vi "MainProgram.vi"(0 "DAQmx Task":refnum<k21>, 1 "BNC Port":refnum<visa-resource-name>, 2 "SRS Port":refnum<visa-resource-name>, 3 "Energy Meter  port":refnum<visa-resource-name>, 4 "SDG II port":refnum<visa-resource-name>, 5 "Mode":T18=enum."GenericTOF", 6 "Micos Port":refnum<visa-resource-name>="COM3", 7 "CommPort (ESP300)":refnum<visa-resource-name>="COM7", 8 "Serial Config (Micos)":T15={"Baud Rate"=115200, "Parity"=0, "Data Bits"=8, "Stop Bits"=10, "Flow Control"=0} {"Flow Control" items=["None", "XON/XOFF", "RTS/CTS", "XON/XOFF & RTS/CTS", "DTR/DSR", "XON/XOFF & DTR/DSR"]; "Stop Bits" items=["1.0"=10, "1.5"=15, "2.0"=20]; "Data Bits" items=["7"=7, "8"=8]; "Parity" items=["None", "Odd", "Even", "Mark", "Space"]; "Baud Rate" items=["300"=300, "600"=600, "1200"=1200, "2400"=2400, "4800"=4800, "9600"=9600, "19200"=19200]}, 9 "Serial Config (ESP300)":T15={"Baud Rate"=19200, "Parity"=0, "Data Bits"=8, "Stop Bits"=10, "Flow Control"=2} {"Flow Control" items=["None", "XON/XOFF", "RTS/CTS", "XON/XOFF & RTS/CTS", "DTR/DSR", "XON/XOFF & DTR/DSR"]; "Stop Bits" items=["1.0"=10, "1.5"=15, "2.0"=20]; "Data Bits" items=["7"=7, "8"=8]; "Parity" items=["None", "Odd", "Even", "Mark", "Space"]; "Baud Rate" items=["300"=300, "600"=600, "1200"=1200, "2400"=2400, "4800"=4800, "9600"=9600, "19200"=19200]}, 10 "#Axis (Micos)":i32=3, 11 "#Axis (ESP300)":i32=3, 12 "Simulation (Micos)":bool=TRUE, 13 "Simulation (ESP300)":bool=TRUE, 14 "MainDAQ_Selector":T16=enum."FakeSignal(Emulator)" caption="Restart Required", 15 "Laser Control Method":T17=enum."SDG_II" caption="Restart Required") -> ()   [LabVIEW 2013]
uses:
  Files/Signal_Segment.ctl
  ControlDef/ProcessingMode.ctl
  ControlDef/Average#.ctl
  ProcessMethods/Binning/BinType.ctl
  ControlDef/MainDAQ_Selector.ctl
  ControlDef/LaserCtrl_Method.ctl
  ControlDef/SpecLengthSelector.ctl
  ControlDef/SampleRateSelector.ctl
  ControlDef/DAQRangeSelector.ctl
  <instrlib>/DG535/Command/DG535_TriggerMode.ctl
  ControlDef/StepWidthSelector.ctl
  ControlDef/Files_Format.ctl
  <instrlib>/DG535/DG535_Configs.ctl
  <instrlib>/DG535/Command/Set Trigger.ctl
  <instrlib>/DG535/Command/Set Delay.ctl
  <instrlib>/DG535/Command/DG535_Channel.ctl
  <instrlib>/DG535/Command/Set Output.ctl
  <instrlib>/DG535/Command/DG535_Output.ctl
  <instrlib>/AnalogDiscSDKLv/VIs/DWF_AnalogIn_Configurations.ctl
  <instrlib>/AnalogDiscSDKLv/VIs/DWF_AcqMode.ctl
  <instrlib>/AnalogDiscSDKLv/VIs/DWF_Filter.ctl
  <instrlib>/AnalogDiscSDKLv/VIs/DWF_TrigSrc.ctl
  <instrlib>/AnalogDiscSDKLv/VIs/DWF_TrigCond.ctl
  <instrlib>/AnalogDiscSDKLv/VIs/DWF_TrigType.ctl
  <instrlib>/GageLv_uic/VI/Gage_Configs.ctl
  ControlDef/InstruMode_Typedef.ctl
  Hardware/BNC(QuantumComposers)/BNC_Configs.ctl
  ControlDef/InstrumentSpecificControls/UIC-AToF/InitializationParams_BNC565_2Ch_AToF.ctl
  Hardware/BNC(QuantumComposers)/Command/Set C-Input.ctl
  Hardware/BNC(QuantumComposers)/Command/Set C-Mode.ctl
  Hardware/BNC(QuantumComposers)/Command/Set C-Output.ctl
  Hardware/BNC(QuantumComposers)/Command/Set C-Enable.ctl
  Hardware/GenericDAQ/VI/GenericDAQ_Configs.ctl
  <vilib>/Utility/error.llb/DialogType.ctl
  ControlDef/AllControlsRefs.ctl
  ControlDef/States-AToF.ctl
  Hardware/FemtoLaser(Legacy)/Laser_Status.ctl
  Files/SaveControlsRef.ctl
  Files/WriterState.ctl
  Hardware/DAQmx(Legacy)/DAQmx_Status.ctl
  Hardware/EPM2000(Legacy)/EPM2K_Status.ctl
  ProcessMethods/SignalAverager/ProcessParams.ctl
  ProcessMethods/SignalAverager/DAQParams.ctl
  ProcessMethods/SignalAverager/DisplayGraph.ctl
  <instrlib>/ESP300/Public/Data/ESP300_State.ctl
  Hardware/BNC(QuantumComposers)/BNC_States.ctl
  <instrlib>/DG535/Command/DG535_States.ctl
  <instrlib>/Micos_uic/Public/Data/Micos_Data.ctl
  ControlDef/QueueRefs.ctl
  <instrlib>/AnalogDiscSDKLv/VIs/DWF_CtrlQueue.ctl
  <instrlib>/AnalogDiscSDKLv/VIs/DWF_State.ctl
  ControlDef/Signal.ctl
  ProcessMethods/SignalAverager/ProcessStates.ctl
  <instrlib>/AnalogDiscSDKLv/VIs/DWF_Signal.ctl
  <instrlib>/AnalogDiscSDKLv/VIs/DWF_PrivateStats.ctl
  <instrlib>/AnalogDiscSDKLv/VIs/DWF_InstrumentStatus.ctl
  <instrlib>/GageLv_uic/VI/Gage_PrivateStats.ctl
  <instrlib>/GageLv_uic/VI/Gage_DAQStatus.ctl
  Apps/GenericUSBCamera/CameraEventTypedef.ctl
  Hardware/Joystick/Joystick_UserEvent.ctl
  Hardware/GenericDAQ/VI/GenericDAQ_PrivateStats.ctl
  Hardware/GenericDAQ/VI/GenericDAQ_Status.ctl
  <instrlib>/GageLv_uic/VI/SetSecondaryDataVIRef_Typedef.ctl
  Files/BinaryHeader.ctl
  Apps/BeamProfiling/BeamProfiling_Params.ctl
  Apps/InstruOptimizer/OptimizerParams.ctl
  Apps/ImagingMS/Imaging_Params.ctl
  <instrlib>/Micos_uic/Public/Data/Micos_State.ctl
  <vilib>/Analysis/baseanly.llb/A x Vector.vi
  ControlDef/QuitProg.vi
  <instrlib>/Micos_uic/Public/Position_Micos.vi
  <instrlib>/ESP300/Public/Position_ESP300.vi
  ControlDef/MiscParams.vi
  ControlDef/PauseMeander.vi
  <userlib>/_OpenG.lib/comparison/comparison.llb/DBL Changed__ogtk.vi
  UI/Autoscale_Y_Single.vi
  <vilib>/Analysis/Matrix/Numeric/Conversions/Array To Matrix - RA2.vi
  <instrlib>/DG535/SRS_DG535_Lib.lvlib
  <instrlib>/ESP300/ESP300.lvlib
  <instrlib>/Micos_uic/Micos_uic.lvlib
  <userlib>/Utility/ErrorLog_lib.lvlib
  Hardware/Signal_Emulator(Legacy)/Emu_CoreDAQ_Globle.vi
  <instrlib>/AnalogDiscSDKLv/AnalogDiscSDKLv.lvlib
  <instrlib>/GageLv_uic/Gage.lvlib
  <vilib>/userdefined/High Color/IMAQdx.ctl
  <vilib>/Analysis/Matrix/NI_Matrix.lvlib
  <vilib>/Analysis/NI_AALBase.lvlib
  Hardware/GenericDAQ/GenericDAQ.lvlib
panel:
  out "Graph (B)":cluster{dbl[], dbl[]}(graph) caption="ChiMS, (C) 2014, Laser Ablation Time-of-Flight Mass Spectrometer with Postionization, under LGPLv3 license, rev.1827"
  in  "Scale(B)Y--":bool caption="AutoScale Y"
  in  "Scale(B)Y++":bool caption="AutoScale Y"
  in  "Binning(B)":bool
  in  "IncrementUpdate(B)":bool=TRUE caption="Increment"
  in  "Scale(B)X++":bool caption="AutoScale X"
  in  "Scale(B)X--":bool caption="AutoScale X"
  in  "Scale(B)_X":bool caption="AutoScale X"
  in  "GraphEnable (B)":bool=TRUE caption="Graph (B)"
  in  "Scale(B)_Y":bool caption="AutoScale Y"
  in  "SW_Average":T1=10 caption="Average" items=["1"=1, "5"=5, "10"=10, "25"=25, "50"=50, "100"=100, "250"=250, "500"=500, "1000"=1000, "2500"=2500, "5000"=5000]
  out "Graph (A)":cluster{dbl[], dbl[]}(graph)
  in  "Scale(A)Y--":bool caption="AutoScale Y"
  in  "Scale(A)Y++":bool caption="AutoScale Y"
  in  "Binning(A)":bool
  in  "IncrementUpdate(A)":bool caption="Increment"
  in  "Scale(A)X++":bool caption="AutoScale X"
  in  "Scale(A)X--":bool caption="AutoScale X"
  in  "Scale(A)_X":bool caption="AutoScale X"
  in  "Scale(A)_Y":bool caption="AutoScale Y"
  in  "GraphEnable (A)":bool=TRUE caption="Graph (A)"
  out "Nd:YAG Energy":dbl(slide) caption="Nd:YAG Energy (J)" scale=0.0..0.03 scale format="%#_2p"
  out "LaserEnergy":dbl(slide) caption="Spitfire Energy (J)" scale=0.0..2e-06 scale format="%#_2p"
  in  "LaserON":bool caption="Spitfire"
  in  "Files Format":T2=enum."Binary Files"
  in  "Snap":bool
  in  "Record":bool
  in  "Signal Segment":T3={"SampleRate"=1000000000.0, "TrigDelay"=0.0, "SpecLength"=512.0, "DAQ_Range"=1000.0, "Average#"=0, "Position"=[], "Spectrum"=[], "Calibr."=[], "Pressure"=-1.0, "Desp_LaserEnergy"=0.0, "PI_LaserEnergy"=0.0, "Voltages Table"=[[0.0, 0.0, 0.0, 0.0]], "ProcMode"=enum."None", "Threshold"=0.005, "Comment"="", "TickCount"=0.0, "Time Stamp"=timestamp(0 s since 1904-01-01)} {"TickCount" format="%#.2f"}
  in  "Setting Panel":T5(tab)=enum."Com.Setup"
  in  "Pause":bool
  in  "StepWidth (Micos)":T6=0.2 caption="StepWidth" items=["0.2 um"=0.0002, "0.001 mm"=0.001, "0.002 mm"=0.002, "0.005 mm "=0.005, "0.01 mm"=0.01, "0.02 mm"=0.02, "0.05 mm"=0.05, "0.1 mm"=0.1, "0.2 mm"=0.2, "1 mm"=1.0]
  in  "SetFocus":bool caption="Go To"
  in  "Focus (-)":bool
  in  "Focus (+)":bool
  in  "Back(+)":bool
  in  "Front(-)":bool
  in  "Back":bool
  in  "Front":bool
  in  "Down(-)":bool
  in  "Right(-)":bool
  in  "Up(+)":bool
  in  "Left(+)":bool
  in  "Right":bool
  in  "Left":bool
  in  "StopMoving":bool
  in  "Up":bool
  in  "Down":bool
  in  "Home(Micos)":bool
  in  "MoveAbs(Micos)":bool caption="Go To"
  in  "Destination":dbl[](array[numeric])=[17.0, 17.0, 24.2] caption="Destination (mm)" min=0.0 max=34.0 format="%#.5f"
  in  "Meander":bool
  in  "Accele.(Micos)":dbl=20.0 caption="Acceleration" format="%#.3f"
  in  "Velocity(Micos)":dbl=10.0 caption="Velocity" format="%#2.3f"
  out "Velcoty_ind_micos":dbl=10.0 caption="Velocity" format="%#_5f"
  out "Accele._ind_micos":dbl=20.0 caption="Acceleration" format="%#_4f"
  out "Position(Micos)":dbl[](array[numeric]) caption="Stage Position (mm)" format="%#.5f"
  in  "DepthProfile":bool
  in  "BeamProfiling(ESP)":bool
  in  "Velocity (ESP) #3":dbl=2.0 caption="Velocity#3" format="%#.3g"
  in  "DelayScan":bool
  in  "MotorDisabled(ESP)":bool
  in  "Meander (ESP)":bool
  in  "Accele. (ESP)":dbl=0.8 caption="Acceleration" format="%#.3g"
  in  "Set dbl pulse Delay":bool
  in  "DP_Delay (ps)":dbl caption="Delay (ps)" min=-3.0 max=300.0 format="%#.3f"
  in  "Down(ESP)":bool
  in  "Up(ESP)":bool
  in  "STOP(ESP)":bool
  in  "Left(ESP)":bool
  in  "Right(ESP)":bool
  in  "Destination(ESP)":dbl[](array[numeric])=[0.0, 0.25, 32.7] caption="Destination" min=0.0 max=360.0 format="%.4f"
  in  "Go(ESP)":bool
  in  "HomeSearch(ESP)":bool
  in  "Velocity (ESP)":dbl=0.2 caption="Velocity" format="%#.3g"
  out "Position(ESP)":dbl[](array[numeric]) caption="Currrent Postion"
  in  "StepWidth (ESP)":T6=0.1 caption="StepWidth (mm)" items=["0.2 um"=0.0002, "0.001 mm"=0.001, "0.002 mm"=0.002, "0.005 mm "=0.005, "0.01 mm"=0.01, "0.02 mm"=0.02, "0.05 mm"=0.05, "0.1 mm"=0.1, "0.2 mm"=0.2, "1 mm"=1.0]
  in  "ZeroDelayPos":dbl=0.679 caption="0 Delay@(mm)" format="%#.3f"
  out "DP_Delay (ps)_indicator":dbl caption="Delay (ps)" min=-3.0 max=300.0 format="%#.3f"
  in  "Delay(PI)":dbl=3e-05 caption="VUV Delay" min=-0.001 max=0.001 step=1e-08 format="%_3ps"
  in  "Delay(LDI-Rej.)":dbl=-2e-06 caption="LDIRej_end" min=-0.001 max=0.0 step=1e-07 format="%_3ps"
  in  "SRS On/Off":bool caption="Dont Rely On\nShowing\nCheck BNC"
  in  "Internal/Burst Rate":dbl=10.0 caption="Internal/Burst Rate (Hz)" min=0.001 max=1000000.0 format="%.3f"
  in  "Trigger Mode (SRS)":T7=enum."External" caption="Trigger Mode"
  in  "Ch_D":dbl=2.8e-05 format="%_3ps"
  in  "Ch_C":dbl format="%_3ps"
  in  "Ch_B":dbl=3e-05 format="%_3ps"
  in  "Ch_A":dbl=0.099807701 format="%_7ps"
  in  "Width B":dbl=1e-06 min=0.0 max=9.9e-05 step=1e-09 format="%_3ps"
  in  "Width A":dbl=1e-06 min=0.0 max=9.9e-05 step=1e-09 format="%_3ps"
  in  "BNC On/Off":bool caption="Dont Rely On\nShowing\nCheck BNC"
  in  "Mode (BNC)":T8(ring)=enum."Single Shot" caption="Mode"
  in  "Channels Enable Status":bool[](array[boolean])=[TRUE, TRUE]
  in  "Set Mode":bool caption="Set BNC"
  in  "Trigger Mode (BNC)":T9(ring)=enum."Triggered" caption="Trigger Mode"
  in  "Rep.Rate (BNC)":dbl=10.0 caption="Repetive Rate" min=0.0 max=1000.0 format="%#_6f Hz"
  in  "Delay B":dbl min=0.0 max=9.9e-05 step=1e-09 format="%_3ps"
  in  "Delay A":dbl format="%_3ps"
  in  "Gain (Voltage Range)":T10=4294966296 items=["-100~900 mV"=4294966296, "-380~20 mV"=4294966895, "-20~380 mV"=4294966896, "+/-5 V"=10000, "+/-2 V"=4000, "+/-1 V"=2000, "+/-500 mV"=1000, "+/-200 mV"=400, "+/-100 mV"=200, "+/-50 mV"=100]
  in  "Spectrum Length":T11=32768.0 items=["256K"=262144.0, "192K"=196608.0, "128K"=131072.0, "96K"=98304.0, "64K"=65280.0, "32K"=32768.0, "24K"=24576.0, "16K"=16384.0, "8K"=8192.0, "1K"=1024.0, "512"=512.0]
  in  "SampleRate":T12=500000000.0 items=["50MS/s"=50000000.0, "100MS/s"=100000000.0, "125MS/s"=125000000.0, "200MS/s"=200000000.0, "250MS/s"=250000000.0, "500MS/s"=500000000.0, "1GS/s"=1000000000.0, "1.6GS/s"=1600000000.0]
  in  "Threshold":dbl=0.01 format="%#_3pV"
  in  "Baseline":dbl
  in  "TopLine":dbl=1.0
  in  "Processing Mode":T4
  in  "ZeroOffsetCorrection":dbl=0.0055 format="%.3p V"
  in  "Resolution(B)":bool
  in  "Resolution(A)":bool
  in  "Cali.":dbl[](array[numeric])=[0.0707, 0.16163, 0.02539] caption="Calibration Params (a, b, c)" format="%#.6f"
  in  "Switch(SDG_II)":bool caption="Status"
  in  "Mode(SDG_II)":bool caption="Mode"
  in  "ManlTrig(SDG)":bool caption="Manual Trigger"
  in  "BinWidth (A)":dbl=0.1
  in  "BinType (A)":T13=enum."ByMass"
  in  "BinWidth (B)":dbl=0.5
  in  "BinType (B)":T13=enum."ByScreen"
  in  "DisplayIncrement":u32=15
  in  "YAGEnergyCoeff.":dbl=132.6
  in  "fsEnergyCoeff.":dbl=1.29
  in  "GenericDAQ_Config":T14={"Acquisition"={"Sample Rate"=1000000000.0, "Mode"=0, "Start (0)"=0.0, "Depth"=1024.0, "Segment"=1}, "Channels"=[{"Range"=1, "DC Offset"=0}], "Mode(Gage)"=enum."Continuous"} {"Acquisition"."Depth" min=256.0 step=128.0; "Acquisition"."Mode" items=["Single", "Dual", "Quad", "Octal"]; "Acquisition"."Sample Rate" format="%.0p"}
  out "Filename Indicator":path caption="Filename"
  in  "ComSettingsTab":enum32{"Micos", "ESP300", "Misc", "Misc 2"}(tab)=enum."ESP300"
  in  "ColdStartReset":bool=TRUE caption="ResetSettings"
  in  "Gage_Config":T19={"Acquisition"={"Sample Rate"=500000000.0, "Mode"=0, "Start (0)"=0.0, "Depth"=32768.0, "Segment Size"=32768.0, "Trigger Delay"=0.0, "Trigger Timeout"=-1.0, "Trigger Holdoff"=0.0, "Clock mode"=enum."Internal", "Segment"=1}, "Channels"=[{"Coupling"=1, "Differential Input"=FALSE, "Direct-to-ADC"=FALSE, "Range"=2000, "Impedance"=50, "DC Offset"=0, "Filter"=0}], "Trigger"={"Slope"=1, "Level"=25, "Source"=0, "External Range"=10000, "External Coupling"=0, "External"=TRUE, "Disable"=FALSE, "External Impedance"=0}, "Mode(Gage)"=enum."Continuous"} {"Trigger"."External Impedance" items=["50 Ohm", "HiZ"]; "Trigger"."External Coupling" items=["DC", "AC"]; "Trigger"."External Range" min=2000 max=10000 step=8000; "Trigger"."Slope" items=["Rising", "Falling"]; "Trigger"."Level" min=-100 max=100; "Trigger"."Source" min=0 max=64 step=1; "Channels"."Impedance" min=50 max=1000000 step=999950; "Channels"."Coupling" items=["DC", "AC"]; "Acquisition"."Segment Size" min=256.0 step=128.0; "Acquisition"."Trigger Delay" min=0.0 step=128.0; "Acquisition"."Trigger Timeout" format="%.0p"; "Acquisition"."Trigger Holdoff" min=0.0 step=128.0; "Acquisition"."Depth" min=256.0 step=128.0; "Acquisition"."Mode" items=["Single", "Dual", "Quad", "Octal"]; "Acquisition"."Sample Rate" format="%.0p"}
  in  "AnalogDisc_Configs":T20={"Acqusition"={"Freq(Hz,SampleRate)"=10000000.0, "BufferSize"=8192, "Mode"=enum."Single", "RecordLength(s)"=8192.0}, "Channels"=[{"Range(V)"=5.0, "Offset(V)"=0.0, "Filter"=enum."Decimate", "Enable"=TRUE}], "Trigger"={"TriggerSource"=enum."None", "Timeout(s)"=0.0, "Holdoff(s)"=1e-06, "Position/Delay(s)"=0.0}, "AnalogTrigger"={"Channel"=0, "Polarity"=enum."Rising", "Type"=enum."Pulse", "Level(V)"=0.0, "Filter"=enum."Decimate", "Hysterisis(V)"=0.0}} {"AnalogTrigger"."Hysterisis(V)" format="%#_6p"; "Acqusition"."RecordLength(s)" format="%#_6p"; "Acqusition"."Freq(Hz,SampleRate)" format="%#_6p"; "Acqusition"."BufferSize" min=1 max=16384 step=1; "Trigger"."Position/Delay(s)" format="%#_6p"; "Trigger"."Holdoff(s)" format="%#_6p"}
  in  "Timing Tab":enum32{"DG535", "BNC"}(tab)
  in  "DG535_Configs":T26={"Trigger"={"Trigger Mode"=enum."External", "Internal/Burst Rate"=10.0, "External  Level"=1.5, "Impedance"=TRUE, "Slope"=FALSE}, "Delays"=[{"Channel"=enum."A Output", "Sync To"=enum."T0 Output", "Delay"=0.099807701}, {"Channel"=enum."B Output", "Sync To"=enum."A Output", "Delay"=1.2e-05}, {"Channel"=enum."C Output", "Sync To"=enum."T0 Output", "Delay"=0.0}, {"Channel"=enum."D Output", "Sync To"=enum."T0 Output", "Delay"=1e-05}, {"Channel"=enum."Trigger Input", "Sync To"=enum."T0 Output", "Delay"=0.0}], "Output"=[{"Channel"=enum."A Output", "Level"=enum."TTL", "Load"=TRUE, "Polarity"=FALSE, "Amplitude"=1.0, "Offset"=0.0}, {"Channel"=enum."B Output", "Level"=enum."TTL", "Load"=FALSE, "Polarity"=TRUE, "Amplitude"=1.0, "Offset"=0.0}, {"Channel"=enum."C Output", "Level"=enum."TTL", "Load"=TRUE, "Polarity"=FALSE, "Amplitude"=1.0, "Offset"=0.0}, {"Channel"=enum."D Output", "Level"=enum."TTL", "Load"=TRUE, "Polarity"=FALSE, "Amplitude"=1.0, "Offset"=0.0}, {"Channel"=enum."T0 Output", "Level"=enum."TTL", "Load"=FALSE, "Polarity"=FALSE, "Amplitude"=1.0, "Offset"=0.0}, {"Channel"=enum."AB Output", "Level"=enum."TTL", "Load"=TRUE, "Polarity"=FALSE, "Amplitude"=1.0, "Offset"=0.0}, {"Channel"=enum."CD Output", "Level"=enum."TTL", "Load"=TRUE, "Polarity"=FALSE, "Amplitude"=1.0, "Offset"=0.0}]} caption="DG535 Settings (Restart Needed)" {"Trigger"."External  Level" min=-2.56 max=2.56 format="%.2f"; "Trigger"."Internal/Burst Rate" min=0.001 max=1000000.0 format="%.3f"; "Delays"."Delay" format="%#_6p"; "Output"."Offset" min=-3.0 max=4.0 format="%.2f"; "Output"."Amplitude" min=-3.0 max=4.0 format="%.2f"}
  in  "BNC_Config":T32={"System"={"Rep.Rate"=1000.0, "Sys Ext Mode"=enum."Triggered", "Mode"=enum."Single Shot"}, "Channels"=[]}
  in  "CameraOn":bool caption="Go To"
  out "Info":string="subProgram Ready..."
  out "Write Counter":i32
  out "Trig. Rate (Hz)":dbl=88.0 caption="DAQ Rate" format="%#.1p"
  out "Moving (Newport)":bool
  out "Moving (Micos)":bool
  in  "Quit":bool
  # "(C) 2014 UIC, Yang Cui, Luke Hanley. Provided AS IS, use at your own risk."
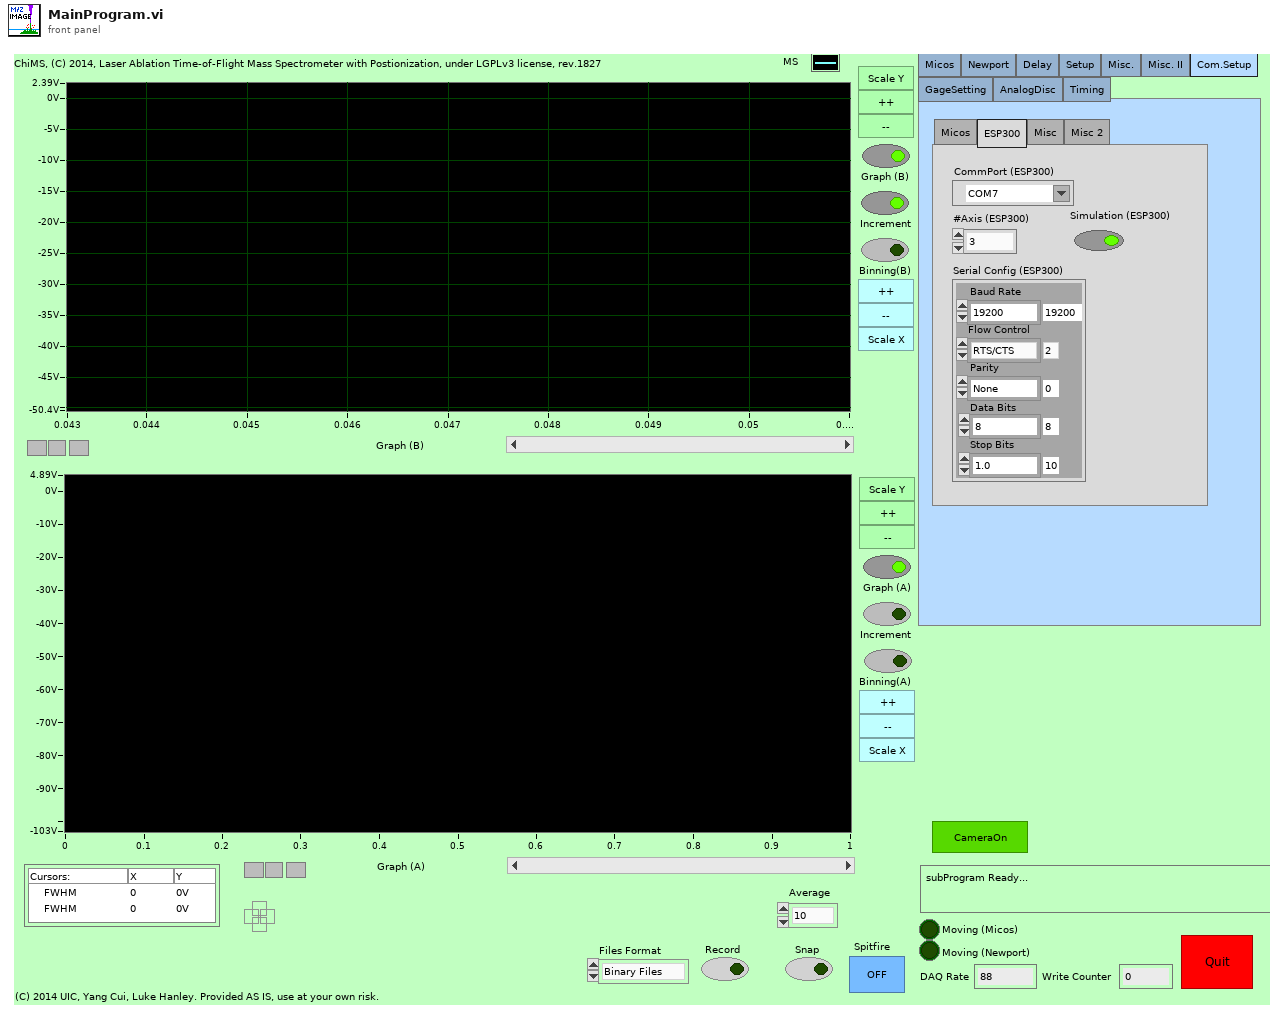
[diagram p1: front panel]
types:
  T1 = typedef "Average#.ctl" = u16
  T2 = typedef "Files_Format.ctl" = enum16{"Text Files", "mzML Files", "Binary Files", "BioMap Files", "imzML Files"}
  T3 = typedef "Signal_Segment.ctl" = cluster{"SampleRate":dbl, "TrigDelay":dbl, "SpecLength":dbl, "DAQ_Range":dbl, "Average#":i32, "Position":dbl[], "Spectrum":sgl[], "Calibr.":dbl[], "Pressure":dbl, "Desp_LaserEnergy":dbl, "PI_LaserEnergy":dbl, "Voltages Table":sgl[][], "ProcMode":T4, "Threshold":dbl, "Comment":string, "TickCount":dbl, "Time Stamp":timestamp}
  T4 = typedef "ProcessingMode.ctl" = enum16{"None", "Drop by Threshold", "TDC Simulate", "SetFilter"}
  T5 = enum32{"Micos", "Newport", "Delay", "Setup", "Misc.", "Misc. II", "Com.Setup", "GageSetting", "AnalogDisc", "Timing"}
  T6 = typedef "StepWidthSelector.ctl" = dbl
  T7 = typedef "SRS_DG535_Lib.lvlib/DG535_TriggerMode.ctl" = enum16{"Internal", "External", "SingleShot", "Burst", "Line"}
  T8 = enum16{"Normal", "Single Shot", "Duty Cycle", "Burst"}
  T9 = enum16{"Disabled", "Triggered", "Gated", "Triggered & Gated"}
  T10 = typedef "DAQRangeSelector.ctl" = u32
  T11 = typedef "SpecLengthSelector.ctl" = dbl
  T12 = typedef "SampleRateSelector.ctl" = dbl
  T13 = typedef "BinType.ctl" = enum16{"ByTime", "ByScreen", "ByMass", "ToUnitMass"}
  T14 = typedef "GenericDAQ.lvlib/GenericDAQ_Configs.ctl" = cluster{"Acquisition":cluster{"Sample Rate":dbl, "Mode":u16, "Start (0)":dbl, "Depth":dbl, "Segment":u32}, "Channels":cluster{"Range":u32, "DC Offset":i32}[], "Mode(Gage)":enum16{"Normal", "Continuous", "MultiRecord", "HwAverage"}}
  T15 = cluster{"Baud Rate":u32, "Parity":u16, "Data Bits":u16, "Stop Bits":u16, "Flow Control":u16}
  T16 = typedef "MainDAQ_Selector.ctl" = enum16{"None", "Gage", "Gage_AdvMultiRec_8bit1Ch", "IonWerks_TDCx4", "Tektronics", "KnifeEdge_Emu", "AnalogDisc", "Gage_AMR_8bit2Ch", "Gage_AMR_16bit1Ch", "Gage_AMR_16bit2Ch", "FakeSignal(Emulator)"}
  T17 = typedef "LaserCtrl_Method.ctl" = enum16{"SRS_DG535", "BNC", "SDG_II"}
  T18 = typedef "InstruMode_Typedef.ctl" = enum16{"fsLDPI", "nsLDPI", "nsLD-fsPI", "GenericTOF", "BeamProfiling"}
  T19 = typedef "Gage.lvlib/Gage_Configs.ctl" = cluster{"Acquisition":cluster{"Sample Rate":dbl, "Mode":u16, "Start (0)":dbl, "Depth":dbl, "Segment Size":dbl, "Trigger Delay":dbl, "Trigger Timeout":dbl, "Trigger Holdoff":dbl, "Clock mode":enum16{"Internal", "External", "Reference"}, "Segment":u32}, "Channels":cluster{"Coupling":u16, "Differential Input":bool, "Direct-to-ADC":bool, "Range":u32, "Impedance":u32, "DC Offset":i32, "Filter":i32}[], "Trigger":cluster{"Slope":u16, "Level":i32, "Source":i32, "External Range":u32, "External Coupling":u16, "External":bool, "Disable":bool, "External Impedance":u16}, "Mode(Gage)":enum16{"Normal", "Continuous", "MultiRecord", "HwAverage"}}
  T20 = typedef "AnalogDiscSDKLv.lvlib/DWF_AnalogIn_Configurations.ctl" = cluster{"Acqusition":cluster{"Freq(Hz,SampleRate)":dbl, "BufferSize":i32, "Mode":T21, "RecordLength(s)":dbl}, "Channels":cluster{"Range(V)":dbl, "Offset(V)":dbl, "Filter":T22, "Enable":bool}[], "Trigger":cluster{"TriggerSource":T23, "Timeout(s)":dbl, "Holdoff(s)":dbl, "Position/Delay(s)":dbl}, "AnalogTrigger":cluster{"Channel":i32, "Polarity":T24, "Type":T25, "Level(V)":dbl, "Filter":T22, "Hysterisis(V)":dbl}}
  T21 = typedef "AnalogDiscSDKLv.lvlib/DWF_AcqMode.ctl" = enum16{"Single", "ScanShift", "ScanScreen", "Record"}
  T22 = typedef "AnalogDiscSDKLv.lvlib/DWF_Filter.ctl" = enum16{"Decimate", "Average", "MinMax"}
  T23 = typedef "AnalogDiscSDKLv.lvlib/DWF_TrigSrc.ctl" = enum16{"None", "PC", "DetectorAnalogIn", "DetectorDigitalIn", "AnalogIn", "DigitalIn", "DigitalOut", "AnalogOut1", "AnalogOut2", "AnalogOut3", "AnalogOut4", "External1", "External2", "External3", "External4"}
  T24 = typedef "AnalogDiscSDKLv.lvlib/DWF_TrigCond.ctl" = enum16{"Rising", "Falling"}
  T25 = typedef "AnalogDiscSDKLv.lvlib/DWF_TrigType.ctl" = enum16{"Edge", "Pulse", "Transition"}
  T26 = typedef "DG535_Configs.ctl" = cluster{"Trigger":T27, "Delays":T28[], "Output":T30[]}
  T27 = typedef "SRS_DG535_Lib.lvlib/Set Trigger.ctl" = cluster{"Trigger Mode":T7, "Internal/Burst Rate":dbl, "External  Level":sgl, "Impedance":bool, "Slope":bool}
  T28 = typedef "SRS_DG535_Lib.lvlib/Set Delay.ctl" = cluster{"Channel":T29, "Sync To":T29, "Delay":dbl}
  T29 = typedef "SRS_DG535_Lib.lvlib/DG535_Channel.ctl" = enum16{"Trigger Input", "T0 Output", "A Output", "B Output", "AB Output", "C Output", "D Output", "CD Output", "NULL"}
  T30 = typedef "SRS_DG535_Lib.lvlib/Set Output.ctl" = cluster{"Channel":T29, "Level":T31, "Load":bool, "Polarity":bool, "Amplitude":dbl, "Offset":dbl}
  T31 = typedef "SRS_DG535_Lib.lvlib/DG535_Output.ctl" = enum16{"TTL", "NIM", "ECL", "Variable"}
  T32 = typedef "BNC_Configs.ctl" = cluster{"System":cluster{"Rep.Rate":dbl, "Sys Ext Mode":enum16{"Disabled", "Triggered", "Gated", "Triggered & Gated"}, "Mode":enum16{"Normal", "Single Shot", "Duty Cycle", "Burst"}}, "Channels":T33[]}
  T33 = typedef "InitializationParams_BNC565_2Ch_AToF.ctl" = cluster{"C-Input":T34, "C-Mode":T35, "C-Output":T36, "C-Enables":T37}
  T34 = typedef "Set C-Input.ctl" = cluster{"Channel":i32, "Sync Source":i32}
  T35 = typedef "Set C-Mode.ctl" = cluster{"Channel":i32, "Delay":dbl, "Width":dbl}
  T36 = typedef "Set C-Output.ctl" = cluster{"Channel":i32, "Polarity":bool}
  T37 = typedef "Set C-Enable.ctl" = cluster{"Channel":i32, "Enable":bool}
  T38 = typedef "AllControlsRefs.ctl" = cluster{"Communication":cluster{"Micos":cluster{"Simulation (Micos)":refnum<vi>, "Micos Port":refnum<vi>, "Serial Config (Micos)":refnum<vi>, "#Axis (Micos)":refnum<vi>}, "ESP300":cluster{"Simulation (ESP300)":refnum<vi>, "CommPort (ESP300)":refnum<vi>, "Serial Config (ESP300)":refnum<vi>, "#Axis (ESP300)":refnum<vi>}, "DAQmx Task":refnum<vi>, "BNC Port":refnum<vi>, "SRS Port":refnum<vi>, "SDG_II port":refnum<vi>, "EnergyMeter port":refnum<vi>}, "Method":cluster{"Mode":refnum<vi>, "MainDAQ_Selector":refnum<vi>, "LaserCtrlMethod":refnum<vi>}, "DG535":cluster{"Delay(PI)":refnum<vi>, "Delay(LDI-Rej.)":refnum<vi>, "Internal/Burst Rate":refnum<vi>, "Trigger Mode (SRS)":refnum<vi>}, "BNC":cluster{"Mode (BNC)":refnum<vi>, "Channels Enable Status":refnum<vi>, "Trigger Mode (BNC)":refnum<vi>, "Rep.Rate (BNC)":refnum<vi>, "Delay A":refnum<vi>, "Width A":refnum<vi>, "Delay B":refnum<vi>, "Width B":refnum<vi>}, "Expt":cluster{"Cali.":refnum<vi>, "Gain (Voltage Range)":refnum<vi>, "Spectrum Length":refnum<vi>, "SampleRate":refnum<vi>, "Processing Mode":refnum<vi>, "Threshold":refnum<vi>, "Baseline":refnum<vi>, "TopLine":refnum<vi>, "ZeroOffsetCorrection":refnum<vi>}, "LowLevel":cluster{"AnalogDisc_Configs":refnum<vi>, "DG535_Configs":refnum<vi>, "Gage_Config":refnum<vi>, "BNC_Config":refnum<vi>}}
  T39 = typedef "DialogType.ctl" = u16
  T40 = cluster{"AnalogDisc_Configs":refnum<vi>, "DG535_Configs":refnum<vi>, "Gage_Config":refnum<vi>, "BNC_Config":refnum<vi>}
  T41 = cluster{"Mode":refnum<vi>, "MainDAQ_Selector":refnum<vi>, "Laser Control Method":refnum<vi>}
  T42 = cluster{"Delay(PI)":refnum<vi>, "Delay(LDI-Rej.)":refnum<vi>, "Internal/Burst Rate":refnum<vi>, "Trigger Mode (SRS)":refnum<vi>}
  T43 = cluster{"Simulation (ESP300)":refnum<vi>, "CommPort (ESP300)":refnum<vi>, "Serial Config (ESP300)":refnum<vi>, "#Axis (ESP300)":refnum<vi>}
  T44 = cluster{"Simulation (Micos)":refnum<vi>, "Micos Port":refnum<vi>, "Serial Config (Micos)":refnum<vi>, "#Axis (Micos)":refnum<vi>}
  T45 = cluster{"Mode (BNC)":refnum<vi>, "Channels Enable Status":refnum<vi>, "Trigger Mode (BNC)":refnum<vi>, "Rep.Rate (BNC)":refnum<vi>, "Delay A":refnum<vi>, "Width A":refnum<vi>, "Delay B":refnum<vi>, "Width B":refnum<vi>}
  T46 = cluster{"Cali.":refnum<vi>, "Gain (Voltage Range)":refnum<vi>, "Spectrum Length":refnum<vi>, "SampleRate":refnum<vi>, "Processing Mode":refnum<vi>, "Threshold":refnum<vi>, "Baseline":refnum<vi>, "TopLine":refnum<vi>, "ZeroOffsetCorrection":refnum<vi>}
  T47 = cluster{cluster{"Simulation (Micos)":refnum<vi>, "Micos Port":refnum<vi>, "Serial Config (Micos)":refnum<vi>, "#Axis (Micos)":refnum<vi>}, cluster{"Simulation (ESP300)":refnum<vi>, "CommPort (ESP300)":refnum<vi>, "Serial Config (ESP300)":refnum<vi>, "#Axis (ESP300)":refnum<vi>}, "DAQmx Task":refnum<vi>, "BNC Port":refnum<vi>, "SRS Port":refnum<vi>, "SDG II port":refnum<vi>, "Energy Meter  port":refnum<vi>}
  T48 = cluster{"Trigger":T27, "Delays":T28[], "Output":T30[]}
  T49 = enum8{"Enabled", "Disabled", "Disabled and Grayed Out"}
  T50 = typedef "InstrumentConfiguration.ctl" = cluster{"Mode":string, "InstrumentMode":cluster{"MainDAQ_Selector":T16, "LaserCtrlMethod":T17, "InstruMode":T18}, "CommuniationSettings":cluster{"SDG_II":refnum<visa-resource-name>, "DG535":refnum<visa-resource-name>, "BNC565":refnum<visa-resource-name>, "EPM2000":refnum<visa-resource-name>, "NI-DAQmx":refnum<visa-resource-name>, "Micos":cluster{"Simulation":bool, "ComPort":refnum<visa-resource-name>, "Serial Config":cluster{"Baud Rate":u32, "Parity":u16, "Data Bits":u16, "Stop Bits":u16, "Flow Control":u16}, "#Axis":i32}, "ESP300":cluster{"Simulation":bool, "ComPort":refnum<visa-resource-name>, "Serial Config":cluster{"Baud Rate":u32, "Parity":u16, "Data Bits":u16, "Stop Bits":u16, "Flow Control":u16}, "#Axis":i32}}, "DG535":cluster{"Trigger":T27, "Delays":T28[], "Output":T30[]}, "Gage_Config":T19, "AnalogDisc_Config":T20, "Micos":cluster{"Velocity":dbl, "Acceleration":dbl}, "ESP300":cluster{"Velocity":dbl[], "Acceleration":dbl[]}, "EPM2000":cluster{"Factor(A)":dbl, "Factor(B)":dbl}, "ProcessMethod":cluster{"TopLine":dbl, "Threshold":dbl, "Baseline":dbl, "ZeroOffset":dbl, "Processing Mode":T4}, "Timing(LDPI)":cluster{"Delay(PI)":dbl, "Delay(Rejection)":dbl, "NoDelayOffset":dbl, "RepRate(Hz)":dbl}, "Cali.":dbl[], "BNC_Config":T32}
  T51 = typedef "GenericDAQ.lvlib/GenericDAQ_PrivateStats.ctl" = cluster{"Model":string, "TrigRate(Hz)":dbl, "TrigCount":i32, "Mode":enum16{"Normal", "Continuous", "MultiRecord", "HwAverage"}, "DAQ_Status":T52, "SecondaryDataVIRef":refnum<vi>, "Option(SecondaryDataVI)":i32, "cSegment":i32}
  T52 = typedef "GenericDAQ.lvlib/GenericDAQ_Status.ctl" = enum16{"Done", "Armed", "Triggered", "Transfering"}
  T53 = typedef "Joystick_UserEvent.ctl" = cluster{"StepMove":refnum<user-event>, "ContMove":refnum<user-event>, "EStop":refnum<user-event>}
  T54 = typedef "CameraEventTypedef.ctl" = cluster{"Command":enum16{"MouseClick", "MouseDoubleClick", "MouseRightClick", "SetCalibration", "AutoCalibration"}, "Params.":variant}
  T55 = typedef "Gage.lvlib/Gage_PrivateStats.ctl" = cluster{"Model":string, "TrigRate(Hz)":dbl, "TrigCount":i32, "Mode(Gage)":enum16{"Normal", "Continuous", "MultiRecord", "HwAverage"}, "Handle":cluster{"Handle":u32, "Sample size":u32, "Resolution":i32, "Offset":i32, "Channels":u32, "Boards":u32}, "DAQ_Status":T56, "SecondaryDataVIRef":refnum<vi>, "Option(SecondaryDataVI)":i32, "cSegment":i32, "TSArray":dbl[], "Adj.SegmenttSize":dbl}
  T56 = typedef "Gage.lvlib/Gage_DAQStatus.ctl" = enum16{"Done", "Armed", "Triggered", "Transfering"}
  T57 = typedef "AnalogDiscSDKLv.lvlib/DWF_PrivateStats.ctl" = cluster{"Handle_DWF":i32, "Model":string, "SN":string, "TrigRate(Hz)":dbl, "TrigCount":i32, "Mode":enum16{"Normal", "Turbo"}, "STS":T58, "SecondaryDataParams.":cluster{"SecondaryDataVIRef.":refnum<vi>, "Option":i32}}
  T58 = typedef "AnalogDiscSDKLv.lvlib/DWF_InstrumentStatus.ctl" = enum16{"stsRdy", "stsARM", "stsDone", "stsTrig", "stsCfg", "stsPrefill", "stsNotDone", "stsTrigDly", "stsError", "stsBusy", "stsStop"}
  T59 = typedef "AnalogDiscSDKLv.lvlib/DWF_Signal.ctl" = cluster{"tickcount":u32, "Signal":sgl[][], "SecondaryData":dbl[], "Flag":enum16{"Normal", "MultiRecStart", "MultiRecEnd", "Reserved1", "Reserved2", "Reserved3"}}
  T60 = typedef "AnalogDiscSDKLv.lvlib/DWF_CtrlQueue.ctl" = cluster{"DWF States":T61, "Variant":variant}
  T61 = typedef "AnalogDiscSDKLv.lvlib/DWF_State.ctl" = enum16{"Enumerate", "Open", "Close", "CloseAll", "Reset", "Quit", "==Settings==", "SetAcquisition_", "SetChannels_", "SetTrigger_", "SetAnalogTrigDetector_", "SetAll_AcquChTrig_", "fConfigurate", "fStart", "GetStatus", "_WaitForDone/Idle", "_GetData", "GetAcquisition", "GetChannels", "GetTrigger", "GetAll_AcquChTrig", "==Messaging==", "_PushDataOut", "GetStat_", "GetConfig_", "==ModeSetup==", "SetSignalBuffer_", "SetMode_", "SetSecondaryDataRef._", "==AnalogOut==", "GetChannelCount_AO", "fStart_AO", "SetChEnable_AO", "SetConfig_AO", "SetFuncData_AO", "SetOffset_AO_", "SetMasterNode_AO", "SetStates_AO", "SetSymetry_AO", "SetTriggerSource_AO", "==Trigger==", "ManualTrigger"}
  T62 = typedef "QueueRefs.ctl" = cluster{"LaserCtrlMethod":T17, "Apps":refnum<queue>, "MainDAQCoreQueue":refnum<queue>, "Micos":refnum<queue>, "ESP300":refnum<queue>, "SMC100":refnum<queue>, "SRS DG535":refnum<queue>, "BNC":refnum<queue>, "SDG_ii":refnum<queue>, "NI-USB_DAQmx":refnum<queue>, "ProcCore_CtrlQueue":refnum<queue>, "WriterCtrl":refnum<queue>, "WriterSIG":refnum<queue>, "Feedback":refnum<queue>, "EPM2000":refnum<queue>, "InfoRef":refnum<vi>, "AppsLock":T63, "ProcCore_SignalQueue":refnum<queue>}
  T63 = typedef "Semaphore RefNum" = refnum<k1>
  T64 = typedef "Micos_uic.lvlib/Micos_Data.ctl" = cluster{"Position":dbl[], "Velocity":dbl[], "Acceleration":dbl[], "Moving":bool, "Simulation":bool, "tickcount_mov":u32, "tickcount_pos":u32, "NumOfAxis":i32, "Initialized":bool, "CommPort":refnum<visa-resource-name>, "Range":dbl[][], "Serial Configuration":cluster{"Baud Rate":u32, "Parity":u16, "Data Bits":u16, "Stop Bits":u16, "Flow Control":u16}, "MotorDisabled":refnum<vi>}
  T65 = typedef "ProcessParams.ctl" = cluster{"DisplayIncrement":u32, "DisplayIncrementRef":refnum<vi>, "Rep .Rate (Hz)":dbl, "Save":bool, "SW_Average":u32, "Filter":T4, "FilterParams":variant, "DAQParams":T66, "Graph":T67[], "CmdParams.":variant, "Average(SW)Ref":refnum<vi>, "Calibr.Params":refnum<vi>, "SignalSegmentRef":refnum<vi>, "WriterQueue":refnum<queue>}
  T66 = typedef "DAQParams.ctl" = cluster{"TrigDelay":dbl, "Offset":i32, "Resolution":i32, "Range (mV)":u32, "Sample Rate":dbl, "Depth":dbl, "Segments":u32}
  T67 = typedef "DisplayGraph.ctl" = cluster{"XY_Graph":refnum<vi>, "Enable":bool, "IncreDisplay":bool, "Binning":bool, "IncremetDisplayRef":refnum<vi>, "PlotDisplayRef":refnum<vi>, "BinningRef":refnum<vi>, "FWHM":bool, "ResoltionRef":refnum<vi>, "BinWidthRef":refnum<vi>, "BinWidth":dbl, "BinTypeRef":refnum<vi>, "BinType":T13}
  T68 = typedef "WriterState.ctl" = cluster{"State":enum16{"Open", "Close", "ChangeFormat", "SetHeader", "QuitProg."}, "Params":variant}
  T69 = typedef "SaveControlsRef.ctl" = cluster{"Write Counter":refnum<vi>, "Segment Counter":refnum<vi>, "Writer error out":refnum<vi>}
  T70 = typedef "Laser_Status.ctl" = cluster{"State":enum16{"Initialize", "Idle/Update", "Configure", "Turn On", "Tun OFF", "Continuous", "Single Shot", "ManualTrigger", "Close", "Quit"}, "Parameter":dbl}
  T71 = typedef "States-AToF.ctl" = enum16{"Initialize", "Idle", "CalcMzArray", "Meander_SGL_MCS", "Meander_MCS", "CleanSurface", "Meander_Npt", "Meander_SGL_Npt", "KnifeEdgeExpt", "KnifeEdgeExpt_Npt", "Imaging_Micos", "Imaging_ESP", "DepthProfiling", "Set_2PulseDelay", "DelayScan", "PeakSearch", "ExportOrigin", "Save Settings", "Load Settings", "Save as Default", "Load Default", "EnergyCalibration", "Quit", "Interrupted_Stop", "Quit_SubProgram", "StepMove_Joystick", "ContMove_Joystick", "Stop_Joystick", "Check_AppsLock", "Return_Status", "DepthProfile_RT", "UpdateInstruStates", "InstruOptimizer_static", "InstruOptimizer_dynamic", "DepthProfiling(3D)"}
  T72 = typedef "SetSecondaryDataVIRef_Typedef.ctl" = cluster{"SecondaryDataVIRef.":refnum<vi>, "Option":i32}
  T73 = cluster{"SecondaryDataVIRef.":refnum<vi>, "Option":i32}
  T74 = typedef "ESP300.lvlib/ESP300_State.ctl" = cluster{"State":enum16{"Initialize", "SetDefaultConfig", "Close", "Quit", "Identify", "MoveAbs", "MoveAbs_all", "MoveRel", "MoveRel_all", "STOP", "Origin/Home", "WaitStop", "QueryStatus", "UpdateXPos", "UpdateAll", "SetVelocity", "SetAcceleration", "ClearErr", "LogMessage", "MotorEnable(1)", "EnableAxis", "JoyStick", "GetVelocity", "GetAcceleration", "SendCmd", "SetSoftLimits", "Beep", "_SettingReturn", "SoftReset"}, "Params.":variant}
  T75 = typedef "Signal.ctl" = cluster{"Command":T76, "Params":variant}
  T76 = typedef "ProcessStates.ctl" = enum16{"Initialize", "Normal", "Display", "Write2Buffer", "CalcMzArray", "StartSave", "StopSave", "ConfigChanged", "EndOfLine", "SetFilterParams", "SetGraphsEnable", "SetAcquisitionParams", "ChangeDisplayIncrement", "ChangeRepRate", "SetWriterRef", "Quit", "StartOfLine"}
  T77 = typedef "BinaryHeader.ctl" = cluster{"Start Position":dbl[], "StepWidth":dbl[], "Dimension":i32[], "SpecLength":i32}
  T78 = typedef "BeamProfiling_Params.ctl" = cluster{"File Header":T77, "w_fit_init.":dbl[], "z0_fit_init.":dbl[], "LowSpeed":dbl, "HighSpeed":dbl, "x/y?":bool, "IncidentAngle":dbl}
  T79 = typedef "OptimizerParams.ctl" = cluster{"File Header":T77, "Instru.Params.":dbl[], "APSO_Params.":dbl[], "LowSpeed":dbl, "HighSpeed":dbl}
  T80 = typedef "Imaging_Params.ctl" = cluster{"File Header":T77, "ScanSpeed":dbl, "HighSpeed":dbl, "SampleRate":T12, "Rep.Rate (Hz)":dbl, "TrigDelay":dbl, "mzCali":dbl[], "KeepStill(ms)":u32, "SaveRaw":bool}
  T81 = cluster{"MotionStageRefs":refnum<queue>, "Axis#":i32, "Delay(ps)":dbl, "ZeroDelay_Offset":dbl}
  T82 = typedef "SRS_DG535_Lib.lvlib/DG535_States.ctl" = cluster{"State":enum16{"Initialize", "Set Trigger", "Set Output", "Set Delay", "Manl_Trig", "Run", "Stop", "Close", "Quit"}, "Para.":variant}
  T83 = typedef "EPM2K_Status.ctl" = cluster{"State":enum16{"Initialize", "Idle/Update", "Configure", "Read", "Close", "Quit"}, "Parameter":dbl}
  T84 = typedef "BNC_States.ctl" = cluster{"State":enum16{"Initialize", "Set System", "Set C-Input", "Set C-Mode", "Set C-Output", "Set C-Enable", "Manl_Trig", "Run", "Stop", "Query C Number", "Close", "Quit"}, "Para.":variant}
  T85 = typedef "DAQmx_Status.ctl" = cluster{"State":enum16{"Initialize", "Idle", "Update", "Close", "Quit"}, "Para.":variant}
  T86 = typedef "Micos_uic.lvlib/Micos_State.ctl" = cluster{"State":enum16{"Initialize", "SetDefaultConfig", "Close", "Quit", "Identify", "MoveAbs", "MoveAbs_all", "MoveRel", "MoveRel_all", "STOP", "Origin/Home", "WaitStop", "QueryStatus", "UpdateXPos", "UpdateAll", "SetVelocity", "SetAcceleration", "ClearErr", "LogMessage", "MotorEnable(1)", "EnableAxis", "JoyStick", "GetVelocity", "GetAcceleration", "SendCmd", "SetSoftLimits", "Beep", "_SettingReturn", "SoftReset"}, "Params.":variant}
  T87 = cluster{"Rep.Rate":dbl, "Sys Ext Mode":enum16{"Disabled", "Triggered", "Gated", "Triggered & Gated"}, "Mode":enum16{"Normal", "Single Shot", "Duty Cycle", "Burst"}}
  T88 = typedef "IMAQdx.ctl" = refnum<k21>
  T89 = cluster{"Coupling":u16, "Differential Input":bool, "Direct-to-ADC":bool, "Range":u32, "Impedance":u32, "DC Offset":i32, "Filter":i32}[]
  T90 = cluster{"Coupling":u16, "Differential Input":bool, "Direct-to-ADC":bool, "Range":u32, "Impedance":u32, "DC Offset":i32, "Filter":i32}
  T91 = cluster{"axes total":u32, "buttons total":u32, "pov total":u32, "device name":string}[]
  T92 = enum16{"MouseClick", "MouseDoubleClick", "MouseRightClick", "SetCalibration", "AutoCalibration"}
  T93 = typedef "NI_Matrix.lvlib/RealMatrix.ctl" = dbl[][]
  T94 = typedef "ImageConvPara.ctl" = cluster{"Start Position":dbl[], "StepWidth":dbl[], "Dimension":i32[], "ScanSpeed":dbl}
  T95 = typedef "ImageConvPara_3d.ctl" = cluster{"Start Position":dbl[], "StepWidth":dbl[], "Dimension":i32[], "MeanderSpeed":dbl}
  T96 = typedef "DepthProfilingParams.ctl" = cluster{"SamplingPos.":cluster{"x":dbl, "y":dbl, "z":dbl}[][], "KeepStill(ms)":u32, "Idle(ms)":u32, "HighSpeed":dbl, "RepRate (Hz)":dbl}
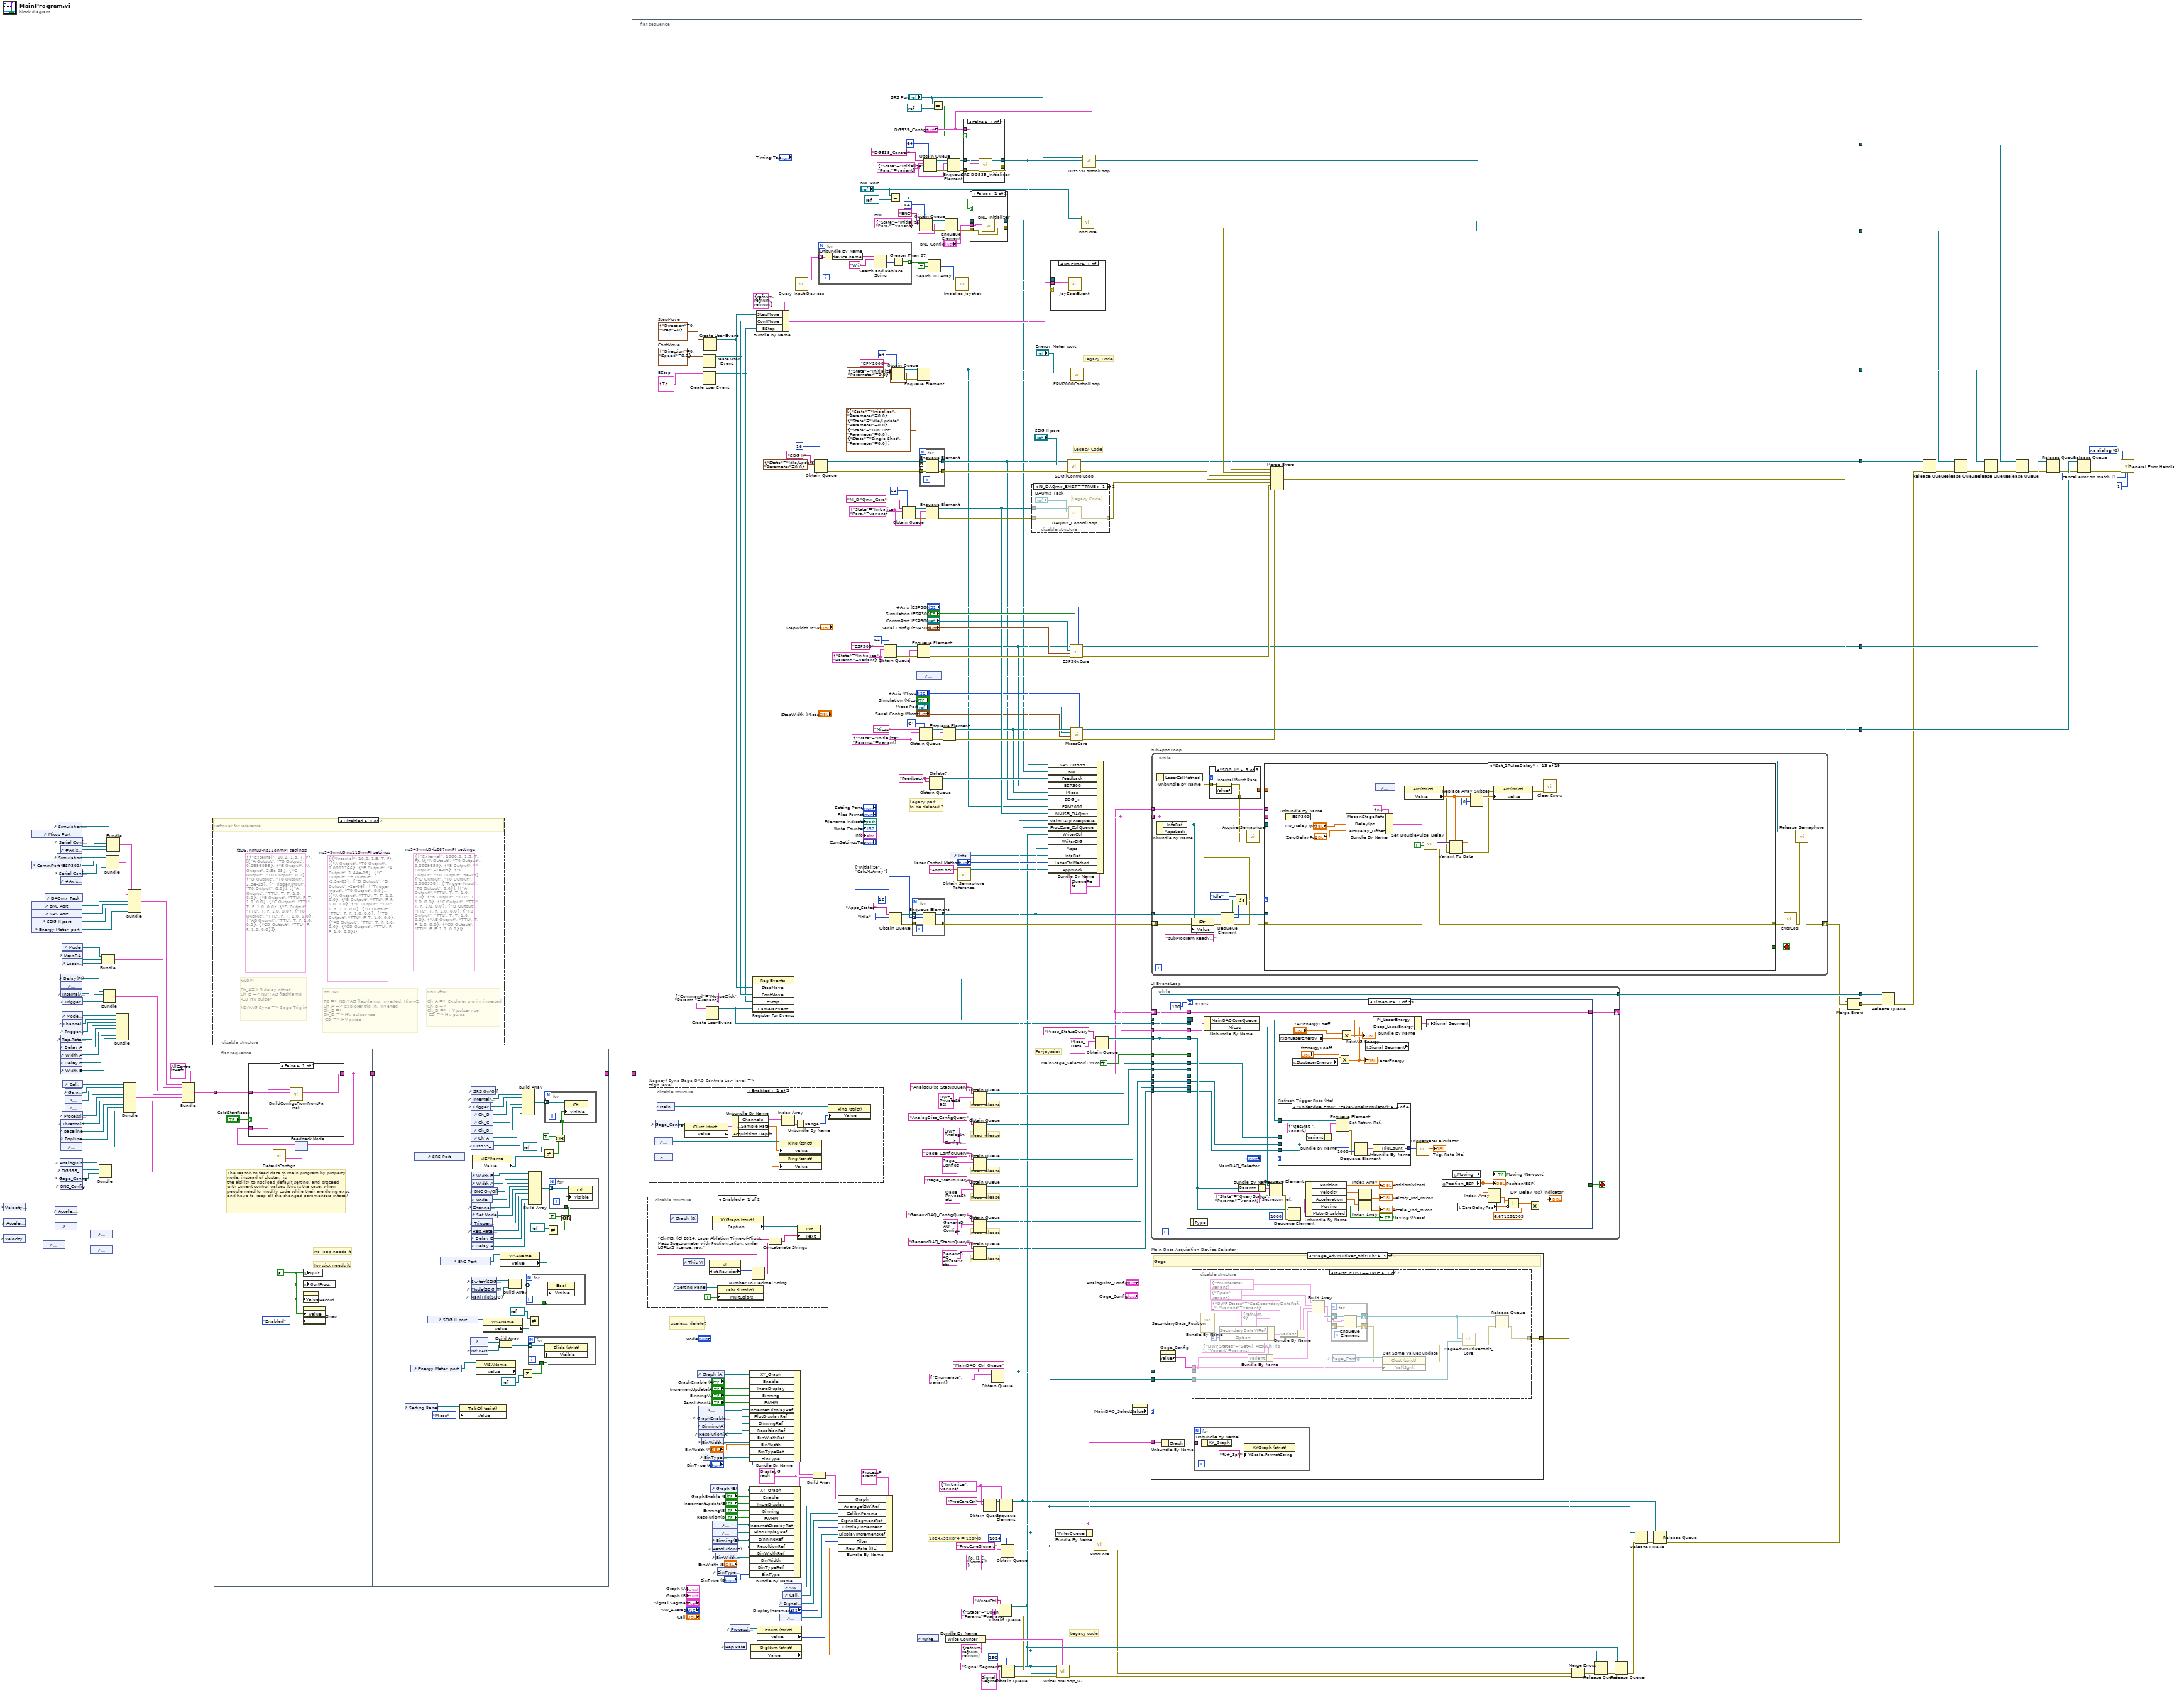
[diagram p0: block diagram]
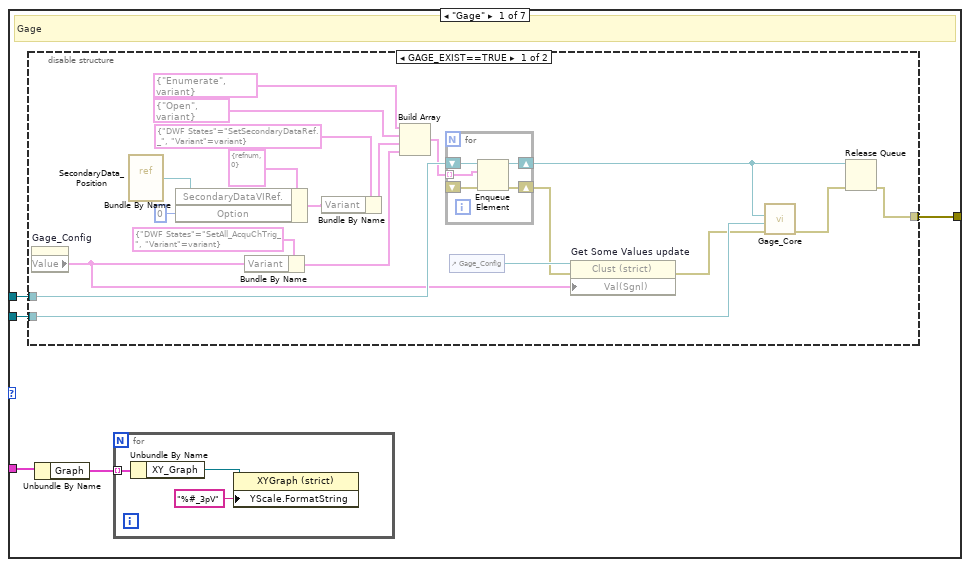
[diagram p8: hidden frame]
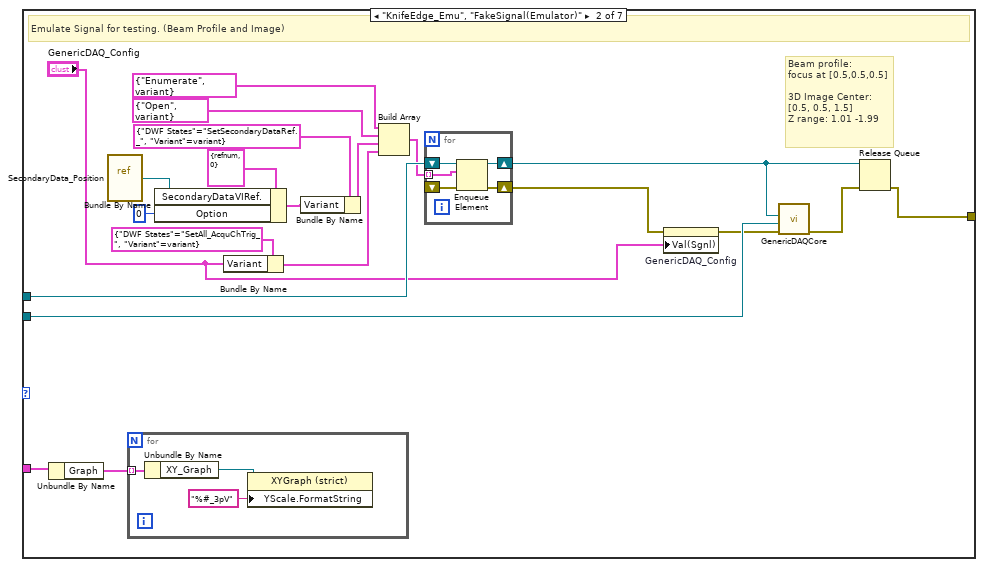
[diagram p10: hidden frame]
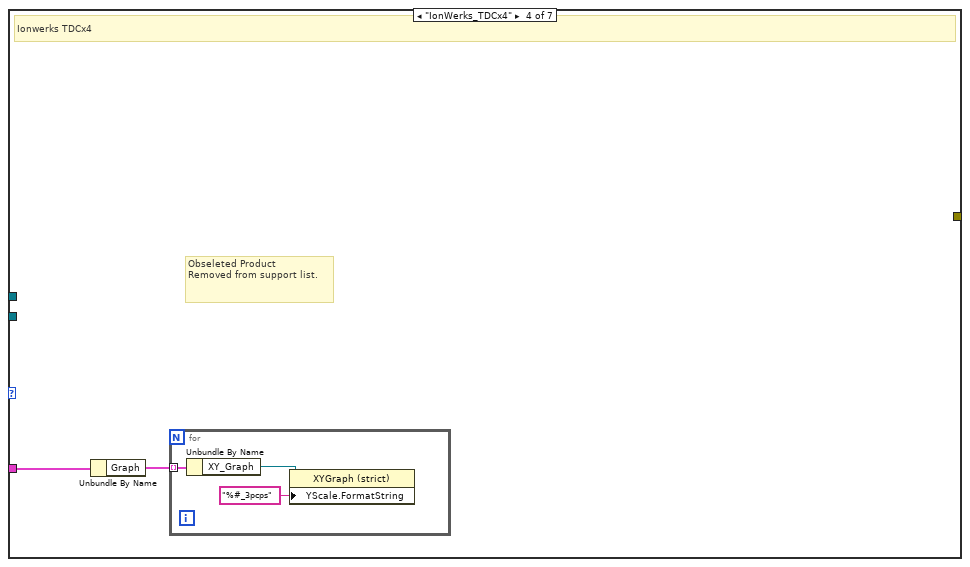
[diagram p12: hidden frame]
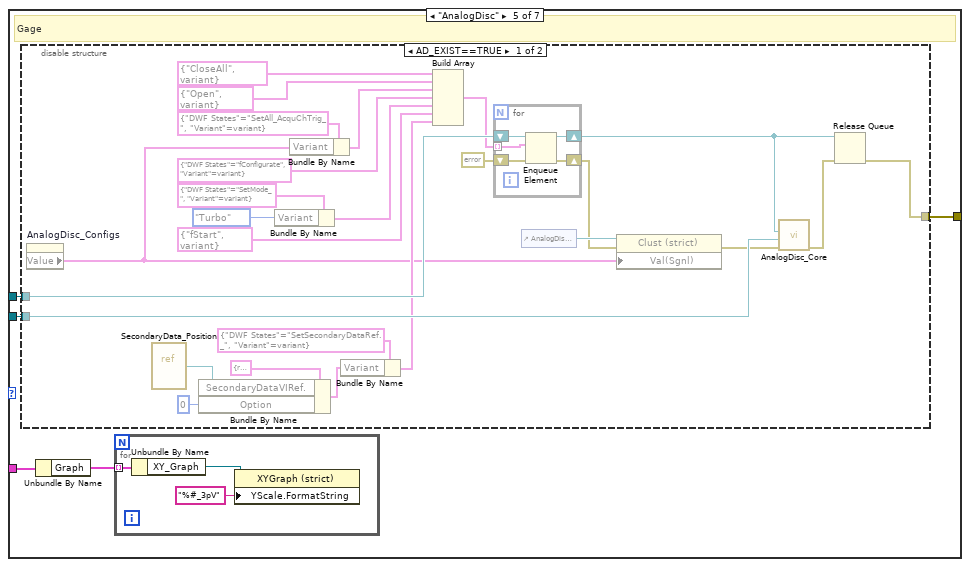
[diagram p13: hidden frame]
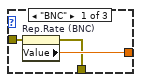
[diagram p17: hidden frame]
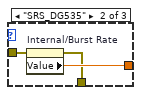
[diagram p18: hidden frame]
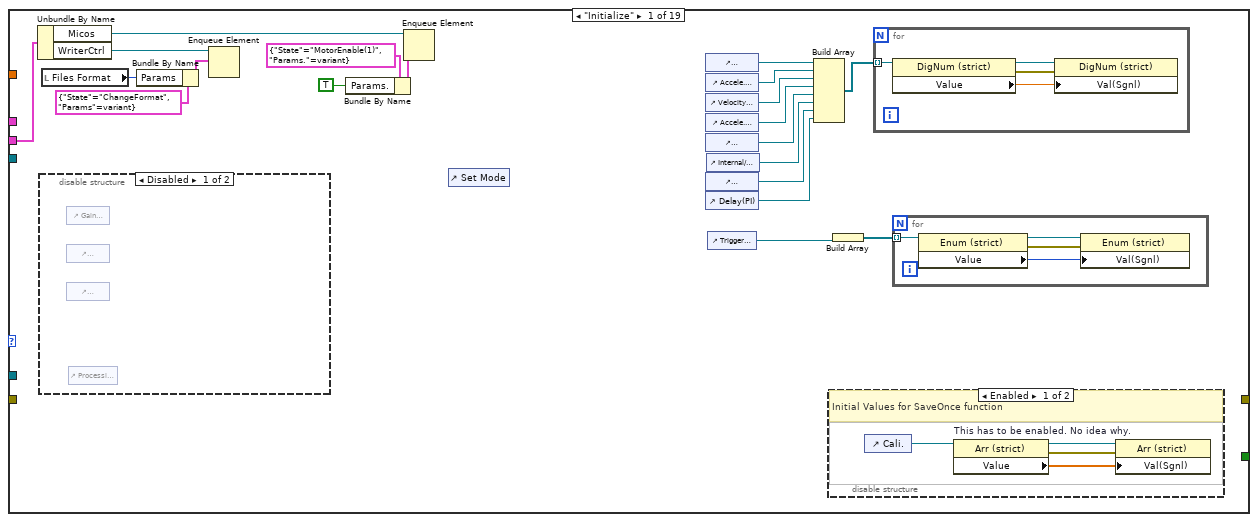
[diagram p19: hidden frame]
diagram:
  w56 = 1 items=["no exception", "cancel error on match", "set error on match"] ("[exception action] (none:0)")
  w57 = T39 0 items=["no dialog", "OK message", "continue or stop message", "OK message + warnings", "continue/stop + warnings"] ("type of dialog (OK msg:1)")
  n1 = control-ref of="Velocity (ESP) #3"() -> ()  [unwired: 1 out]
  n2 = control-ref of="Accele. (ESP)"() -> ()  [unwired: 1 out]
  n3 = control-ref of="Velocity (ESP)"() -> ()  [unwired: 1 out]
  n4 = control-ref of="Micos Port"() -> (w49:refnum<vi>)
  n5 = control-ref of="CommPort (ESP300)"() -> (w52:refnum<vi>)
  n6 = control-ref of="BNC Port"() -> (w45:refnum<vi>)
  n7 = control-ref of="SRS Port"() -> (w44:refnum<vi>)
  n8 = control-ref of="SDG II port"() -> (w42:refnum<vi>)
  n9 = control-ref of="Energy Meter  port"() -> (w43:refnum<vi>)
  n10 = control-ref of="ZeroDelayPos"() -> ()  [unwired: 1 out]
  n11 = control-ref of="DAQmx Task"() -> (w6:refnum<vi>)
  n12 = control-ref of="Accele.(Micos)"() -> ()  [unwired: 1 out]
  n13 = control-ref of="Velocity(Micos)"() -> ()  [unwired: 1 out]
  n14 = control-ref of="Simulation (Micos)"() -> (w47:refnum<vi>)
  n15 = control-ref of="Simulation (ESP300)"() -> (w53:refnum<vi>)
  n16 = control-ref of="Serial Config (Micos)"() -> (w48:refnum<vi>)
  n17 = control-ref of="Serial Config (ESP300)"() -> (w51:refnum<vi>)
  n18 = control-ref of="AnalogDisc_Configs"() -> (w37:refnum<vi>)
  n19 = control-ref of="DG535_Configs"() -> (w38:refnum<vi>)
  n20 = control-ref of="Gage_Config"() -> (w39:refnum<vi>)
  n21 = control-ref of="BNC_Config"() -> (w3:refnum<vi>)
  n22 = control-ref of="#Axis (Micos)"() -> (w46:refnum<vi>)
  n23 = control-ref of="#Axis (ESP300)"() -> (w50:refnum<vi>)
  n24 = control-ref of="Delay(PI)"() -> (w33:refnum<vi>)
  n25 = control-ref of="Delay(LDI-Rej.)"() -> (w32:refnum<vi>)
  n26 = control-ref of="Internal/Burst Rate"() -> (w31:refnum<vi>)
  n27 = control-ref of="Rep.Rate (BNC)"() -> (w27:refnum<vi>)
  n28 = control-ref of="Delay A"() -> (w26:refnum<vi>)
  n29 = control-ref of="Width A"() -> (w25:refnum<vi>)
  n30 = control-ref of="Delay B"() -> (w24:refnum<vi>)
  n31 = control-ref of="Width B"() -> (w23:refnum<vi>)
  n32 = control-ref of="Threshold"() -> (w17:refnum<vi>)
  n33 = control-ref of="Baseline"() -> (w16:refnum<vi>)
  n34 = control-ref of="TopLine"() -> (w15:refnum<vi>)
  n35 = control-ref of="ZeroOffsetCorrection"() -> (w14:refnum<vi>)
  n36 = control-ref of="Mode"() -> (w34:refnum<vi>)
  n37 = control-ref of="MainDAQ_Selector"() -> (w36:refnum<vi>)
  n38 = control-ref of="Laser Control Method"() -> (w35:refnum<vi>)
  n39 = control-ref of="Trigger Mode (SRS)"() -> (w30:refnum<vi>)
  n40 = control-ref of="Mode (BNC)"() -> (w29:refnum<vi>)
  n41 = control-ref of="Trigger Mode (BNC)"() -> (w28:refnum<vi>)
  n42 = control-ref of="Processing Mode"() -> (w18:refnum<vi>)
  n43 = control-ref of="Channels Enable Status"() -> (w1:refnum<vi>)
  n44 = control-ref of="Cali."() -> (w22:refnum<vi>)
  n45 = control-ref of="Gain (Voltage Range)"() -> (w21:refnum<vi>)
  n46 = control-ref of="Spectrum Length"() -> (w20:refnum<vi>)
  n47 = control-ref of="SampleRate"() -> (w19:refnum<vi>)
  n48 = control-ref of="YAGEnergyCoeff."() -> ()  [unwired: 1 out]
  n49 = control-ref of="fsEnergyCoeff."() -> ()  [unwired: 1 out]
  n50 = Bundle("AnalogDisc_Configs"=w37, "DG535_Configs"=w38, "Gage_Config"=w39, "BNC_Config"=w3) -> (w9:T40)  [unwired: 1 in]
  n51 = Bundle("Mode"=w34, "MainDAQ_Selector"=w36, "Laser Control Method"=w35) -> (w13:T41)  [unwired: 1 in]
  n52 = Bundle("Delay(PI)"=w33, "Delay(LDI-Rej.)"=w32, "Internal/Burst Rate"=w31, "Trigger Mode (SRS)"=w30) -> (w12:T42)  [unwired: 1 in]
  n53 = Bundle("Simulation (ESP300)"=w53, "CommPort (ESP300)"=w52, "Serial Config (ESP300)"=w51, "#Axis (ESP300)"=w50) -> (w41:T43)  [unwired: 1 in]
  n54 = Bundle("Simulation (Micos)"=w47, "Micos Port"=w49, "Serial Config (Micos)"=w48, "#Axis (Micos)"=w46) -> (w40:T44)  [unwired: 1 in]
  n55 = Bundle("Mode (BNC)"=w29, "Channels Enable Status"=w1, "Trigger Mode (BNC)"=w28, "Rep.Rate (BNC)"=w27, "Delay A"=w26, "Width A"=w25, "Delay B"=w24, "Width B"=w23) -> (w11:T45)  [unwired: 1 in]
  n56 = Bundle("Cali."=w22, "Gain (Voltage Range)"=w21, "Spectrum Length"=w20, "SampleRate"=w19, "Processing Mode"=w18, "Threshold"=w17, "Baseline"=w16, "TopLine"=w15, "ZeroOffsetCorrection"=w14) -> (w10:T46)  [unwired: 1 in]
  n57 = Bundle(w40, w41, "DAQmx Task"=w6, "BNC Port"=w45, "SRS Port"=w44, "SDG II port"=w42, "Energy Meter  port"=w43) -> (w8:T47)  [unwired: 1 in]
  n58 = Bundle(cluster=T38 {"Communication"={"Micos"={"Simulation (Micos)"=refnum, "Micos Port"=refnum, "Serial Config (Micos)"=refnum, "#Axis (Micos)"=refnum}, "ESP300"={"Simulation (ESP300)"=refnum, "CommPort (ESP300)"=refnum, "Serial Config (ESP300)"=refnum, "#Axis (ESP300)"=refnum}, "DAQmx Task"=refnum, "BNC Port"=refnum, "SRS Port"=refnum, "SDG_II port"=refnum, "EnergyMeter port"=refnum}, "Method"={"Mode"=refnum, "MainDAQ_Selector"=refnum, "LaserCtrlMethod"=refnum}, "DG535"={"Delay(PI)"=refnum, "Delay(LDI-Rej.)"=refnum, "Internal/Burst Rate"=refnum, "Trigger Mode (SRS)"=refnum}, "BNC"={"Mode (BNC)"=refnum, "Channels Enable Status"=refnum, "Trigger Mode (BNC)"=refnum, "Rep.Rate (BNC)"=refnum, "Delay A"=refnum, "Width A"=refnum, "Delay B"=refnum, "Width B"=refnum}, "Expt"={"Cali."=refnum, "Gain (Voltage Range)"=refnum, "Spectrum Length"=refnum, "SampleRate"=refnum, "Processing Mode"=refnum, "Threshold"=refnum, "Baseline"=refnum, "TopLine"=refnum, "ZeroOffsetCorrection"=refnum}, "LowLevel"={"AnalogDisc_Configs"=refnum, "DG535_Configs"=refnum, "Gage_Config"=refnum, "BNC_Config"=refnum}}, "Communication"=w8, "Method"=w13, "DG535"=w12, "BNC"=w11, "Expt"=w10, "LowLevel"=w9) -> (w2:T38)
  n59 = disable-structure shown="Disabled" {
    frame Disabled {
      (unwired) T48 {"Trigger"={"Trigger Mode"=enum."Internal", "Internal/Burst Rate"=10.0, "External  Level"=1.5, "Impedance"=TRUE, "Slope"=FALSE}, "Delays"=[{"Channel"=enum."A Output", "Sync To"=enum."T0 Output", "Delay"=0.0001766}, {"Channel"=enum."B Output", "Sync To"=enum."A Output", "Delay"=1.44e-05}, {"Channel"=enum."C Output", "Sync To"=enum."B Output", "Delay"=-2.5e-05}, {"Channel"=enum."D Output", "Sync To"=enum."B Output", "Delay"=-2e-06}, {"Channel"=enum."Trigger Input", "Sync To"=enum."T0 Output", "Delay"=0.0}], "Output"=[{"Channel"=enum."A Output", "Level"=enum."TTL", "Load"=TRUE, "Polarity"=TRUE, "Amplitude"=1.0, "Offset"=0.0}, {"Channel"=enum."B Output", "Level"=enum."TTL", "Load"=FALSE, "Polarity"=FALSE, "Amplitude"=1.0, "Offset"=0.0}, {"Channel"=enum."C Output", "Level"=enum."TTL", "Load"=TRUE, "Polarity"=FALSE, "Amplitude"=1.0, "Offset"=0.0}, {"Channel"=enum."D Output", "Level"=enum."TTL", "Load"=TRUE, "Polarity"=FALSE, "Amplitude"=1.0, "Offset"=0.0}, {"Channel"=enum."T0 Output", "Level"=enum."TTL", "Load"=FALSE, "Polarity"=TRUE, "Amplitude"=1.0, "Offset"=0.0}, {"Channel"=enum."AB Output", "Level"=enum."TTL", "Load"=TRUE, "Polarity"=FALSE, "Amplitude"=1.0, "Offset"=0.0}, {"Channel"=enum."CD Output", "Level"=enum."TTL", "Load"=FALSE, "Polarity"=FALSE, "Amplitude"=1.0, "Offset"=0.0}]}  # ns349nmLD,ns118nmPI settings
      (unwired) T48 {"Trigger"={"Trigger Mode"=enum."External", "Internal/Burst Rate"=10.0, "External  Level"=1.5, "Impedance"=TRUE, "Slope"=FALSE}, "Delays"=[{"Channel"=enum."A Output", "Sync To"=enum."T0 Output", "Delay"=0.0998095}, {"Channel"=enum."B Output", "Sync To"=enum."A Output", "Delay"=2.5e-05}, {"Channel"=enum."C Output", "Sync To"=enum."T0 Output", "Delay"=0.0}, {"Channel"=enum."D Output", "Sync To"=enum."T0 Output", "Delay"=2.3e-05}, {"Channel"=enum."Trigger Input", "Sync To"=enum."T0 Output", "Delay"=0.0}], "Output"=[{"Channel"=enum."A Output", "Level"=enum."TTL", "Load"=TRUE, "Polarity"=TRUE, "Amplitude"=1.0, "Offset"=0.0}, {"Channel"=enum."B Output", "Level"=enum."TTL", "Load"=FALSE, "Polarity"=TRUE, "Amplitude"=1.0, "Offset"=0.0}, {"Channel"=enum."C Output", "Level"=enum."TTL", "Load"=TRUE, "Polarity"=FALSE, "Amplitude"=1.0, "Offset"=0.0}, {"Channel"=enum."D Output", "Level"=enum."TTL", "Load"=TRUE, "Polarity"=FALSE, "Amplitude"=1.0, "Offset"=0.0}, {"Channel"=enum."T0 Output", "Level"=enum."TTL", "Load"=FALSE, "Polarity"=TRUE, "Amplitude"=1.0, "Offset"=0.0}, {"Channel"=enum."AB Output", "Level"=enum."TTL", "Load"=TRUE, "Polarity"=FALSE, "Amplitude"=1.0, "Offset"=0.0}, {"Channel"=enum."CD Output", "Level"=enum."TTL", "Load"=FALSE, "Polarity"=FALSE, "Amplitude"=1.0, "Offset"=0.0}]}  # fs267nmLD-ns118nmPI settings
      (unwired) T48 {"Trigger"={"Trigger Mode"=enum."External", "Internal/Burst Rate"=1000.0, "External  Level"=1.5, "Impedance"=TRUE, "Slope"=FALSE}, "Delays"=[{"Channel"=enum."A Output", "Sync To"=enum."T0 Output", "Delay"=0.0009859}, {"Channel"=enum."B Output", "Sync To"=enum."A Output", "Delay"=-2e-05}, {"Channel"=enum."C Output", "Sync To"=enum."T0 Output", "Delay"=5e-05}, {"Channel"=enum."D Output", "Sync To"=enum."T0 Output", "Delay"=0.000998}, {"Channel"=enum."Trigger Input", "Sync To"=enum."T0 Output", "Delay"=0.0}], "Output"=[{"Channel"=enum."A Output", "Level"=enum."TTL", "Load"=TRUE, "Polarity"=TRUE, "Amplitude"=1.0, "Offset"=0.0}, {"Channel"=enum."B Output", "Level"=enum."TTL", "Load"=TRUE, "Polarity"=TRUE, "Amplitude"=1.0, "Offset"=0.0}, {"Channel"=enum."C Output", "Level"=enum."TTL", "Load"=TRUE, "Polarity"=FALSE, "Amplitude"=1.0, "Offset"=0.0}, {"Channel"=enum."D Output", "Level"=enum."TTL", "Load"=TRUE, "Polarity"=FALSE, "Amplitude"=1.0, "Offset"=0.0}, {"Channel"=enum."T0 Output", "Level"=enum."TTL", "Load"=TRUE, "Polarity"=TRUE, "Amplitude"=1.0, "Offset"=0.0}, {"Channel"=enum."AB Output", "Level"=enum."TTL", "Load"=TRUE, "Polarity"=FALSE, "Amplitude"=1.0, "Offset"=0.0}, {"Channel"=enum."CD Output", "Level"=enum."TTL", "Load"=FALSE, "Polarity"=FALSE, "Amplitude"=1.0, "Offset"=0.0}]}  # ns349nmLD-fs267nmPI settings
      # "nsLD-fsPI\n\nCh_A => Explorer trig in, inverted\nCh_B => \nCh_D => HV pulser rise\n-CD => HV pulse"
      # "nsLDPI\n\nT0 => ND:YAG flashlamp, inverted, High-Z\nCh_A => Explorer trig in, inverted\nCh_B => \nCh_D => HV pulser rise\n-CD => HV pulse"
      # "fsLDPI\n\nCh_A=> 0 delay offset\nCh_B => ND:YAG flashlamp\n-CD HV pulser\n\nND:YAG Sync => Gage Trig in"
      # "Leftover for reference"
    }
    frame Enabled {
    }
  }
  n60 = flat-sequence {
    tunnel: [w75] -> w5
    tunnel: w2 -> [w72]
    tunnel: [w92] -> w4
    tunnel: w5 -> [w92]
    frame #0 {
      w74 = FALSE
      # "no loop needs it"
      # "Joystick needs it"
      # "The reason to feed data to main program by property \nnode, instead of cluster,  is\nthe ability to not load default setting, and proceed \nwith current control values (this is the case, when \npeople need to modify code while their are doing expt\nand have to keep all the changed paramenters intact.)"
      n61 = call "DefaultConfigs.vi"() -> ("Configuration 2"=w76:T50)  [unwired: 11 in]
      n62 = feedback #1(w76) -> (w77:T50)
      n63 = case shown="False" "ColdStartReset" {
        tunnel: w72 -> [w80 w83]
        tunnel: [w81 w82] -> w75
        tunnel: w77 -> [w79 _]
        frame False {
          n64 = call "BuildConfigsFromFrontPanel.vi"("AllControlsRefs"=w80, "InstruConfig"=w79) -> ("InstruConfig out"=w81:T50)  [unwired: 9 in]
        }
        frame True {
          n65 = call "LoadConfigs_fromFile.vi"() -> ("Configuration"=w82:T50)  [unwired: 11 in]
          n66 = property on="ColdStartReset" class="Bool (strict)"("Value"=FALSE ("ResetSettings")) -> ()  [unwired: 2 in, 2 out]
          n67 = call "InitializeAllConfigs.vi"("AllControlsRefs"=w83, "InstruConfig"=w82) -> ()  [unwired: 10 in]
        }
      }
      n68 = feedback-in #1(w75) -> ()
      n69 = local write "Quit"(w74) -> ()
      n70 = global write "QuitProg.vi" "QuitProg."(w74) -> ()
      n71 = property on="Record" class="Bool (strict)"("Value"=w74) -> ()  [unwired: 2 in, 2 out]
      n72 = property on="Snap" class="Bool (strict)"("Value"=w74, "DisabledEnum"=T49."Enabled" ("Disabled")) -> ()  [unwired: 2 in, 2 out]
    }
    frame #1 {
      n73 = control-ref of="Setting Panel"() -> (w86:refnum<vi>)
      n74 = control-ref of="Energy Meter  port"() -> (w93:refnum<vi>)
      n75 = control-ref of="SRS Port"() -> (w100:refnum<vi>)
      n76 = control-ref of="SDG II port"() -> (w95:refnum<vi>)
      n77 = control-ref of="BNC Port"() -> (w97:refnum<vi>)
      n78 = property class="TabCtl (strict)"(reference=w86, "Value"=T5."Micos") -> ()  [unwired: 1 in, 2 out]
      n79 = control-ref of="LaserEnergy"() -> (w121:refnum<vi>)
      n80 = control-ref of="Nd:YAG Energy"() -> (w122:refnum<vi>)
      n81 = control-ref of="SRS On/Off"() -> (w134:refnum<vi>)
      n82 = control-ref of="Internal/Burst Rate"() -> (w133:refnum<vi>)
      n83 = control-ref of="Trigger Mode (SRS)"() -> (w132:refnum<vi>)
      n84 = control-ref of="Ch_D"() -> (w131:refnum<vi>)
      n85 = control-ref of="Ch_C"() -> (w130:refnum<vi>)
      n86 = control-ref of="Ch_B"() -> (w129:refnum<vi>)
      n87 = control-ref of="Ch_A"() -> (w128:refnum<vi>)
      n88 = control-ref of="DG535_Configs"() -> (w124:refnum<vi>)
      n89 = control-ref of="Switch(SDG_II)"() -> (w113:refnum<vi>)
      n90 = control-ref of="Mode(SDG_II)"() -> (w114:refnum<vi>)
      n91 = control-ref of="ManlTrig(SDG)"() -> (w115:refnum<vi>)
      n92 = control-ref of="Width B"() -> (w101:refnum<vi>)
      n93 = control-ref of="Width A"() -> (w102:refnum<vi>)
      n94 = control-ref of="BNC On/Off"() -> (w103:refnum<vi>)
      n95 = control-ref of="Mode (BNC)"() -> (w104:refnum<vi>)
      n96 = control-ref of="Channels Enable Status"() -> (w105:refnum<vi>)
      n97 = control-ref of="Set Mode"() -> (w106:refnum<vi>)
      n98 = control-ref of="Trigger Mode (BNC)"() -> (w107:refnum<vi>)
      n99 = control-ref of="Rep.Rate (BNC)"() -> (w108:refnum<vi>)
      n100 = control-ref of="Delay B"() -> (w109:refnum<vi>)
      n101 = control-ref of="Delay A"() -> (w110:refnum<vi>)
      n102 = property class="VISAName"(reference=w100) -> ("Value"=w99:refnum<visa-resource-name>)  [unwired: 1 in, 2 out]
      n103 = property class="VISAName"(reference=w93) -> ("Value"=w94:refnum<visa-resource-name>)  [unwired: 1 in, 2 out]
      n104 = property class="VISAName"(reference=w95) -> ("Value"=w96:refnum<visa-resource-name>)  [unwired: 1 in, 2 out]
      n105 = Build Array(w121, w122) -> (w123:refnum<vi>[])
      n106 = property class="VISAName"(reference=w97) -> ("Value"=w98:refnum<visa-resource-name>)  [unwired: 1 in, 2 out]
      n107 = Build Array(w113, w114, w115) -> (w118:refnum<vi>[])
      n108 = Not Equal?(x=w94, y=refnum<visa-resource-name> refnum ("BNC Port")) -> (x != y?=w119:bool)
      n109 = Build Array(w134, w133, w132, w131, w130, w129, w128, w124) -> (w125:refnum<vi>[])
      n110 = Not Equal?(x=refnum<visa-resource-name> refnum ("BNC Port"), y=w96) -> (x != y?=w116:bool)
      n111 = for {
        tunnel: w118 -> [w138] mode=indexing
        tunnel: w116 -> [w137]
        n112 = property class="Bool"(reference=w138, "Visible"=w137) -> ()  [unwired: 1 in, 2 out]
      }
      n113 = Build Array(w101, w102, w103, w104, w105, w106, w107, w108, w109, w110) -> (w111:refnum<vi>[])
      n114 = for {
        tunnel: w123 -> [w136] mode=indexing
        tunnel: w119 -> [w135]
        n115 = property class="Slide (strict)"(reference=w136, "Visible"=w135) -> ()  [unwired: 1 in, 2 out]
      }
      n116 = Not Equal?(x=refnum<visa-resource-name> refnum ("BNC Port"), y=w99) -> (x != y?=w127:bool)
      n117 = Not Equal?(x=refnum<visa-resource-name> refnum ("BNC Port"), y=w98) -> (x != y?=w91:bool)
      n118 = Or(x=TRUE, y=w127) -> (x .or. y?=w88:bool)
      n119 = for {
        tunnel: w125 -> [w142] mode=indexing
        tunnel: w88 -> [w141]
        n120 = property class="Ctl"(reference=w142, "Visible"=w141) -> ()  [unwired: 1 in, 2 out]
      }
      n121 = Or(x=TRUE, y=w91) -> (x .or. y?=w90:bool)
      n122 = for {
        tunnel: w111 -> [w140] mode=indexing
        tunnel: w90 -> [w139]
        n123 = property class="Ctl"(reference=w140, "Visible"=w139) -> ()  [unwired: 1 in, 2 out]
      }
    }
  }
  n124 = flat-sequence {
    tunnel: [w234] -> w71
    tunnel: [w221] -> w70
    tunnel: [w219] -> w68
    tunnel: [w217] -> w67
    tunnel: [w216] -> w66
    tunnel: [w215] -> w64
    tunnel: [w214] -> w62
    tunnel: [w213] -> w61
    tunnel: w4 -> [w158]
    frame #0 {
      w157 = T75 {"Command"=enum."Initialize", "Params"=variant} ("element")
      w198 = cluster{"EStop":bool} {"EStop"=TRUE}  # EStop
      w203 = cluster{"Direction":i32, "Speed":dbl} {"Direction"=0, "Speed"=0.0}  # ContMove
      w204 = cluster{"Direction":i32, "Step":i32} {"Direction"=0, "Step"=0}  # StepMove
      w205 = TRUE  # MainStage_Selector(T:Micos)
      w280 = T67 {"XY_Graph"=refnum, "Enable"=FALSE, "IncreDisplay"=FALSE, "Binning"=FALSE, "IncremetDisplayRef"=refnum, "PlotDisplayRef"=refnum, "BinningRef"=refnum, "FWHM"=FALSE, "ResoltionRef"=refnum, "BinWidthRef"=refnum, "BinWidth"=0.0, "BinTypeRef"=refnum, "BinType"=enum."ByTime"} ("Graph")
      w243 = T74 {"State"=enum."Initialize", "Params."=variant} ("Cluster")
      w248 = T82 {"State"=enum."Initialize", "Para."=variant} ("element")
      w256 = T84 {"State"=enum."Initialize", "Para."=variant}  # BNC
      w285 = T74 {"State"=enum."Initialize", "Params."=variant} ("Cluster")
      w323 = T83 {"State"=enum."Initialize", "Parameter"=0.0} ("Idle")
      w328 = T85 {"State"=enum."Initialize", "Para."=variant} ("Micos States")
      w350 = "Feedback"
      w358 = T71[] [enum."Initialize", enum."CalcMzArray"] items=["Initialize", "Idle", "CalcMzArray", "Meander_SGL_MCS", "Meander_MCS", "CleanSurface", "Meander_Npt", "Meander_SGL_Npt", "KnifeEdgeExpt", "KnifeEdgeExpt_Npt", "Imaging_Micos", "Imaging_ESP", "DepthProfiling", "Set_2PulseDelay", "DelayScan", "PeakSearch", "ExportOrigin", "Save Settings", "Load Settings", "Save as Default", "Load Default", "EnergyCalibration", "Quit", "Interrupted_Stop", "Quit_SubProgram", "StepMove_Joystick", "ContMove_Joystick", "Stop_Joystick", "Check_AppsLock", "Return_Status", "DepthProfile_RT", "UpdateInstruStates", "InstruOptimizer_static", "InstruOptimizer_dynamic", "DepthProfiling(3D)"]
      # "need release"
      # "need release"
      # "useless, delete?"
      # "For joystick"
      # "Legacy part\nto be deleted ?"
      # "Legacy Code"
      # "Legacy Code"
      # "Legacy code"
      # "need release"
      # "need release"
      # "need release"
      # "need release"
      # "1024x32KB*4 = 128MB"
      n125 = disable-structure shown="Enabled" {
        frame Enabled {
          n126 = control-ref of="Graph (B)"() -> (w371:refnum<vi>)
          n127 = control-ref of="Setting Panel"() -> (w378:refnum<vi>)
          n128 = control-ref of="This VI"() -> (w376:refnum<vi>)
          n129 = property class="VI"(reference=w376) -> ("Hist.Revision"=w373:u32)  [unwired: 1 in, 2 out]
          n130 = property class="XYGraph (strict)"(reference=w371) -> ("Caption"=w370:refnum<vi>)  [unwired: 1 in, 2 out]
          n131 = property class="TabCtl (strict)"(reference=w378, "MultColors"=TRUE ("Allow Multiple Colors")) -> ()  [unwired: 1 in, 2 out]
          n132 = Number To Decimal String(number=w373) -> (decimal integer string=w372:string)  [unwired: 1 in]
          n133 = Concatenate Strings("ChiMS, (C) 2014, Laser Ablation Time-of-Flight Mass Spectrometer with Postionization, under LGPLv3 license, rev." ("string"), w372) -> (w375:string)
          n134 = property class="Txt"(reference=w370, "Text"=w375) -> ()  [unwired: 1 in, 2 out]
        }
        frame Disabled {
        }
      }
      n135 = disable-structure "(Legacy) Sync Gage DAQ Controls Low level =>  High level" shown="Enabled" {
        frame Enabled {
          n136 = control-ref of="SampleRate"() -> (w386:refnum<vi>)
          n137 = control-ref of="Spectrum Length"() -> (w388:refnum<vi>)
          n138 = control-ref of="Gage_Config"() -> (w384:refnum<vi>)
          n139 = control-ref of="Gain (Voltage Range)"() -> (w387:refnum<vi>)
          n140 = property class="Clust (strict)"(reference=w384) -> ("Value"=w385:T19)  [unwired: 1 in, 2 out]
          n141 = Unbundle By Name(w385) -> ("Channels"=w381:T89, "Acquisition.Sample Rate"=w383:dbl, "Acquisition.Depth"=w382:dbl)
          n142 = property class="Ring (strict)"(reference=w386, "Value"=w383) -> ()  [unwired: 1 in, 2 out]
          n143 = property class="Ring (strict)"(reference=w388, "Value"=w382) -> ()  [unwired: 1 in, 2 out]
          n144 = Index Array(array=w381) -> (element=w380:T90)  [unwired: 1 in]
          n145 = Unbundle By Name(w380) -> ("Range"=w379:u32)
          n146 = property class="Ring (strict)"(reference=w387, "Value"=w379) -> ()  [unwired: 1 in, 2 out]
        }
        frame Disabled {
        }
      }
      n147 = control-ref of="Graph (A)"() -> (w314:refnum<vi>)
      n148 = control-ref of="IncrementUpdate(A)"() -> (w306:refnum<vi>)
      n149 = control-ref of="GraphEnable (A)"() -> (w305:refnum<vi>)
      n150 = control-ref of="Binning(A)"() -> (w304:refnum<vi>)
      n151 = control-ref of="Resolution(A)"() -> (w291:refnum<vi>)
      n152 = control-ref of="BinWidth (A)"() -> (w284:refnum<vi>)
      n153 = Create User Event(user event datatype=w203) -> (user event=w201:refnum<user-event>)  [unwired: 1 in, 1 out]
      n154 = Create User Event(user event datatype=w198) -> (user event=w197:refnum<user-event>)  [unwired: 1 in, 1 out]
      n155 = control-ref of="BinType (A)"() -> (w282:refnum<vi>)
      n156 = Create User Event(user event datatype=w204) -> (user event=w202:refnum<user-event>)  [unwired: 1 in, 1 out]
      n157 = Create User Event(user event datatype=T54 {"Command"=enum."MouseClick", "Params."=variant} ("CameraEvent")) -> (user event=w159:refnum<user-event>)  [unwired: 1 in, 1 out]
      n158 = control-ref of="Graph (B)"() -> (w313:refnum<vi>)
      n159 = control-ref of="IncrementUpdate(B)"() -> (w300:refnum<vi>)
      n160 = control-ref of="GraphEnable(B)"() -> (w299:refnum<vi>)
      n161 = control-ref of="Binning(B)"() -> (w298:refnum<vi>)
      n162 = control-ref of="Resolution(B)"() -> (w290:refnum<vi>)
      n163 = control-ref of="BinWidth (B)"() -> (w279:refnum<vi>)
      n164 = control-ref of="BinType (B)"() -> (w277:refnum<vi>)
      n165 = control-ref of="Rep.Rate (BNC)"() -> (w266:refnum<vi>)
      n166 = control-ref of="Processing Mode"() -> (w275:refnum<vi>)
      n167 = Bundle By Name(cluster=w280, "XY_Graph"=w314, "Enable"="GraphEnable (A)", "IncreDisplay"="IncrementUpdate(A)", "Binning"="Binning(A)", "FWHM"="Resolution(A)", "IncremetDisplayRef"=w306, "PlotDisplayRef"=w305, "BinningRef"=w304, "ResoltionRef"=w291, "BinWidthRef"=w284, "BinWidth"="BinWidth (A)", "BinTypeRef"=w282, "BinType"="BinType (A)") -> (w312:T67)
      n168 = Bundle By Name(cluster=w280, "XY_Graph"=w313, "Enable"="GraphEnable (B)", "IncreDisplay"="IncrementUpdate(B)", "Binning"="Binning(B)", "FWHM"="Resolution(B)", "IncremetDisplayRef"=w300, "PlotDisplayRef"=w299, "BinningRef"=w298, "ResoltionRef"=w290, "BinWidthRef"=w279, "BinWidth"="BinWidth (B)", "BinTypeRef"=w277, "BinType"="BinType (B)") -> (w311:T67)
      n169 = property class="DigNum (strict)"(reference=w266) -> ("Value"=w265:dbl)  [unwired: 1 in, 2 out]
      n170 = register-events(w202, w201, w197, w159) -> (reference out=w294:refnum<event-registration>)  [unwired: 2 in, 1 out]
      n171 = Bundle By Name(cluster=T53 {"StepMove"=refnum, "ContMove"=refnum, "EStop"=refnum}, "StepMove"=w202, "ContMove"=w201, "EStop"=w197) -> (w200:T53)
      n172 = property class="Enum (strict)"(reference=w275) -> ("Value"=w274:T4)  [unwired: 1 in, 2 out]
      n173 = control-ref of="Signal Segment"() -> (w295:refnum<vi>)
      n174 = control-ref of="DisplayIncrement"() -> (w264:refnum<vi>)
      n175 = control-ref of="Cali."() -> (w296:refnum<vi>)
      n176 = control-ref of="SW Average"() -> (w297:refnum<vi>)
      n177 = call <vilib>:"Query Input Devices.vi"() -> ("error out"=w322:errorcluster, "joystick info"=w193:T91)  [unwired: 8 in, 2 out]
      n178 = Build Array(w312, w311) -> (w310:T67[])
      n179 = Obtain Queue(max queue size (-1, unlimited)=16, name (unnamed)="SDG II", element data type=T70 {"State"=enum."Idle/Update", "Parameter"=0.0} ("Cluster")) -> (queue out=w346:refnum<queue>, error out=w347:errorcluster)  [unwired: 2 in, 1 out]
      n180 = for {
        tunnel: w193 -> [w402] mode=indexing
        tunnel: [w398] -> w196 mode=indexing
        n181 = Unbundle By Name(w402) -> ("device name"=w401:string)
        n182 = Search and Replace String(input string=w401, search string="Wii") -> (number of replacements=w399:i32)  [unwired: 6 in, 3 out]
        n183 = Greater Than 0?(x=w399) -> (x > 0?=w398:bool)
      }
      n184 = Bundle By Name(cluster=T65 {"DisplayIncrement"=0, "DisplayIncrementRef"=refnum, "Rep .Rate (Hz)"=0.0, "Save"=FALSE, "SW_Average"=0, "Filter"=enum."None", "FilterParams"=variant, "DAQParams"={"TrigDelay"=0.0, "Offset"=0, "Resolution"=0, "Range (mV)"=0, "Sample Rate"=0.0, "Depth"=0.0, "Segments"=0}, "Graph"=[], "CmdParams."=variant, "Average(SW)Ref"=refnum, "Calibr.Params"=refnum, "SignalSegmentRef"=refnum, "WriterQueue"=refnum}, "Graph"=w310, "Average(SW)Ref"=w297, "Calibr.Params"=w296, "SignalSegmentRef"=w295, "DisplayIncrement"="DisplayIncrement", "DisplayIncrementRef"=w264, "Filter"=w274, "Rep .Rate (Hz)"=w265) -> (w262:T65)
      n185 = Obtain Queue(max queue size (-1, unlimited)=64, name (unnamed)="ESP300", element data type=w285) -> (queue out=w348:refnum<queue>, error out=w349:errorcluster)  [unwired: 2 in, 1 out]
      n186 = Obtain Queue(max queue size (-1, unlimited)=16, name (unnamed)="Apps_States", element data type=States-AToF."Idle" ("Ring")) -> (queue out=w362:refnum<queue>, error out=w361:errorcluster)  [unwired: 2 in, 1 out]
      n187 = Equal?(x="BNC Port", y=refnum<visa-resource-name> refnum ("SRS Port")) -> (x = y?=w152:bool)
      n188 = Obtain Queue(max queue size (-1, unlimited)=64, name (unnamed)="EPM2000", element data type=w323) -> (queue out=w325:refnum<queue>, error out=w324:errorcluster)  [unwired: 2 in, 1 out]
      n189 = Obtain Queue(max queue size (-1, unlimited)=64, name (unnamed)="NI_DAQmx_Core", element data type=w328) -> (queue out=w329:refnum<queue>, error out=w331:errorcluster)  [unwired: 2 in, 1 out]
      n190 = for {
        tunnel: w362 -> [w1138]
        tunnel: w361 -> [w1137]
        tunnel: [w1136] -> w269
        tunnel: [w1135] -> w351
        tunnel: w358 -> [w1134] mode=indexing
        n191 = Enqueue Element(queue=w1138, element=w1134, error in (no error)=w1137) -> (queue out=w1136:refnum<queue>, error out=w1135:errorcluster)  [unwired: 1 in, 1 out]
      }
      n192 = control-ref of="MotorDisabled(ESP)"() -> (w260:refnum<vi>)
      n193 = control-ref of="Write Counter"() -> (w336:refnum<vi>)
      n194 = Enqueue Element(queue=w325, element=w323, error in (no error)=w324) -> (queue out=w218:refnum<queue>, error out=w327:errorcluster)  [unwired: 1 in, 1 out]
      n195 = Enqueue Element(queue=w348, element=w285, error in (no error)=w349) -> (queue out=w244:refnum<queue>, error out=w340:errorcluster)  [unwired: 1 in, 1 out]
      n196 = Obtain Queue(max queue size (-1, unlimited)=64, name (unnamed)="BNC", element data type=w256) -> (queue out=w258:refnum<queue>, error out=w259:errorcluster)  [unwired: 2 in, 1 out]
      n197 = Obtain Queue(max queue size (-1, unlimited)=64, name (unnamed)="Micos", element data type=w243) -> (queue out=w359:refnum<queue>, error out=w360:errorcluster)  [unwired: 2 in, 1 out]
      n198 = for {
        tunnel: [w554] -> w341
        tunnel: w347 -> [w553]
        tunnel: w346 -> [w552]
        tunnel: [w551] -> w220
        tunnel: T70[] [{"State"=enum."Initialize", "Parameter"=0.0}, {"State"=enum."Idle/Update", "Parameter"=0.0}, {"State"=enum."Tun OFF", "Parameter"=0.0}, {"State"=enum."Single Shot", "Parameter"=0.0}] -> [w550] mode=indexing
        n199 = Enqueue Element(queue=w552, element=w550, error in (no error)=w553) -> (queue out=w551:refnum<queue>, error out=w554:errorcluster)  [unwired: 1 in, 1 out]
      }
      n200 = Obtain Queue(max queue size (-1, unlimited)=64, name (unnamed)="DG535_Control", element data type=w248) -> (queue out=w247:refnum<queue>, error out=w250:errorcluster)  [unwired: 2 in, 1 out]
      n201 = Enqueue Element(queue=w329, element=w328, error in (no error)=w331) -> (queue out=w271:refnum<queue>, error out=w330:errorcluster)  [unwired: 1 in, 1 out]
      n202 = Search 1D Array(1D array=w196, element=TRUE) -> (index of element=w194:i32)  [unwired: 1 in]
      n203 = Obtain Queue "Delete?"(name (unnamed)=w350, element data type=w350) -> (queue out=w272:refnum<queue>)  [unwired: 3 in, 2 out]
      n204 = Equal?(x="SRS Port", y=refnum<visa-resource-name> refnum ("SRS Port")) -> (x = y?=w231:bool)
      n205 = Enqueue Element(queue=w359, element=w243, error in (no error)=w360) -> (queue out=w242:refnum<queue>, error out=w339:errorcluster)  [unwired: 1 in, 1 out]
      n206 = Enqueue Element(queue=w258, element=w256, error in (no error)=w259) -> (queue out=w156:refnum<queue>, error out=w150:errorcluster)  [unwired: 1 in, 1 out]
      n207 = Bundle By Name(cluster=T69 {"Write Counter"=refnum, "Segment Counter"=refnum, "Writer error out"=refnum} ("Controls ref."), "Write Counter"=w336) -> (w337:T69)
      n208 = Enqueue Element(queue=w247, element=w248, error in (no error)=w250) -> (queue out=w246:refnum<queue>, error out=w249:errorcluster)  [unwired: 1 in, 1 out]
      n209 = control-ref of="Info"() -> (w268:refnum<vi>)
      n210 = call <vilib>:"Initialize Joystick.vi"("error in (no error)"=w322, "device index"=w194) -> ("error out"=w192:errorcluster, "device ID"=w321:refnum<k1>)  [unwired: 8 in]
      n211 = call <vilib>:"Obtain Semaphore Reference.vi"("name (unnamed)"="AppsLock") -> ("semaphore"=w206:T63)  [unwired: 4 in, 2 out]
      n212 = case shown="False" w231 {
        tunnel: [w407 w408] -> w253
        tunnel: [w406 w409] -> w252
        tunnel: "DG535_Configs" -> [w405 _]
        tunnel: w249 -> [w404 w409]
        tunnel: w246 -> [w403 w408]
        frame False {
          n213 = call "SRS-DG535_Initializer.vi"("error in (no error)"=w404, "DG535_Configs"=w405, "Queue in"=w403) -> ("error out"=w406:errorcluster, "Queue out"=w407:refnum<queue>)  [unwired: 7 in]
        }
        frame True {
        }
      }
      n214 = case shown="False" w152 {
        tunnel: w156 -> [w392 w394]
        tunnel: [w391 w394] -> w155
        tunnel: [w390 w393] -> w151
        tunnel: w150 -> [w390 w393]
        tunnel: "BNC_Config" -> [w389 _]
        frame False {
          n215 = call "BNC_Initializer.vi"("BNC_Config"=w389, "BNC Control Queue in"=w392) -> ("BNC Ctrl queue out"=w391:refnum<queue>)  [unwired: 9 in]
        }
        frame True {
        }
      }
      n216 = Obtain Queue(name (unnamed)="AnalogDisc_StatusQuery", element data type=T57 {"Handle_DWF"=0, "Model"="", "SN"="", "TrigRate(Hz)"=0.0, "TrigCount"=0, "Mode"=enum."Normal", "STS"=enum."stsRdy", "SecondaryDataParams."={"SecondaryDataVIRef."=refnum, "Option"=0}} ("PrivateStats(Live)")) -> (queue out=w185:refnum<queue>)  [unwired: 3 in, 2 out]
      n217 = Obtain Queue(name (unnamed)="AnalogDisc_ConfigQuery", element data type=T20 {"Acqusition"={"Freq(Hz,SampleRate)"=10000000.0, "BufferSize"=8192, "Mode"=enum."Single", "RecordLength(s)"=0.0}, "Channels"=[{"Range(V)"=5.0, "Offset(V)"=0.0, "Filter"=enum."Decimate", "Enable"=TRUE}], "Trigger"={"TriggerSource"=enum."None", "Timeout(s)"=0.0, "Holdoff(s)"=1e-06, "Position/Delay(s)"=0.0}, "AnalogTrigger"={"Channel"=0, "Polarity"=enum."Rising", "Type"=enum."Pulse", "Level(V)"=0.0, "Filter"=enum."Decimate", "Hysterisis(V)"=0.0}} ("AnalogDisc_Configs 2")) -> (queue out=w183:refnum<queue>)  [unwired: 3 in, 2 out]
      n218 = Obtain Queue(name (unnamed)="Gage_ConfigQuery", element data type=T19 {"Acquisition"={"Sample Rate"=100000000.0, "Mode"=1, "Start (0)"=8192.0, "Depth"=8192.0, "Segment Size"=100.0, "Trigger Delay"=0.0, "Trigger Timeout"=0.0, "Trigger Holdoff"=0.0, "Clock mode"=enum."Internal", "Segment"=0}, "Channels"=[{"Coupling"=0, "Differential Input"=FALSE, "Direct-to-ADC"=FALSE, "Range"=2000, "Impedance"=50, "DC Offset"=0, "Filter"=0}, {"Coupling"=0, "Differential Input"=FALSE, "Direct-to-ADC"=FALSE, "Range"=2000, "Impedance"=50, "DC Offset"=0, "Filter"=0}], "Trigger"={"Slope"=0, "Level"=0, "Source"=0, "External Range"=2000, "External Coupling"=0, "External"=TRUE, "Disable"=FALSE, "External Impedance"=0}, "Mode(Gage)"=enum."Continuous"} ("Gage_Config")) -> (queue out=w180:refnum<queue>)  [unwired: 3 in, 2 out]
      n219 = Obtain Queue(name (unnamed)="Gage_StatusQuery", element data type=T55 {"Model"="", "TrigRate(Hz)"=0.0, "TrigCount"=0, "Mode(Gage)"=enum."Normal", "Handle"={"Handle"=0, "Sample size"=0, "Resolution"=0, "Offset"=0, "Channels"=0, "Boards"=0}, "DAQ_Status"=enum."Done", "SecondaryDataVIRef"=refnum, "Option(SecondaryDataVI)"=0, "cSegment"=0, "TSArray"=[], "Adj.SegmenttSize"=0.0} ("PrivateStats(Live)")) -> (queue out=w177:refnum<queue>)  [unwired: 3 in, 2 out]
      n220 = Obtain Queue(name (unnamed)="GenericDAQ_ConfigQuery", element data type=T14 {"Acquisition"={"Sample Rate"=1000000000.0, "Mode"=0, "Start (0)"=0.0, "Depth"=1024.0, "Segment"=1}, "Channels"=[{"Range"=1, "DC Offset"=0}], "Mode(Gage)"=enum."Continuous"} ("GenericDAQ_Config")) -> (queue out=w146:refnum<queue>)  [unwired: 3 in, 2 out]
      n221 = Obtain Queue(name (unnamed)="GenericDAQ_StatusQuery", element data type=T51 {"Model"="", "TrigRate(Hz)"=0.0, "TrigCount"=0, "Mode"=enum."Normal", "DAQ_Status"=enum."Done", "SecondaryDataVIRef"=refnum, "Option(SecondaryDataVI)"=0, "cSegment"=0} ("PrivateStats(Live)")) -> (queue out=w144:refnum<queue>)  [unwired: 3 in, 2 out]
      n222 = Obtain Queue(name (unnamed)="ProcCoreCtrl", element data type=w157) -> (queue out=w188:refnum<queue>, error out=w187:errorcluster)  [unwired: 3 in, 1 out]
      n223 = Obtain Queue(name (unnamed)="MainDAQ_Ctrl_Queue", element data type=T60 {"DWF States"=enum."Enumerate", "Variant"=variant}) -> (queue out=w270:refnum<queue>)  [unwired: 3 in, 2 out]
      n224 = Obtain Queue(name (unnamed)="WriterCtrl", element data type=T68 {"State"=enum."Open", "Params"=variant} ("Writer_State")) -> (queue out=w173:refnum<queue>, error out=w332:errorcluster)  [unwired: 3 in, 1 out]
      n225 = Enqueue Element(queue=w188, element=w157) -> (queue out=w163:refnum<queue>)  [unwired: 2 in, 2 out]
      n226 = Obtain Queue(max queue size (-1, unlimited)=1024, name (unnamed)="ProcCoreSignals", element data type=T59 {"tickcount"=0, "Signal"=[], "SecondaryData"=[], "Flag"=enum."Normal"} ("Signal_Typedef")) -> (queue out=w162:refnum<queue>)  [unwired: 2 in, 2 out]
      n227 = Obtain Queue(max queue size (-1, unlimited)=256, name (unnamed)="Signal Segment", element data type=T3 {"SampleRate"=0.0, "TrigDelay"=0.0, "SpecLength"=0.0, "DAQ_Range"=0.0, "Average#"=0, "Position"=[], "Spectrum"=[], "Calibr."=[], "Pressure"=0.0, "Desp_LaserEnergy"=0.0, "PI_LaserEnergy"=0.0, "Voltages Table"=[], "ProcMode"=enum."None", "Threshold"=0.0, "Comment"="", "TickCount"=0.0, "Time Stamp"=timestamp(0 s since 1904-01-01)} ("Signal Segment")) -> (queue out=w171:refnum<queue>, error out=w335:errorcluster)  [unwired: 2 in, 1 out]
      n228 = disable-structure shown="NI_DAQmx_EXIST==TRUE" {
        disable-tunnel: w330 -> [w368 w369]
        disable-tunnel: w271 -> [w367 _]
        disable-tunnel: [w366 w369] -> w227
        frame condition #0 {
          # "Legacy Code"
          n229 = call "DAQmx_ControlLoop.vi"("error in"=w368, "DAQmx Task Name"="DAQmx Task", "queue out"=w367) -> ("error out"=w366:errorcluster)  [unwired: 8 in]
        }
        frame condition #1 (active) {
        }
      }
      n230 = Bundle By Name(cluster=T62 {"LaserCtrlMethod"=enum."SRS_DG535", "Apps"=refnum, "MainDAQCoreQueue"=refnum, "Micos"=refnum, "ESP300"=refnum, "SMC100"=refnum, "SRS DG535"=refnum, "BNC"=refnum, "SDG_ii"=refnum, "NI-USB_DAQmx"=refnum, "ProcCore_CtrlQueue"=refnum, "WriterCtrl"=refnum, "WriterSIG"=refnum, "Feedback"=refnum, "EPM2000"=refnum, "InfoRef"=refnum, "AppsLock"=refnum, "ProcCore_SignalQueue"=refnum}, "SRS DG535"=w253, "BNC"=w155, "Feedback"=w272, "ESP300"=w244, "Micos"=w242, "SDG_ii"=w220, "EPM2000"=w218, "NI-USB_DAQmx"=w271, "MainDAQCoreQueue"=w270, "ProcCore_CtrlQueue"=w163, "WriterCtrl"=w173, "WriterSIG"=w171, "Apps"=w269, "InfoRef"=w268, "LaserCtrlMethod"="Laser Control Method", "AppsLock"=w206) -> (w263:T62)
      n231 = case shown="No Error" w192 {
        selector: w192 -> [w395 _]
        tunnel: w321 -> [w397 _]
        tunnel: w200 -> [w396 _]
        frame No Error {
          n232 = call "JoyStickEvent.vi"("error in"=w395, "UserEvent_Handle"=w396, "device ID"=w397) -> ()  [unwired: 9 in]
        }
        frame Error {
        }
      }
      n233 = Bundle By Name(cluster=w262, "WriterQueue"=w171) -> (w245:T65)
      n234 = call "WriteCoreLoop_v2.vi"("Controls ref."=w337, "data error in"=w335, "data queue in"=w171, 10:"control queue in"=w332, 11:"control queue in"=w173) -> ("error out"=w168:errorcluster)  [unwired: 6 in]
      n235 = call "SDGiiControlLoop.vi"("queue error in"=w341, "VISA resource"="SDG II port", "queue in"=w220) -> ("error out"=w226:errorcluster, "queue out"=w219:refnum<queue>)  [unwired: 7 in]
      n236 = call <instrlib>:"ESP30xCore.vi"("NumOfAxis"="#Axis (ESP300)", "MotorDisabled"=w260, "Simulation"="Simulation (ESP300)", "error in"=w340, "Serial Configuration"="Serial Config (ESP300)", "CommPort"="CommPort (ESP300)", "ControlQueue in"=w244) -> ("error out"=w228:errorcluster, "queue out"=w213:refnum<queue>)  [unwired: 3 in]
      n237 = call <instrlib>:"MicosCore.vi"("NumOfAxis"="#Axis (Micos)", "Simulation"="Simulation (Micos)", "error in"=w339, "Serial Configuration"="Serial Config (Micos)", "CommPort"="Micos Port", "ControlQueue in"=w242) -> ("error out"=w229:errorcluster, "queue out"=w214:refnum<queue>)  [unwired: 4 in]
      n238 = call "EPM2000ControlLoop.vi"("queue error in"=w327, "VISA resource"="Energy Meter  port", "Control queue in"=w218) -> ("error out"=w225:errorcluster, "queue out"=w217:refnum<queue>)  [unwired: 7 in]
      n239 = call "BncCore.vi"("error in"=w151, "queue in"=w155, "VISA resource"="BNC Port") -> ("error out"=w224:errorcluster, "queue out"=w216:refnum<queue>)  [unwired: 7 in]
      n240 = call <instrlib>:"DG535ControlLoop.vi"("Settings"="DG535_Configs", "error in"=w252, "queue in"=w253, "VISA resource"="SRS Port") -> ("error out"=w223:errorcluster, "queue out"=w215:refnum<queue>)  [unwired: 6 in]
      n241 = call "ProcCore.vi"("ProcessParams"=w245, "error in"=w187, "SignalBuffer in"=w162, "CtrlQueue in"=w163) -> ("error out"=w169:errorcluster)  [unwired: 7 in]
      n242 = Obtain Queue(name (unnamed)="Micos_StatusQuery", element data type=T64 {"Position"=[], "Velocity"=[], "Acceleration"=[], "Moving"=FALSE, "Simulation"=FALSE, "tickcount_mov"=0, "tickcount_pos"=0, "NumOfAxis"=0, "Initialized"=FALSE, "CommPort"="", "Range"=[], "Serial Configuration"={"Baud Rate"=0, "Parity"=0, "Data Bits"=0, "Stop Bits"=0, "Flow Control"=0}, "MotorDisabled"=refnum}) -> (queue out=w236:refnum<queue>)  [unwired: 3 in, 2 out]
      n243 = property on="MainDAQ_Selector" class="Enum (strict)"() -> ("Value"=w176:T16)  [unwired: 2 in, 2 out]
      n244 = while "UI Event Loop" {
        tunnel: w294 -> [w1151]
        tunnel: w263 -> [w1150]
        tunnel: w236 -> [w1149]
        tunnel: [w1149] -> w234
        tunnel: w205 -> [w1148]
        tunnel: w185 -> [w1147]
        tunnel: w183 -> [w1146]
        tunnel: w180 -> [w1145]
        tunnel: w177 -> [w1144]
        tunnel: w159 -> [w1142]
        shift-right: [w1141] -> _
        shift-left: w158 -> [w1143]
        tunnel: w146 -> [w1140]
        tunnel: w144 -> [w1139]
        stop <- w1153 stop-if-true
        n245 = event shown="[0] Timeout" {
          selector: w1151 -> [_ _ _ _ _ _ _ _ _ _ _ _ _ _ _ _ _ _ _ _ _ _ _ _ _ _ _ _ _ _ _ _ _ _ _ _ _ _ _ _ _ _ _ _ _ _ _ _ _ _ _ _ _ _ _ _ _ _ _]
          dyn-events: _ -> [_ _ _ _ _ _ _ _ _ _ _ _ _ _ _ _ _ _ _ _ _ _ _ _ _ _ _ _ _ _ _ _ _ _ _ _ _ _ _ _ _ _ _ _ _ _ _ _ _ _ _ _ _ _ _ _ _ _ _]
          timeout: 100 -> [_ _ _ _ _ _ _ _ _ _ _ _ _ _ _ _ _ _ _ _ _ _ _ _ _ _ _ _ _ _ _ _ _ _ _ _ _ _ _ _ _ _ _ _ _ _ _ _ _ _ _ _ _ _ _ _ _ _ _]
          tunnel: [_ TRUE ("status") w1229 _ _ _ _ _ _ _ _ _ _ _ _ _ _ _ _ _ _ _ _ _ _ _ _ _ _ _ _ _ _ _ _ _ _ _ _ _ _ _ _ _ _ _ _ _ _ _ _ _ _ _ _ _ _ _ _] -> w1153
          tunnel: w1150 -> [w1179 w1223 w1230 w1334 w1337 w1346 w1365 w1378 w1385 w1393 w1400 w1442 w1477 w1514 w1538 w1554 w1574 w1588 w1596 w1612 _ _ w1643 w1654 w1682 w1718 w1755 w1763 w1774 w1780 w1790 w1796 w1800 w1814 w1843 w1851 _ w1866 w1882 _ w1899 w1922 w1948 w1978 _ w2062 w2073 w2080 w2117 w2160 _ _ _ _ _ _ _ _ _]
          tunnel: w1149 -> [w1170 _ _ _ _ _ _ _ _ _ _ _ _ _ _ _ _ _ _ _ _ _ _ _ _ _ _ _ _ _ _ _ _ _ _ _ _ _ _ _ _ _ _ _ _ _ _ _ _ _ _ _ _ _ _ _ _ _ _]
          tunnel: w1148 -> [_ _ _ _ _ _ _ _ _ _ w1401 w1443 w1479 _ _ _ _ _ _ _ _ _ _ _ _ _ _ _ _ _ _ _ _ _ _ _ _ _ _ _ _ _ _ _ _ _ _ _ _ _ _ _ _ _ _ _ _ _ _]
          tunnel: w1147 -> [w1165 _ _ _ _ _ _ _ _ _ _ _ _ _ _ _ _ _ _ _ _ _ _ _ _ _ _ _ _ _ _ _ _ _ _ _ _ _ _ _ _ _ _ _ _ _ _ _ _ _ _ _ _ _ _ _ _ _ _]
          tunnel: w1146 -> [_ _ _ _ _ _ _ _ _ _ _ _ _ _ _ _ _ _ _ _ _ _ _ _ w1677 _ _ _ _ _ _ _ _ _ _ _ _ _ _ _ _ _ _ _ _ _ _ _ _ _ _ _ _ _ _ _ _ _ _]
          tunnel: w1145 -> [_ _ _ _ _ _ _ _ _ _ _ _ _ _ _ _ _ _ _ _ _ _ _ _ _ w1703 _ _ _ _ _ _ _ _ _ _ _ _ _ _ _ _ _ _ _ _ _ _ _ _ _ _ _ _ _ _ _ _ _]
          tunnel: w1144 -> [w1166 _ _ _ _ _ _ _ _ _ _ _ _ _ _ _ _ _ _ _ _ _ _ _ _ _ _ _ _ _ _ _ _ _ _ _ _ _ _ _ _ _ _ _ _ _ _ _ _ _ _ _ _ _ _ _ _ _ _]
          tunnel: w1143 -> [w1163 w1222 w1228 w1315 w1335 w1343 w1363 w1376 w1380 w1387 w1395 w1435 w1475 w1495 w1532 w1552 w1572 w1581 w1589 w1602 w1619 w1625 w1635 w1646 w1658 w1688 w1728 w1761 w1772 w1778 w1787 w1794 w1798 w1812 w1841 w1849 w1857 w1864 w1872 w1890 w1893 w1918 w1943 w1969 w2004 w2055 w2066 w2077 w2114 w2157 w2165 w2183 w2185 w2192 w2215 w2225 w2250 w2285 w2298]
          tunnel: w1142 -> [_ _ _ _ _ _ _ _ _ _ _ _ _ _ _ _ _ _ _ _ _ _ _ _ _ _ _ _ _ _ _ _ _ _ _ _ _ _ _ _ _ _ _ _ _ _ _ _ _ _ _ _ _ _ _ _ _ _ w2299]
          tunnel: [w1163 w1222 w1228 w1315 w1335 w1342 w1362 w1376 w1380 w1387 w1395 w1435 w1475 w1495 w1532 w1552 w1572 w1581 w1589 w1602 w1619 w1625 w1634 w1645 w1657 w1687 w1728 w1761 w1771 w1778 w1786 w1794 w1798 w1811 w1841 w1849 w1857 w1864 w1872 w1890 w1893 w1917 w1944 w1968 w2001 w2054 w2066 w2077 w2114 w2157 w2165 w2183 w2185 w2192 w2215 w2225 w2250 w2285 w2298] -> w1141
          tunnel: w1140 -> [_ _ _ _ _ _ _ _ _ _ _ _ _ _ _ _ _ _ _ _ _ _ _ _ _ _ w1725 _ _ _ _ _ _ _ _ _ _ _ _ _ _ _ _ _ _ _ _ _ _ _ _ _ _ _ _ _ _ _ _]
          tunnel: w1139 -> [w1154 _ _ _ _ _ _ _ _ _ _ _ _ _ _ _ _ _ _ _ _ _ _ _ _ _ _ _ _ _ _ _ _ _ _ _ _ _ _ _ _ _ _ _ _ _ _ _ _ _ _ _ _ _ _ _ _ _ _]
          event Timeout {
            n246 = event-data() -> ()  [unwired: 1 in, 1 out]
            n247 = Unbundle By Name(w1179) -> ("MainDAQCoreQueue"=w1169:refnum<queue>, "Micos"=w1178:refnum<queue>)
            n248 = Bundle By Name(cluster=T86 {"State"=enum."QueryStatus", "Params."=variant} ("element"), "Params."=w1170) -> (w1181:T86)
            n249 = Enqueue Element "Set return ref."(queue=w1178, element=w1181) -> (error out=w1183:errorcluster)  [unwired: 2 in, 2 out]
            n250 = case "Refresh Trigger Rate (Hz)" shown="\"KnifeEdge_Emu\", \"FakeSignal(Emulator)\"" "MainDAQ_Selector" {
              tunnel: w1169 -> [_ w1200 w1208 w1216]
              tunnel: [0 ("TrigCount") w1194 w1202 w1210] -> w1168
              tunnel: w1166 -> [_ _ w1201 _]
              tunnel: w1165 -> [_ w1193 _ _]
              tunnel: w1154 -> [_ _ _ w1209]
              frame "None", Default {
              }
              frame "AnalogDisc" {
                n251 = Bundle By Name(cluster=T60 {"DWF States"=enum."GetStat_", "Variant"=variant} ("element"), "Variant"=w1193) -> (w1198:T60)
                n252 = Enqueue Element "Set Return Ref."(queue=w1200, element=w1198) -> (error out=w1196:errorcluster)  [unwired: 2 in, 2 out]
                n253 = Dequeue Element(queue=w1193, timeout in ms (-1)=1000, error in (no error)=w1196) -> (element=w1195:T57)  [unwired: 3 out]
                n254 = Unbundle By Name(w1195) -> ("TrigCount"=w1194:i32)
              }
              frame "Gage" {
                n255 = Bundle By Name(cluster=T60 {"DWF States"=enum."GetStat_", "Variant"=variant} ("element"), "Variant"=w1201) -> (w1206:T60)
                n256 = Enqueue Element "Set Return Ref."(queue=w1208, element=w1206) -> (error out=w1204:errorcluster)  [unwired: 2 in, 2 out]
                n257 = Dequeue Element(queue=w1201, timeout in ms (-1)=1000, error in (no error)=w1204) -> (element=w1203:T55)  [unwired: 3 out]
                n258 = Unbundle By Name(w1203) -> ("TrigCount"=w1202:i32)
              }
              frame "KnifeEdge_Emu", "FakeSignal(Emulator)" {
                n259 = Bundle By Name(cluster=T60 {"DWF States"=enum."GetStat_", "Variant"=variant} ("element"), "Variant"=w1209) -> (w1214:T60)
                n260 = Enqueue Element "Set Return Ref."(queue=w1216, element=w1214) -> (error out=w1212:errorcluster)  [unwired: 2 in, 2 out]
                n261 = Dequeue Element(queue=w1209, timeout in ms (-1)=1000, error in (no error)=w1212) -> (element=w1211:T51)  [unwired: 3 out]
                n262 = Unbundle By Name(w1211) -> ("TrigCount"=w1210:i32)
              }
            }
            n263 = global read "MiscParams.vi" "IonLaserEnergy"() -> (w1186:dbl)
            n264 = Dequeue Element(queue=w1170, timeout in ms (-1)=1000, error in (no error)=w1183) -> (element=w1177:T64)  [unwired: 3 out]
            n265 = global read "MiscParams.vi" "DspLaserEnergy"() -> (w1189:dbl)
            n266 = Unbundle By Name(w1177) -> ("Position"=→"Position(Micos)":dbl[], "Velocity"=w1176:dbl[], "Acceleration"=w1175:dbl[], "Moving"=→"Moving (Micos)":bool)  [unwired: 1 out]
            n267 = Multiply(x="fsEnergyCoeff.", y=w1189) -> (x*y=w1184:dbl)
            "LaserEnergy" <- w1184
            n268 = Multiply(x="YAGEnergyCoeff.", y=w1186) -> (x*y=w1185:dbl)
            "Nd:YAG Energy" <- w1185
            n269 = Index Array(array=w1176) -> (element=→"Velcoty_ind_micos":dbl)  [unwired: 1 in]
            n270 = Index Array(array=w1175) -> (element=→"Accele._ind_micos":dbl)  [unwired: 1 in]
            n271 = local read "Signal Segment"() -> (w1190:T3)
            n272 = Bundle By Name(cluster=w1190, "PI_LaserEnergy"=w1185, "Desp_LaserEnergy"=w1184) -> (w1191:T3)
            n273 = call "TriggerRateCalculator.vi"("Count"=w1168) -> ("rep rate"=→"Trig. Rate (Hz)":dbl)  [unwired: 10 in]
            n274 = local write "Signal Segment"(w1191) -> ()
            n275 = global read "Position_ESP300.vi" "Position_ESP"() -> (w1156:dbl[])
            "Position(ESP)" <- w1156
            n276 = global read "Position_ESP300.vi" "Moving"() -> (→"Moving (Newport)":bool)
            n277 = local read "ZeroDelayPos"() -> (w1159:dbl)
            n278 = Index Array(array=w1156) -> (element #1=w1157:dbl, element #2=w1158:dbl)  [unwired: 2 in]
            n279 = Compound Arithmetic op=ADD(w1157, w1158, invert w1159) -> (w1160:dbl)
            n280 = Multiply(x=w1160, y=6.671281903) -> (x*y=→"DP_Delay (ps)_indicator":dbl)
          }
          event "Quit": Value Change; Panel Close; Application Instance Close {
            n281 = event-data() -> ()  [unwired: 1 in, 1 out]
            n282 = Unbundle By Name(w1223) -> ("Apps"=w1224:refnum<queue>)
            n283 = local write "Quit"(FALSE ("Quit")) -> ()
            n284 = Enqueue Element(queue=w1224, element=States-AToF."Quit") -> ()  [unwired: 2 in, 3 out]
            n285 = control-ref of="This VI"() -> (w1220:refnum<vi>)
            n286 = property class="VI"(reference=w1220) -> ("Path"=w1218:path)  [unwired: 1 in, 2 out]
            n287 = Strip Path(path=w1218) -> (stripped path=w1217:path)  [unwired: 1 out]
            n288 = Build Path(base path=w1217, name or relative path=path "Configs/Previous.conf.json" ("ConfigFile Path")) -> (appended path=w1219:path)
            n289 = call "SaveConfigs_toFile.vi"("ConfigFile Path"=w1219, "Configuration"=w1222) -> ()  [unwired: 10 in]
          }
          event Menu Selection (User) {
            n290 = event-data() -> ("ItemTag"=w1232:string, "ItemPath"=w1231:string)  [unwired: 1 in]
            n291 = case shown="\"DepthProfiling(3D)\"" w1232 {
              tunnel: w1231 -> [w1236 _ _ _ _ _ _ _ _ _ _ _ _ _ _ _]
              tunnel: w1230 -> [_ w1240 _ w1264 w1267 w1270 w1272 w1283 w1286 w1289 w1292 w1294 w1299 w1308 _ _]
              tunnel: [_ TRUE _ _ _ _ _ _ _ _ _ _ _ _ _ _] -> w1229
              tunnel: w1228 -> [_ _ w1260 _ _ _ _ _ _ _ _ _ _ _ _ _]
              frame Default {
                n292 = Concatenate Strings(w1236, "\r\n", "This function is not supported by menu yet.") -> (w1235:string)
                n293 = One Button Dialog(message=w1235, button name ("OK")="I know") -> ()  [unwired: 1 out]
              }
              frame "Exit" {
                n294 = Unbundle By Name(w1240) -> ("Apps"=w1239:refnum<queue>)
                n295 = Enqueue Element(queue=w1239, element=States-AToF."Quit") -> ()  [unwired: 2 in, 3 out]
              }
              frame "SaveConfigs" {
                n296 = control-ref of="This VI"() -> (w1253:refnum<vi>)
                n297 = property class="VI"(reference=w1253) -> ("Path"=w1252:path)  [unwired: 1 in, 2 out]
                n298 = Build Path(base path=w1252, name or relative path=".\\Configs\\Default.conf.json") -> (appended path=w1250:path)
                n299 = feedback #2(w1250) -> (w1257:path)
                n300 = Strip Path(path=w1257) -> (stripped path=w1255:path, name=w1256:string)
                n301 = call "File Dialog3"("start path"=w1255, "default name"=w1256, "pattern (all files)"="*.conf.json", "pattern label"="Json Configuration Files") -> ("selected path"=w1243:path, "cancelled"=w1254:bool)  [unwired: 8 in, 2 out]
                n302 = feedback-in #2(w1243) -> ()
                n303 = Strip Path(path=w1243) -> (stripped path=w1245:path, name=w1249:string)
                n304 = Search and Replace String(case sensitive?=TRUE ("ignore case? (F)"), input string=w1249, search string=".conf.json.conf.json", replace string=".conf.json" ("replace string (\"\")")) -> (result string=w1244:string)  [unwired: 4 in, 3 out]
                n305 = Build Path(base path=w1245, name or relative path=w1244) -> (appended path=w1242:path)
                n306 = case shown="False" w1254 {
                  tunnel: w1260 -> [w1262 _]
                  tunnel: w1242 -> [w1261 _]
                  frame False {
                    n307 = call "SaveConfigs_toFile.vi"("ConfigFile Path"=w1261, "Configuration"=w1262) -> ()  [unwired: 10 in]
                  }
                  frame True {
                  }
                }
              }
              frame "EnergyCalibration" {
                n308 = Unbundle By Name(w1264) -> ("Apps"=w1263:refnum<queue>)
                n309 = Enqueue Element(queue=w1263, element=States-AToF."EnergyCalibration") -> ()  [unwired: 2 in, 3 out]
              }
              frame "BeamProfile Measurement" {
                n310 = Unbundle By Name(w1267) -> ("Apps"=w1266:refnum<queue>)
                n311 = Enqueue Element(queue=w1266, element=States-AToF."KnifeEdgeExpt") -> ()  [unwired: 2 in, 3 out]
              }
              frame "DepthProfile" {
                n312 = Unbundle By Name(w1270) -> ("Apps"=w1269:refnum<queue>)
                n313 = Enqueue Element(queue=w1269, element=States-AToF."DepthProfile_RT") -> ()  [unwired: 2 in, 3 out]
              }
              frame "Reset_Micos" {
                n314 = Two Button Dialog(message="Reset Micos? \nHave all subroutines stopped? \nIf not, stop them first. \n", 1:"Cancel" ("F button name (\"Cancel\")"), 2:"Reset Micos" ("T button name (\"OK\")")) -> (T button?=w1276:bool)
                n315 = case shown="True" w1276 {
                  tunnel: w1272 -> [_ w1281]
                  frame False {
                  }
                  frame True {
                    n316 = Unbundle By Name(w1281) -> ("Micos"=w1278:refnum<queue>)
                    n317 = Enqueue Element(queue=w1278, element=T74 {"State"=enum."Close", "Params."=variant}) -> (error out=w1277:errorcluster)  [unwired: 2 in, 2 out]
                    n318 = Enqueue Element(queue=w1278, element=T74 {"State"=enum."Initialize", "Params."=variant}, error in (no error)=w1277) -> ()  [unwired: 1 in, 3 out]
                  }
                }
              }
              frame "Imaging" {
                n319 = Unbundle By Name(w1283) -> ("Apps"=w1282:refnum<queue>)
                n320 = Enqueue Element(queue=w1282, element=States-AToF."Imaging_Micos") -> ()  [unwired: 2 in, 3 out]
              }
              frame "DepthProfiling(3D)" {
                n321 = Unbundle By Name(w1286) -> ("Apps"=w1285:refnum<queue>)
                n322 = Enqueue Element(queue=w1285, element=States-AToF."DepthProfiling(3D)") -> ()  [unwired: 2 in, 3 out]
              }
              frame "BeamProfile Measurement (ESP)" {
                n323 = Unbundle By Name(w1289) -> ("Apps"=w1288:refnum<queue>)
                n324 = Enqueue Element(queue=w1288, element=States-AToF."KnifeEdgeExpt_Npt") -> ()  [unwired: 2 in, 3 out]
              }
              frame "Cleanup Surface" {
                n325 = Unbundle By Name(w1292) -> ("Apps"=w1291:refnum<queue>)
                n326 = Enqueue Element(queue=w1291, element=States-AToF."CleanSurface") -> ()  [unwired: 2 in, 3 out]
              }
              frame "ResetEPM2000" {
                n327 = Unbundle By Name(w1294) -> ("EPM2000"=w1298:refnum<queue>)
                n328 = Enqueue Element(queue=w1298, element=T83 {"State"=enum."Close", "Parameter"=0.0}) -> (queue out=w1297:refnum<queue>)  [unwired: 2 in, 2 out]
                n329 = Enqueue Element(queue=w1297, element=T83 {"State"=enum."Initialize", "Parameter"=0.0}) -> ()  [unwired: 2 in, 3 out]
              }
              frame "ResetBNC" {
                n330 = Unbundle By Name(w1299) -> ("BNC"=w1303:refnum<queue>)
                n331 = Enqueue Element(queue=w1303, element=T84 {"State"=enum."Close", "Para."=variant}) -> (queue out=w1300:refnum<queue>)  [unwired: 2 in, 2 out]
                n332 = Enqueue Element(queue=w1300, element=T84 {"State"=enum."Initialize", "Para."=variant}) -> ()  [unwired: 2 in, 3 out]
              }
              frame "ResetSDGii" {
                n333 = Unbundle By Name(w1308) -> ("SDG_ii"=w1307:refnum<queue>)
                n334 = Enqueue Element(queue=w1307, element=T70 {"State"=enum."Close", "Parameter"=0.0}) -> (queue out=w1304:refnum<queue>)  [unwired: 2 in, 2 out]
                n335 = Enqueue Element(queue=w1304, element=T70 {"State"=enum."Initialize", "Parameter"=0.0}) -> ()  [unwired: 2 in, 3 out]
              }
              frame "SaveCurrentGraph" {
                n336 = control-ref of="Snap"() -> (w1312:refnum<vi>)
                n337 = property class="Bool (strict)"(reference=w1312) -> (reference out=w1309:refnum<vi>, error out=w1310:errorcluster, "Value"=w1311:bool)  [unwired: 1 in]
                n338 = property class="Bool (strict)"(reference=w1309, error in=w1310, "Val(Sgnl)"=w1311) -> ()  [unwired: 2 out]
              }
              frame "MassCalibration", "StartAnalysisTool" {
                n339 = control-ref of="Cali."() -> (w1314:refnum<vi>)
                n340 = vi-ref "AnalysisTools.vi"() -> (w1313:refnum<vi>)
                n341 = call-by-ref "?"(reference=w1313, "Cali.Ref(Caller)"=w1314) -> ()  [unwired: 12 in, 2 out]
              }
            }
          }
          event "Down(ESP)", "Left(ESP)", "Right(ESP)", "Up(ESP)": Value Change {
            n342 = event-data() -> ()  [unwired: 1 in, 1 out]
            n343 = Unbundle By Name(w1334) -> ("ESP300"=w1333:refnum<queue>)
            n344 = Build Array("Up(ESP)", "Down(ESP)", "Left(ESP)", "Right(ESP)") -> (w1328:bool[])
            n345 = Search 1D Array(1D array=w1328, element=TRUE) -> (index of element=w1322:i32)  [unwired: 1 in]
            n346 = Index Array(array=dbl[] [1.0, -1.0, -1.0, 1.0], index=w1322) -> (element=w1325:dbl)
            n347 = Index Array(array=i32[] [2, 2, 1, 1], index=w1322) -> (element=w1326:i32)
            n348 = local read "StepWidth (ESP)"() -> (w1316:T6)
            n349 = Multiply(x=w1325, y=w1316) -> (x*y=w1318:T6)
            n350 = Bundle By Name(cluster=cluster{"Axis":i32, "Position":dbl} {"Axis"=0, "Position"=0.0}, "Position"=w1318, "Axis"=w1326) -> (w1317:cluster{"Axis":i32, "Position":dbl})
            n351 = Bundle By Name(cluster=T74 {"State"=enum."MoveRel", "Params."=variant} ("element"), "Params."=w1317) -> (w1320:T74)
            n352 = Enqueue Element(queue=w1333, element=w1320) -> ()  [unwired: 2 in, 3 out]
          }
          event "Destination(ESP)", "Go(ESP)": Value Change {
            n353 = event-data() -> ()  [unwired: 1 in, 2 out]
            n354 = Unbundle By Name(w1337) -> ("ESP300"=w1336:refnum<queue>)
            n355 = Bundle By Name(cluster=T74 {"State"=enum."MoveAbs_all", "Params."=variant} ("element"), "Params."="Destination(ESP)") -> (w1339:T74)
            n356 = Enqueue Element(queue=w1336, element=w1339) -> ()  [unwired: 2 in, 3 out]
          }
          event "Velocity (ESP)", "Velocity (ESP) #3": Value Change {
            n357 = event-data() -> ()  [unwired: 1 in, 1 out]
            n358 = Unbundle By Name(w1346) -> ("ESP300"=w1345:refnum<queue>)
            n359 = property on="#Axis (ESP300)" class="DigNum (strict)"() -> ("Value"=w1347:i32)  [unwired: 2 in, 2 out]
            n360 = for {
              N: w1347 -> [_]
              tunnel: "Velocity (ESP)" -> [w1353]
              tunnel: w1345 -> [w1355]
              tunnel: "Velocity (ESP) #3" -> [w1354]
              tunnel: [w1349] -> w1341 mode=indexing
              i -> [w1360]
              n361 = Increment(x=w1360) -> (x+1=w1352:i32)
              n362 = Equal?(x=3, y=w1352) -> (x = y?=w1350:bool)
              n363 = Select(t=w1354, s=w1350, f=w1353) -> (s? t:f=w1349:dbl)
              n364 = Bundle By Name(cluster=cluster{"Axis":i32, "Velocity":dbl} {"Axis"=0, "Velocity"=0.0}, "Velocity"=w1349, "Axis"=w1352) -> (w1356:cluster{"Axis":i32, "Velocity":dbl})
              n365 = Bundle By Name(cluster=T74 {"State"=enum."SetVelocity", "Params."=variant} ("element"), "Params."=w1356) -> (w1358:T74)
              n366 = Enqueue Element(queue=w1355, element=w1358) -> ()  [unwired: 2 in, 3 out]
            }
            n367 = Bundle By Name(cluster=w1343, "ESP300.Velocity"=w1341) -> (w1342:T50)
          }
          event "Accele. (ESP)": Value Change {
            n368 = event-data() -> ()  [unwired: 1 in, 2 out]
            n369 = Unbundle By Name(w1365) -> ("ESP300"=w1364:refnum<queue>)
            n370 = property on="#Axis (ESP300)" class="DigNum (strict)"() -> ("Value"=w1367:i32)  [unwired: 2 in, 2 out]
            n371 = for {
              N: w1367 -> [_]
              tunnel: "Accele. (ESP)" -> [w1368]
              tunnel: w1364 -> [w1370]
              tunnel: [w1368] -> w1361 mode=indexing
              i -> [w1375]
              n372 = Increment(x=w1375) -> (x+1=w1374:i32)
              n373 = Bundle By Name(cluster=cluster{"Axis":i32, "Acceleration":dbl} {"Axis"=0, "Acceleration"=0.0}, "Acceleration"=w1368, "Axis"=w1374) -> (w1371:cluster{"Axis":i32, "Acceleration":dbl})
              n374 = Bundle By Name(cluster=T74 {"State"=enum."SetAcceleration", "Params."=variant} ("element"), "Params."=w1371) -> (w1373:T74)
              n375 = Enqueue Element(queue=w1370, element=w1373) -> ()  [unwired: 2 in, 3 out]
            }
            n376 = Bundle By Name(cluster=w1363, "ESP300.Acceleration"=w1361) -> (w1362:T50)
          }
          event "HomeSearch(ESP)": Value Change {
            n377 = event-data() -> ()  [unwired: 1 in, 1 out]
            n378 = Unbundle By Name(w1378) -> ("ESP300"=w1377:refnum<queue>)
            n379 = Enqueue Element(queue=w1377, element=T74 {"State"=enum."Origin/Home", "Params."=variant}) -> ()  [unwired: 2 in, 3 out]
          }
          event "MotorDisabled(ESP)": Value Change {
            n380 = event-data() -> ()  [unwired: 1 in, 1 out]
            n381 = Unbundle By Name(w1385) -> ("ESP300"=w1384:refnum<queue>)
            n382 = Not(x="MotorDisabled(ESP)") -> (.not. x?=w1381:bool)
            n383 = Bundle By Name(cluster=T74 {"State"=enum."MotorEnable(1)", "Params."=variant} ("element"), "Params."=w1381) -> (w1383:T74)
            n384 = Enqueue Element(queue=w1384, element=w1383) -> ()  [unwired: 2 in, 3 out]
          }
          event "STOP(ESP)": Value Change {
            # "think about race condition !!"
            n385 = event-data() -> ()  [unwired: 1 in, 1 out]
            n386 = Unbundle By Name(w1393) -> ("Apps"=w1391:refnum<queue>, "ESP300"=w1392:refnum<queue>)
            n387 = Enqueue Element(queue=w1391, element=States-AToF."Interrupted_Stop") -> (error out=w1389:errorcluster)  [unwired: 2 in, 2 out]
            n388 = call <vilib>:"Clear Errors.vi"("error in (no error)"=w1389) -> ("error out"=w1388:errorcluster)  [unwired: 6 in]
            n389 = Enqueue Element(queue=w1392, element=T74 {"State"=enum."STOP", "Params."=variant}, error in (no error)=w1388) -> ()  [unwired: 1 in, 3 out]
          }
          event User Event {
            n390 = event-data() -> ("Direction"=w1405:i32, "Step"=w1398:i32)  [unwired: 1 in]
            n391 = local read "StepWidth (Micos)"() -> (w1403:T6)
            n392 = Unbundle By Name(w1400) -> ("AppsLock"=w1397:T63, "Micos"=w1408:refnum<queue>, "ESP300"=w1407:refnum<queue>)
            n393 = local read "StepWidth (ESP)"() -> (w1402:T6)
            n394 = Select(t=w1408, s=w1401, f=w1407) -> (s? t:f=w1406:refnum<queue>)
            n395 = Select(t=w1403, s=w1401, f=w1402) -> (s? t:f=w1399:T6)
            n396 = call <vilib>:"Acquire Semaphore.vi"("ms timeout (-1)"=0, "semaphore"=w1397) -> ("timed out"=w1409:bool, "semaphore out"=w1396:T63)  [unwired: 3 in, 1 out]
            n397 = case shown="False" w1409 {
              tunnel: w1406 -> [w1412 _]
              tunnel: w1405 -> [w1416 _]
              tunnel: i32[] [0, 90, 180, 270, -2] -> [w1417 _]
              tunnel: w1399 -> [w1414 _]
              tunnel: w1398 -> [w1413 _]
              tunnel: w1396 -> [w1411 _]
              frame False {
                n398 = Search 1D Array(1D array=w1417, element=w1416) -> (index of element=w1415:i32)  [unwired: 1 in]
                n399 = case shown="0..3" w1415 {
                  selector: w1415 -> [_ w1425]
                  tunnel: w1414 -> [_ w1427]
                  tunnel: w1413 -> [_ w1424]
                  tunnel: w1412 -> [_ w1422]
                  tunnel: w1411 -> [_ w1418]
                  frame Default {
                  }
                  frame 0..3 {
                    n400 = Index Array(array=dbl[] [1.0, -1.0, -1.0, 1.0], index=w1425) -> (element=w1426:dbl)
                    n401 = Index Array(array=i32[] [2, 1, 2, 1], index=w1425) -> (element=w1434:i32)
                    n402 = Compound Arithmetic op=MULTIPLY(w1427, w1426, w1424) -> (w1429:T6)
                    n403 = Bundle By Name(cluster=cluster{"Axis":i32, "Position":dbl} {"Axis"=0, "Position"=0.0}, "Position"=w1429, "Axis"=w1434) -> (w1428:cluster{"Axis":i32, "Position":dbl})
                    n404 = Bundle By Name(cluster=T74 {"State"=enum."MoveRel", "Params."=variant} ("element"), "Params."=w1428) -> (w1423:T74)
                    n405 = Enqueue Element(queue=w1422, element=w1423, timeout in ms (-1)=50) -> (error out=w1419:errorcluster)  [unwired: 1 in, 2 out]
                    n406 = call <vilib>:"Clear Errors.vi"("error in (no error)"=w1419) -> ("error out"=w1420:errorcluster)  [unwired: 6 in]
                    n407 = call <vilib>:"Release Semaphore.vi"("error in (no error)"=w1420, "semaphore"=w1418) -> ()  [unwired: 4 in, 2 out]
                  }
                }
              }
              frame True {
              }
            }
          }
          event User Event {
            w1439 = 1.0  # Pitch
            n408 = event-data() -> ("Direction"=w1445:i32, "Speed"=w1440:dbl)  [unwired: 1 in]
            n409 = Unbundle By Name(w1442) -> ("AppsLock"=w1437:T63, "Micos"=w1448:refnum<queue>, "ESP300"=w1447:refnum<queue>)
            n410 = Select(t=w1448, s=w1443, f=w1447) -> (s? t:f=w1446:refnum<queue>)
            n411 = call <vilib>:"Acquire Semaphore.vi"("ms timeout (-1)"=0, "semaphore"=w1437) -> ("timed out"=w1449:bool, "semaphore out"=w1436:T63)  [unwired: 3 in, 1 out]
            n412 = Select(t=w1439, s=w1443, f=1.0) -> (s? t:f=w1441:dbl)
            n413 = case shown="False" w1449 {
              tunnel: w1446 -> [w1452 _]
              tunnel: w1445 -> [w1453 _]
              tunnel: i32[] [1, 2, 3, 6, -2] -> [w1457 _]
              tunnel: w1441 -> [w1455 _]
              tunnel: w1440 -> [w1454 _]
              tunnel: w1436 -> [w1451 _]
              frame False {
                n414 = Search 1D Array(1D array=w1457, element=w1453) -> (index of element=w1456:i32)  [unwired: 1 in]
                n415 = case shown="0, 1" w1456 {
                  selector: w1456 -> [_ w1467]
                  tunnel: w1455 -> [_ w1469]
                  tunnel: w1454 -> [_ w1470]
                  tunnel: w1453 -> [_ w1468]
                  tunnel: w1452 -> [_ w1462]
                  tunnel: w1451 -> [_ w1459]
                  frame Default {
                  }
                  frame 0, 1 {
                    n416 = Index Array(array=dbl[] [1.0, -1.0], index=w1467) -> (element=w1465:dbl)
                    n417 = Compound Arithmetic op=MULTIPLY(3.0, w1469, w1465, w1470) -> (w1472:dbl)
                    n418 = Bundle By Name(cluster=cluster{"Axis":i32, "Speed(rev/s)":dbl} {"Axis"=0, "Speed(rev/s)"=0.0}, "Speed(rev/s)"=w1472, "Axis"=w1468) -> (w1471:cluster{"Axis":i32, "Speed(rev/s)":dbl})
                    n419 = Bundle By Name(cluster=T74 {"State"=enum."JoyStick", "Params."=variant} ("element"), "Params."=w1471) -> (w1464:T74)
                    n420 = Enqueue Element(queue=w1462, element=w1464, timeout in ms (-1)=0) -> (error out=w1460:errorcluster)  [unwired: 1 in, 2 out]
                    n421 = call <vilib>:"Clear Errors.vi"("error in (no error)"=w1460) -> ("error out"=w1461:errorcluster)  [unwired: 6 in]
                    n422 = call <vilib>:"Release Semaphore.vi"("error in (no error)"=w1461, "semaphore"=w1459) -> ()  [unwired: 4 in, 2 out]
                  }
                }
              }
              frame True {
              }
            }
          }
          event User Event {
            n423 = event-data() -> ()  [unwired: 1 in, 1 out]
            n424 = Unbundle By Name(w1477) -> ("Micos"=w1482:refnum<queue>, "ESP300"=w1481:refnum<queue>)
            n425 = Unbundle By Name(w1477) -> ("AppsLock"=w1478:T63)
            n426 = call <vilib>:"Acquire Semaphore.vi"("ms timeout (-1)"=0, "semaphore"=w1478) -> ("timed out"=w1483:bool, "semaphore out"=w1476:T63)  [unwired: 3 in, 1 out]
            n427 = Select(t=w1482, s=w1479, f=w1481) -> (s? t:f=w1480:refnum<queue>)
            n428 = case shown="False" w1483 {
              tunnel: w1480 -> [w1494 _]
              tunnel: w1476 -> [w1488 _]
              frame False {
                n429 = Enqueue Element(queue=w1494, element=T74 {"State"=enum."STOP", "Params."=variant}) -> (error out=w1489:errorcluster)  [unwired: 2 in, 2 out]
                n430 = call <vilib>:"Clear Errors.vi"("error in (no error)"=w1489) -> ("error out"=w1486:errorcluster)  [unwired: 6 in]
                n431 = call <userlib>:"Wait (ms)__ogtk.vi"("error in (no error)"=w1486, "milliseconds to wait"=u32 250) -> ("error out"=w1487:errorcluster)  [unwired: 8 in, 1 out]
                n432 = call <vilib>:"Release Semaphore.vi"("error in (no error)"=w1487, "semaphore"=w1488) -> ()  [unwired: 4 in, 2 out]
                n433 = feedback #3(0) -> (w1491:i32)
                n434 = Increment(x=w1491) -> (x+1=w1492:i32)
                n435 = feedback-in #3(w1492) -> ()
              }
              frame True {
              }
            }
          }
          event "Up", "Down", "Left", "Right", "Up(+)", "Down(-)", "Left(+)", "Right(-)", "Front", "Back", "Front(-)", "Back(+)": Value Change {
            n436 = event-data() -> ()  [unwired: 1 in, 1 out]
            n437 = Unbundle By Name(w1514) -> ("Micos"=w1513:refnum<queue>, "AppsLock"=w1510:T63)
            n438 = call <vilib>:"Acquire Semaphore.vi"("ms timeout (-1)"=0, "semaphore"=w1510) -> ("timed out"=w1511:bool, "semaphore out"=w1496:T63)  [unwired: 3 in, 1 out]
            n439 = Build Array("Up", "Down", "Left", "Right", "Front", "Back", "Up(+)", "Down(-)", "Left(+)", "Right(-)", "Front(-)", "Back(+)") -> (w1500:bool[])
            n440 = case shown="False" w1511 {
              tunnel: w1513 -> [w1525 _]
              tunnel: w1500 -> [w1518 _]
              tunnel: w1496 -> [w1516 _]
              frame False {
                n441 = Search 1D Array(1D array=w1518, element=TRUE) -> (index of element=w1526:i32)  [unwired: 1 in]
                n442 = local read "StepWidth (Micos)"() -> (w1519:T6)
                n443 = Index Array(array=dbl[] [1.0, -1.0, 1.0, -1.0, -1.0, 1.0, 5.0, -5.0, 5.0, -5.0, -5.0, 5.0], index=w1526) -> (element=w1529:dbl)
                n444 = Index Array(array=i32[] [2, 2, 1, 1, 3, 3, 2, 2, 1, 1, 3, 3], index=w1526) -> (element=w1530:i32)
                n445 = Multiply(x=w1529, y=w1519) -> (x*y=w1521:T6)
                n446 = Bundle By Name(cluster=cluster{"Axis":i32, "Position":dbl} {"Axis"=0, "Position"=0.0}, "Position"=w1521, "Axis"=w1530) -> (w1520:cluster{"Axis":i32, "Position":dbl})
                n447 = Bundle By Name(cluster=T74 {"State"=enum."MoveRel", "Params."=variant} ("element"), "Params."=w1520) -> (w1523:T74)
                n448 = Enqueue Element(queue=w1525, element=w1523) -> (error out=w1515:errorcluster)  [unwired: 2 in, 2 out]
                n449 = call <vilib>:"Clear Errors.vi"("error in (no error)"=w1515) -> ("error out"=w1517:errorcluster)  [unwired: 6 in]
                n450 = call <vilib>:"Release Semaphore.vi"("error in (no error)"=w1517, "semaphore"=w1516) -> ()  [unwired: 4 in, 2 out]
              }
              frame True {
              }
            }
          }
          event "Focus (+)": Value Change {
            n451 = event-data() -> ()  [unwired: 1 in, 1 out]
            n452 = Unbundle By Name(w1538) -> ("Micos"=w1537:refnum<queue>, "AppsLock"=w1534:T63)
            n453 = call <vilib>:"Acquire Semaphore.vi"("ms timeout (-1)"=0, "semaphore"=w1534) -> ("timed out"=w1535:bool, "semaphore out"=w1533:T63)  [unwired: 3 in, 1 out]
            n454 = case shown="False" w1535 {
              tunnel: w1537 -> [w1544 _]
              tunnel: w1533 -> [w1539 _]
              frame False {
                w1542 = 60.0  # Incidence Angle
                n455 = Tangent(1:w1542) -> (0:w1543:dbl)
                n456 = local read "StepWidth (Micos)"() -> (w1550:T6)
                n457 = Build Array(w1543, 0.0 ("element"), 1.0) -> (w1546:dbl[])
                n458 = Multiply(x=w1546, y=w1550) -> (x*y=w1545:T6[])
                n459 = Bundle By Name(cluster=T74 {"State"=enum."MoveRel_all", "Params."=variant} ("element"), "Params."=w1545) -> (w1549:T74)
                n460 = Enqueue Element(queue=w1544, element=w1549) -> (error out=w1540:errorcluster)  [unwired: 2 in, 2 out]
                n461 = call <vilib>:"Clear Errors.vi"("error in (no error)"=w1540) -> ("error out"=w1541:errorcluster)  [unwired: 6 in]
                n462 = call <vilib>:"Release Semaphore.vi"("error in (no error)"=w1541, "semaphore"=w1539) -> ()  [unwired: 4 in, 2 out]
              }
              frame True {
              }
            }
          }
          event "Focus (-)": Value Change {
            n463 = event-data() -> ()  [unwired: 1 in, 1 out]
            n464 = Unbundle By Name(w1554) -> ("Micos"=w1558:refnum<queue>, "AppsLock"=w1555:T63)
            n465 = call <vilib>:"Acquire Semaphore.vi"("ms timeout (-1)"=0, "semaphore"=w1555) -> ("timed out"=w1556:bool, "semaphore out"=w1553:T63)  [unwired: 3 in, 1 out]
            n466 = case shown="False" w1556 {
              tunnel: w1558 -> [w1564 _]
              tunnel: w1553 -> [w1559 _]
              frame False {
                w1562 = -60.0  # Incidence Angle
                n467 = local read "StepWidth (Micos)"() -> (w1570:T6)
                n468 = Tangent(1:w1562) -> (0:w1563:dbl)
                n469 = Build Array(w1563, 0.0 ("element"), -1.0) -> (w1566:dbl[])
                n470 = Multiply(x=w1566, y=w1570) -> (x*y=w1565:T6[])
                n471 = Bundle By Name(cluster=T74 {"State"=enum."MoveRel_all", "Params."=variant} ("element"), "Params."=w1565) -> (w1569:T74)
                n472 = Enqueue Element(queue=w1564, element=w1569) -> (error out=w1560:errorcluster)  [unwired: 2 in, 2 out]
                n473 = call <vilib>:"Clear Errors.vi"("error in (no error)"=w1560) -> ("error out"=w1561:errorcluster)  [unwired: 6 in]
                n474 = call <vilib>:"Release Semaphore.vi"("error in (no error)"=w1561, "semaphore"=w1559) -> ()  [unwired: 4 in, 2 out]
              }
              frame True {
              }
            }
          }
          event "SetFocus": Value Change {
            n475 = event-data() -> ()  [unwired: 1 in, 1 out]
            n476 = Unbundle By Name(w1574) -> ("Micos"=w1573:refnum<queue>)
            n477 = call "SetFocus.vi"() -> ("Aborted?"=w1576:bool, "Destination"=w1575:dbl[])  [unwired: 10 in]
            n478 = case shown="False" w1576 {
              tunnel: w1575 -> [w1578 _]
              tunnel: w1573 -> [w1580 _]
              frame False {
                n479 = property on="Destination" class="Arr (strict)"("Value"=w1578) -> ()  [unwired: 2 in, 2 out]
                n480 = Bundle By Name(cluster=T74 {"State"=enum."MoveAbs_all", "Params."=variant} ("element"), "Params."=w1578) -> (w1577:T74)
                n481 = Enqueue Element(queue=w1580, element=w1577) -> ()  [unwired: 2 in, 3 out]
              }
              frame True {
              }
            }
          }
          event "StopMoving": Value Change {
            n482 = event-data() -> ()  [unwired: 1 in, 1 out]
            n483 = Unbundle By Name(w1588) -> ("Apps"=w1582:refnum<queue>, "Micos"=w1587:refnum<queue>)
            n484 = Enqueue Element(queue=w1582, element=States-AToF."Interrupted_Stop") -> (error out=w1584:errorcluster)  [unwired: 2 in, 2 out]
            n485 = call <vilib>:"Clear Errors.vi"("error in (no error)"=w1584) -> ("error out"=w1583:errorcluster)  [unwired: 6 in]
            n486 = Enqueue Element(queue=w1587, element=T74 {"State"=enum."STOP", "Params."=variant}, error in (no error)=w1583) -> ()  [unwired: 1 in, 3 out]
          }
          event "Home(Micos)": Value Change {
            n487 = event-data() -> ()  [unwired: 1 in, 1 out]
            n488 = Unbundle By Name(w1596) -> ("AppsLock"=w1591:T63, "Micos"=w1592:refnum<queue>)
            n489 = call <vilib>:"Acquire Semaphore.vi"("ms timeout (-1)"=0, "semaphore"=w1591) -> ("timed out"=w1595:bool, "semaphore out"=w1590:T63)  [unwired: 3 in, 1 out]
            n490 = case shown="False" w1595 {
              tunnel: w1592 -> [w1601 _]
              tunnel: T74 {"State"=enum."Origin/Home", "Params."=variant} ("element") -> [w1600 _]
              tunnel: w1590 -> [w1597 _]
              frame False {
                n491 = Enqueue Element(queue=w1601, element=w1600) -> (error out=w1598:errorcluster)  [unwired: 2 in, 2 out]
                n492 = call <vilib>:"Clear Errors.vi"("error in (no error)"=w1598) -> ("error out"=w1599:errorcluster)  [unwired: 6 in]
                n493 = call <vilib>:"Release Semaphore.vi"("error in (no error)"=w1599, "semaphore"=w1597) -> ()  [unwired: 4 in, 2 out]
              }
              frame True {
              }
            }
          }
          event "MoveAbs(Micos)": Value Change {
            n494 = event-data() -> ()  [unwired: 1 in, 1 out]
            n495 = Unbundle By Name(w1612) -> ("AppsLock"=w1609:T63, "Micos"=w1605:refnum<queue>)
            n496 = Bundle By Name(cluster=T74 {"State"=enum."MoveAbs_all", "Params."=variant} ("element"), "Params."="Destination") -> (w1606:T74)
            n497 = property on="MoveAbs(Micos)" class="Bool (strict)"("Value"=FALSE ("MoveAbs(Micos)")) -> ()  [unwired: 2 in, 2 out]
            n498 = call <vilib>:"Acquire Semaphore.vi"("ms timeout (-1)"=0, "semaphore"=w1609) -> ("timed out"=w1610:bool, "semaphore out"=w1604:T63)  [unwired: 3 in, 1 out]
            n499 = case shown="False" w1610 {
              tunnel: w1605 -> [w1617 _]
              tunnel: w1606 -> [w1616 _]
              tunnel: w1604 -> [w1613 _]
              frame False {
                n500 = Enqueue Element(queue=w1617, element=w1616) -> (error out=w1614:errorcluster)  [unwired: 2 in, 2 out]
                n501 = call <vilib>:"Clear Errors.vi"("error in (no error)"=w1614) -> ("error out"=w1615:errorcluster)  [unwired: 6 in]
                n502 = call <vilib>:"Release Semaphore.vi"("error in (no error)"=w1615, "semaphore"=w1613) -> ()  [unwired: 4 in, 2 out]
              }
              frame True {
              }
            }
          }
          event "Position(Micos)": Mouse Down {
            n503 = event-data() -> ("CtlRef"=w1620:refnum<vi>, "Mods.Double Click"=w1621:bool)  [unwired: 1 in]
            n504 = control-ref of="Destination (Micos)"() -> (w1618:refnum<vi>)
            n505 = case shown="True" w1621 {
              tunnel: w1620 -> [_ w1623]
              tunnel: w1618 -> [_ w1622]
              frame False {
              }
              frame True {
                n506 = property on="Property Node" class="Arr (strict)"(reference=w1623) -> ("Value"=w1624:dbl[])  [unwired: 1 in, 2 out]
                n507 = property on="Property Node" class="Arr (strict)"(reference=w1622, "Value"=w1624) -> ()  [unwired: 1 in, 2 out]
              }
            }
          }
          event "Position(ESP)": Mouse Down {
            n508 = event-data() -> ("CtlRef"=w1627:refnum<vi>, "Mods.Double Click"=w1628:bool)  [unwired: 1 in]
            n509 = control-ref of="Destination(ESP)"() -> (w1626:refnum<vi>)
            n510 = case shown="True" w1628 {
              tunnel: w1627 -> [_ w1631]
              tunnel: w1626 -> [_ w1630]
              frame False {
              }
              frame True {
                n511 = property on="Property Node" class="Arr (strict)"(reference=w1631) -> (error out=w1629:errorcluster, "Value"=w1632:dbl[])  [unwired: 1 in, 1 out]
                n512 = property on="Property Node" class="Arr (strict)"(reference=w1630, error in=w1629, "Value"=w1632) -> ()  [unwired: 2 out]
              }
            }
          }
          event "Velocity(Micos)": Value Change {
            n513 = event-data() -> ("NewVal"=w1633:dbl)  [unwired: 1 in]
            n514 = Bundle By Name(cluster=w1635, "Micos.Velocity"=w1633) -> (w1634:T50)
            n515 = Unbundle By Name(w1643) -> ("Micos"=w1638:refnum<queue>)
            n516 = Bundle By Name(cluster=cluster{"Axis":i32, "Velocity":dbl} {"Axis"=1, "Velocity"=0.0}, "Velocity"=w1633) -> (w1639:cluster{"Axis":i32, "Velocity":dbl})
            n517 = Bundle By Name(cluster=T74 {"State"=enum."SetVelocity", "Params."=variant} ("element"), "Params."=w1639) -> (w1641:T74)
            n518 = Enqueue Element(queue=w1638, element=w1641) -> (error out=w1637:errorcluster)  [unwired: 2 in, 2 out]
            n519 = Enqueue Element(queue=w1638, element=T74 {"State"=enum."GetVelocity", "Params."=variant}, error in (no error)=w1637) -> ()  [unwired: 1 in, 3 out]
          }
          event "Accele.(Micos)": Value Change {
            n520 = event-data() -> ("NewVal"=w1644:dbl)  [unwired: 1 in]
            n521 = Bundle By Name(cluster=w1646, "Micos.Acceleration"=w1644) -> (w1645:T50)
            n522 = Bundle By Name(cluster=cluster{"Axis":i32, "Acceleration":dbl} {"Axis"=1, "Acceleration"=0.0}, "Acceleration"=w1644) -> (w1650:cluster{"Axis":i32, "Acceleration":dbl})
            n523 = Unbundle By Name(w1654) -> ("Micos"=w1653:refnum<queue>)
            n524 = Bundle By Name(cluster=T74 {"State"=enum."SetAcceleration", "Params."=variant} ("element"), "Params."=w1650) -> (w1655:T74)
            n525 = Enqueue Element(queue=w1653, element=w1655) -> (queue out=w1649:refnum<queue>, error out=w1648:errorcluster)  [unwired: 2 in, 1 out]
            n526 = Enqueue Element(queue=w1649, element=T74 {"State"=enum."GetAcceleration", "Params."=variant}, error in (no error)=w1648) -> ()  [unwired: 1 in, 3 out]
          }
          event Value Change {
            # "Convert  AnalogDisc's TriggerPosition to Gage's TriggerDelay"
            n527 = event-data() -> ("NewVal"=w1656:T20)  [unwired: 1 in]
            n528 = Unbundle By Name(w1682) -> ("ProcCore_CtrlQueue"=w1675:refnum<queue>, "MainDAQCoreQueue"=w1685:refnum<queue>)
            n529 = Bundle By Name(cluster=w1658, "AnalogDisc_Config"=w1656) -> (w1657:T50)
            n530 = Bundle By Name(cluster=T60 {"DWF States"=enum."SetAll_AcquChTrig_", "Variant"=variant} ("element"), "Variant"=w1656) -> (w1683:T60)
            n531 = Bundle By Name(cluster=T60 {"DWF States"=enum."GetConfig_", "Variant"=variant} ("element"), "Variant"=w1677) -> (w1679:T60)
            n532 = Enqueue Element(queue=w1685, element=w1683) -> (queue out=w1681:refnum<queue>)  [unwired: 2 in, 2 out]
            n533 = Enqueue Element(queue=w1681, element=w1679) -> (error out=w1678:errorcluster)  [unwired: 2 in, 2 out]
            n534 = Dequeue Element(queue=w1677, timeout in ms (-1)=-1, error in (no error)=w1678) -> (element=w1676:T20)  [unwired: 3 out]
            n535 = Unbundle By Name(w1676) -> ("Acqusition.Freq(Hz,SampleRate)"=w1668:dbl, "Acqusition.BufferSize"=w1670:i32, "Trigger.Position/Delay(s)"=w1667:dbl)
            n536 = Quotient & Remainder(x=w1670, y=2) -> (floor(x/y)=w1664:i32)  [unwired: 1 out]
            n537 = Reciprocal(x=w1668) -> (1/x=w1666:dbl)
            n538 = Multiply(x=w1666, y=w1664) -> ()  [unwired: 1 out]
            n539 = Divide(x=w1667, y=w1666) -> (x/y=w1663:dbl)
            n540 = Negate(x=w1664) -> (-x=w1665:i32)
            n541 = Subtract(x=w1665, y=w1663) -> (x-y=w1662:dbl)
            n542 = Bundle By Name(cluster=T66 {"TrigDelay"=0.0, "Offset"=0, "Resolution"=-32768, "Range (mV)"=0, "Sample Rate"=100000000.0, "Depth"=16384.0, "Segments"=1} ("DAQParams"), "Sample Rate"=w1668, "Depth"=w1670, "TrigDelay"=w1662) -> (w1672:T66)
            n543 = Bundle By Name(cluster=T75 {"Command"=enum."SetAcquisitionParams", "Params"=variant} ("element"), "Params"=w1672) -> (w1673:T75)
            n544 = Enqueue Element(queue=w1675, element=w1673) -> (queue out=w1661:refnum<queue>)  [unwired: 2 in, 2 out]
            n545 = Enqueue Element(queue=w1661, element=T75 {"Command"=enum."CalcMzArray", "Params"=variant}) -> ()  [unwired: 2 in, 3 out]
          }
          event Value Change {
            n546 = event-data() -> ("NewVal"=w1686:T19, "NewVal.Acquisition.Trigger Delay"=w1700:dbl, "NewVal.Channels"=w1699:T89)  [unwired: 1 in]
            n547 = Unbundle By Name(w1718) -> ("ProcCore_CtrlQueue"=w1713:refnum<queue>, "MainDAQCoreQueue"=w1720:refnum<queue>)
            n548 = Bundle By Name(cluster=T60 {"DWF States"=enum."SetAll_AcquChTrig_", "Variant"=variant} ("element"), "Variant"=w1686) -> (w1691:T60)
            n549 = Build Array(T60 {"DWF States"=enum."GetAll_AcquChTrig", "Variant"=variant} ("element"), T60 {"DWF States"=enum."fStart", "Variant"=variant} ("element"), T60 {"DWF States"=enum."fConfigurate", "Variant"=variant} ("element"), w1691) -> (w1695:T60[])
            n550 = Index Array(array=w1699) -> (element=w1698:T90)  [unwired: 1 in]
            n551 = Reverse 1D Array(array=w1695) -> (reversed array=w1690:T60[])
            n552 = for {
              tunnel: w1690 -> [w1722] mode=indexing
              shift-right: [w1721] -> w1694
              shift-left: w1720 -> [w1723]
              n553 = Enqueue Element(queue=w1723, element=w1722) -> (queue out=w1721:refnum<queue>)  [unwired: 2 in, 2 out]
            }
            n554 = Unbundle By Name(w1698) -> ("Range"=w1697:u32)
            n555 = local read "Signal Segment"() -> (w1702:T3)
            n556 = Bundle By Name(cluster=T60 {"DWF States"=enum."GetConfig_", "Variant"=variant} ("element"), "Variant"=w1703) -> (w1716:T60)
            n557 = Bundle By Name(cluster=w1702, "TrigDelay"=w1700, "DAQ_Range"=w1697) -> (w1701:T3)
            n558 = Enqueue Element(queue=w1694, element=w1716) -> (error out=w1715:errorcluster)  [unwired: 2 in, 2 out]
            n559 = Dequeue Element(queue=w1703, timeout in ms (-1)=-1, error in (no error)=w1715) -> (element=w1714:T19)  [unwired: 3 out]
            n560 = Unbundle By Name(w1714) -> ("Acquisition.Sample Rate"=w1707:dbl, "Acquisition.Depth"=w1708:dbl, "Acquisition.Trigger Delay"=w1704:dbl)
            n561 = local write "Signal Segment"(w1701) -> ()
            n562 = Bundle By Name(cluster=T66 {"TrigDelay"=0.0, "Offset"=0, "Resolution"=-32768, "Range (mV)"=0, "Sample Rate"=100000000.0, "Depth"=16384.0, "Segments"=1} ("DAQParams"), "Sample Rate"=w1707, "Depth"=w1708, "TrigDelay"=w1704) -> (w1710:T66)
            n563 = Bundle By Name(cluster=T75 {"Command"=enum."SetAcquisitionParams", "Params"=variant} ("element"), "Params"=w1710) -> (w1711:T75)
            n564 = Enqueue Element(queue=w1713, element=w1711) -> (queue out=w1706:refnum<queue>)  [unwired: 2 in, 2 out]
            n565 = Bundle By Name(cluster=w1688, "Gage_Config"=w1686) -> (w1687:T50)
            n566 = Enqueue Element(queue=w1706, element=T75 {"Command"=enum."CalcMzArray", "Params"=variant}) -> ()  [unwired: 2 in, 3 out]
          }
          event Value Change {
            # "Removed Configs=>Instrument\nSettings, since GenericDAQ settings need not \nto be saved"
            n567 = event-data() -> ("NewVal"=w1727:T14, "NewVal.Channels"=w1739:cluster{"Range":u32, "DC Offset":i32}[])  [unwired: 1 in]
            n568 = Unbundle By Name(w1755) -> ("ProcCore_CtrlQueue"=w1750:refnum<queue>, "MainDAQCoreQueue"=w1757:refnum<queue>)
            n569 = Bundle By Name(cluster=T60 {"DWF States"=enum."SetAll_AcquChTrig_", "Variant"=variant} ("element"), "Variant"=w1727) -> (w1731:T60)
            n570 = Build Array(T60 {"DWF States"=enum."GetAll_AcquChTrig", "Variant"=variant} ("element"), T60 {"DWF States"=enum."fStart", "Variant"=variant} ("element"), T60 {"DWF States"=enum."fConfigurate", "Variant"=variant} ("element"), w1731) -> (w1735:T60[])
            n571 = Index Array(array=w1739) -> (element=w1738:cluster{"Range":u32, "DC Offset":i32})  [unwired: 1 in]
            n572 = Reverse 1D Array(array=w1735) -> (reversed array=w1730:T60[])
            n573 = for {
              tunnel: w1730 -> [w1759] mode=indexing
              shift-right: [w1758] -> w1734
              shift-left: w1757 -> [w1760]
              n574 = Enqueue Element(queue=w1760, element=w1759) -> (queue out=w1758:refnum<queue>)  [unwired: 2 in, 2 out]
            }
            n575 = Unbundle By Name(w1738) -> ("Range"=w1737:u32)
            n576 = local read "Signal Segment"() -> (w1741:T3)
            n577 = Bundle By Name(cluster=T60 {"DWF States"=enum."GetConfig_", "Variant"=variant} ("element"), "Variant"=w1725) -> (w1753:T60)
            n578 = Bundle By Name(cluster=w1741, "TrigDelay"=0.0, "DAQ_Range"=w1737) -> (w1740:T3)
            n579 = Enqueue Element(queue=w1734, element=w1753) -> (error out=w1752:errorcluster)  [unwired: 2 in, 2 out]
            n580 = Dequeue Element(queue=w1725, timeout in ms (-1)=-1, error in (no error)=w1752) -> (element=w1751:T14)  [unwired: 3 out]
            n581 = Unbundle By Name(w1751) -> ("Acquisition.Sample Rate"=w1744:dbl, "Acquisition.Depth"=w1745:dbl)
            n582 = local write "Signal Segment"(w1740) -> ()
            n583 = Bundle By Name(cluster=T66 {"TrigDelay"=0.0, "Offset"=0, "Resolution"=-32768, "Range (mV)"=0, "Sample Rate"=100000000.0, "Depth"=16384.0, "Segments"=1} ("DAQParams"), "Sample Rate"=w1744, "Depth"=w1745, "TrigDelay"=0.0) -> (w1747:T66)
            n584 = Bundle By Name(cluster=T75 {"Command"=enum."SetAcquisitionParams", "Params"=variant} ("element"), "Params"=w1747) -> (w1748:T75)
            n585 = Enqueue Element(queue=w1750, element=w1748) -> (queue out=w1743:refnum<queue>)  [unwired: 2 in, 2 out]
            n586 = Enqueue Element(queue=w1743, element=T75 {"Command"=enum."CalcMzArray", "Params"=variant}) -> ()  [unwired: 2 in, 3 out]
          }
          event Value Change {
            n587 = event-data() -> ("NewVal"=w1764:T1)  [unwired: 1 in]
            n588 = Unbundle By Name(w1763) -> ("ProcCore_CtrlQueue"=w1762:refnum<queue>)
            n589 = local read "Signal Segment"() -> (w1766:T3)
            n590 = Bundle By Name(cluster=w1766, "Average#"=w1764) -> (w1765:T3)
            n591 = Bundle By Name(cluster=T75 {"Command"=enum."Initialize", "Params"=variant} ("element"), "Command"=ProcessStates."Initialize") -> (w1768:T75)
            n592 = local write "Signal Segment"(w1765) -> ()
            n593 = Enqueue Element(queue=w1762, element=w1768) -> ()  [unwired: 2 in, 3 out]
          }
          event "Rep.Rate (BNC)": Value Change {
            n594 = event-data() -> ("NewVal"=w1770:dbl)  [unwired: 1 in]
            n595 = Unbundle By Name(w1774) -> ("ProcCore_CtrlQueue"=w1773:refnum<queue>)
            n596 = Bundle By Name(cluster=T75 {"Command"=enum."Initialize", "Params"=variant} ("element"), "Params"=w1770, "Command"=ProcessStates."ChangeRepRate") -> (w1776:T75)
            n597 = Enqueue Element(queue=w1773, element=w1776) -> ()  [unwired: 2 in, 3 out]
            n598 = Bundle By Name(cluster=w1772, "Timing(LDPI).RepRate(Hz)"=w1770) -> (w1771:T50)
          }
          event "DisplayIncrement": Value Change {
            n599 = event-data() -> ("NewVal"=w1781:u32)  [unwired: 1 in]
            n600 = Unbundle By Name(w1780) -> ("ProcCore_CtrlQueue"=w1779:refnum<queue>)
            n601 = Bundle By Name(cluster=T75 {"Command"=enum."Initialize", "Params"=variant} ("element"), "Params"=w1781, "Command"=ProcessStates."ChangeDisplayIncrement") -> (w1783:T75)
            n602 = Enqueue Element(queue=w1779, element=w1783) -> ()  [unwired: 2 in, 3 out]
          }
          event "Cali.": Value Change {
            n603 = event-data() -> ("NewVal"=w1785:dbl[])  [unwired: 1 in]
            n604 = Unbundle By Name(w1790) -> ("ProcCore_CtrlQueue"=w1789:refnum<queue>)
            n605 = local read "Signal Segment"() -> (w1792:T3)
            n606 = Bundle By Name(cluster=w1792, "Calibr."=w1785) -> (w1791:T3)
            n607 = local write "Signal Segment"(w1791) -> ()
            n608 = Bundle By Name(cluster=T75 {"Command"=enum."CalcMzArray", "Params"=variant} ("element"), "Params"=w1785) -> (w1788:T75)
            n609 = Enqueue Element(queue=w1789, element=w1788) -> ()  [unwired: 2 in, 3 out]
            n610 = Bundle By Name(cluster=w1787, "Cali."=w1785) -> (w1786:T50)
          }
          event "GraphEnable (A)", "GraphEnable (B)", "IncrementUpdate(A)", "IncrementUpdate(B)", "Resolution(B)", "Resolution(A)": Value Change {
            n611 = event-data() -> ()  [unwired: 1 in, 2 out]
            n612 = Unbundle By Name(w1796) -> ("ProcCore_CtrlQueue"=w1795:refnum<queue>)
            n613 = Enqueue Element At Opposite End(queue=w1795, element=T75 {"Command"=enum."SetGraphsEnable", "Params"=variant}) -> ()  [unwired: 2 in, 3 out]
          }
          event "Binning(A)", "Binning(B)", "BinWidth (A)", "BinWidth (B)": Value Change {
            n614 = event-data() -> ()  [unwired: 1 in, 2 out]
            n615 = Unbundle By Name(w1800) -> ("ProcCore_CtrlQueue"=w1799:refnum<queue>)
            n616 = control-ref of="Binning(B)"() -> (w1809:refnum<vi>)
            n617 = control-ref of="Binning(A)"() -> (w1808:refnum<vi>)
            n618 = property class="Bool (strict)"(reference=w1809) -> ("Value"=w1807:bool)  [unwired: 1 in, 2 out]
            n619 = property class="Bool (strict)"(reference=w1808) -> ("Value"=w1806:bool)  [unwired: 1 in, 2 out]
            n620 = Enqueue Element At Opposite End(queue=w1799, element=T75 {"Command"=enum."SetGraphsEnable", "Params"=variant}) -> ()  [unwired: 2 in, 3 out]
            n621 = control-ref of="Snap"() -> (w1805:refnum<vi>)
            n622 = And(x=w1807, y=w1806) -> (x .and. y?=w1802:bool)
            n623 = Select(t=T49."Disabled and Grayed Out" ("Disabled"), s=w1802, f=T49."Enabled" ("Disabled")) -> (s? t:f=w1801:T49)
            n624 = property class="Bool (strict)"(reference=w1805, "DisabledEnum"=w1801) -> ()  [unwired: 1 in, 2 out]
          }
          event "TopLine", "Baseline", "Threshold", "ZeroOffsetCorrection": Value Change {
            # "Legacy Code, do not follow"
            n625 = event-data() -> ("OldVal"=w1815:variant)  [unwired: 1 in]
            n626 = Unbundle By Name(w1814) -> ("ProcCore_CtrlQueue"=w1813:refnum<queue>)
            n627 = case shown="Default" "Processing Mode" {
              selector: "Processing Mode" -> [w1827 w1837]
              tunnel: w1813 -> [w1835 _]
              tunnel: w1815 -> [_ w1839]
              tunnel: w1812 -> [w1823 w1836]
              tunnel: [w1822 w1836] -> w1811
              frame Default {
                n628 = local read "Processing Mode"() -> (w1817:T4)
                n629 = Build Array("TopLine", "Threshold", "Baseline", "ZeroOffsetCorrection") -> (w1829:dbl[])
                n630 = local read "Threshold"() -> (w1824:dbl)
                n631 = To Variant(anything=w1829) -> (Variant=w1831:variant)
                n632 = Bundle(cluster=cluster{"Processing Mode":T4, "Variant":variant} {"Processing Mode"=enum."None", "Variant"=variant}, "Processing Mode"=w1827, "Variant"=w1831) -> (w1828:cluster{"Processing Mode":T4, "Variant":variant})
                n633 = Bundle By Name(cluster=T75 {"Command"=enum."Initialize", "Params"=variant} ("element"), "Command"=ProcessStates."SetFilterParams", "Params"=w1828) -> (w1833:T75)
                n634 = local read "Signal Segment"() -> (w1826:T3)
                n635 = Enqueue Element(queue=w1835, element=w1833) -> ()  [unwired: 2 in, 3 out]
                n636 = Bundle By Name(cluster=w1826, "ProcMode"=w1817, "Threshold"=w1824) -> (w1825:T3)
                n637 = Bundle By Name(cluster=w1823, "ProcessMethod.TopLine"="TopLine", "ProcessMethod.Threshold"="Threshold", "ProcessMethod.Baseline"="Baseline", "ProcessMethod.ZeroOffset"="ZeroOffsetCorrection", "ProcessMethod.Processing Mode"=w1817) -> (w1822:T50)
                n638 = local write "Signal Segment"(w1825) -> ()
              }
              frame "SetFilter" {
                n639 = Variant To Data(type=w1837, Variant=w1839) -> (data=w1838:T4)  [unwired: 1 in, 1 out]
                n640 = control-ref of="Processing Mode"() -> (w1840:refnum<vi>)
                n641 = property class="Enum (strict)"(reference=w1840, "Value"=w1838) -> ()  [unwired: 1 in, 2 out]
              }
            }
          }
          event "Switch(SDG_II)": Value Change {
            n642 = event-data() -> ()  [unwired: 1 in, 1 out]
            n643 = Unbundle By Name(w1843) -> ("SDG_ii"=w1842:refnum<queue>)
            n644 = Select(t=T70 {"State"=enum."Turn On", "Parameter"=0.0} ("element"), s="Switch(SDG_II)", f=T70 {"State"=enum."Tun OFF", "Parameter"=0.0} ("element")) -> (s? t:f=w1844:T70)
            n645 = Enqueue Element(queue=w1842, element=w1844) -> ()  [unwired: 2 in, 3 out]
          }
          event "Mode(SDG_II)": Value Change {
            n646 = event-data() -> ()  [unwired: 1 in, 1 out]
            n647 = Unbundle By Name(w1851) -> ("SDG_ii"=w1850:refnum<queue>)
            n648 = Select(t=T70 {"State"=enum."Continuous", "Parameter"=0.0} ("element"), s="Mode(SDG_II)", f=T70 {"State"=enum."Single Shot", "Parameter"=0.0} ("element")) -> (s? t:f=w1853:T70)
            n649 = Enqueue Element(queue=w1850, element=w1853) -> ()  [unwired: 2 in, 3 out]
            n650 = Unbundle By Name(w1849) -> ("InstrumentMode.LaserCtrlMethod"=w1848:T17)
            n651 = case shown="\"SDG_II\"" w1848 {
              tunnel: "Mode(SDG_II)" -> [_ w1856]
              frame Default {
              }
              frame "SDG_II" {
                n652 = property on="LaserON" class="Bool (strict)"("Value"=w1856) -> ()  [unwired: 2 in, 2 out]
              }
            }
          }
          event "LaserON": Value Change {
            n653 = event-data() -> ()  [unwired: 1 in, 2 out]
            n654 = Unbundle By Name(w1857) -> ("InstrumentMode.LaserCtrlMethod"=w1859:T17)
            n655 = case shown="\"SRS_DG535\"" w1859 {
              tunnel: "LaserON" -> [w1861 w1862 w1863]
              frame "SDG_II" {
                n656 = property on="Mode(SDG_II)" class="Bool (strict)"("Val(Sgnl)"=w1861) -> ()  [unwired: 2 in, 2 out]
              }
              frame "BNC" {
                n657 = property on="BNC On/Off" class="Bool (strict)"("Val(Sgnl)"=w1862) -> ()  [unwired: 2 in, 2 out]
              }
              frame "SRS_DG535" {
                n658 = property on="SRS On/Off" class="Bool (strict)"("Val(Sgnl)"=w1863) -> ()  [unwired: 2 in, 2 out]
              }
            }
            n659 = disable-structure shown="Disabled" {
              disable-tunnel: "LaserON" -> [w1860 _]
              frame Disabled {
                # "^For Emulation only"
                n660 = global write "Emu_CoreDAQ_Globle.vi" "Enable"(w1860) -> ()
              }
              frame Enabled {
              }
            }
          }
          event "ManlTrig(SDG)": Value Change {
            n661 = event-data() -> ()  [unwired: 1 in, 1 out]
            n662 = Unbundle By Name(w1866) -> ("SDG_ii"=w1865:refnum<queue>)
            n663 = Enqueue Element(queue=w1865, element=T70 {"State"=enum."ManualTrigger", "Parameter"=0.0}) -> ()  [unwired: 2 in, 3 out]
          }
          event "Meander", "DepthProfile", "Set dbl pulse Delay", "Meander (ESP)", "DelayScan", "BeamProfiling(ESP)": Value Change {
            w1880 = T71[] [enum."Meander_MCS", enum."DepthProfiling", enum."DelayScan", enum."Set_2PulseDelay", enum."Meander_Npt", enum."KnifeEdgeExpt_Npt"] items=["Initialize", "Idle", "CalcMzArray", "Meander_SGL_MCS", "Meander_MCS", "CleanSurface", "Meander_Npt", "Meander_SGL_Npt", "KnifeEdgeExpt", "KnifeEdgeExpt_Npt", "Imaging_Micos", "Imaging_ESP", "DepthProfiling", "Set_2PulseDelay", "DelayScan", "PeakSearch", "ExportOrigin", "Save Settings", "Load Settings", "Save as Default", "Load Default", "EnergyCalibration", "Quit", "Interrupted_Stop", "Quit_SubProgram", "StepMove_Joystick", "ContMove_Joystick", "Stop_Joystick", "Check_AppsLock", "Return_Status", "DepthProfile_RT", "UpdateInstruStates", "InstruOptimizer_static", "InstruOptimizer_dynamic", "DepthProfiling(3D)"]
            n664 = event-data() -> ()  [unwired: 1 in, 1 out]
            n665 = Unbundle By Name(w1882) -> ("Apps"=w1881:refnum<queue>)
            n666 = Build Array("Meander", "DepthProfile", "DelayScan", "Set dbl pulse Delay", "Meander (ESP)", "BeamProfiling(ESP)") -> (w1877:bool[])
            n667 = global read "Position_Micos.vi" "Moving(Micos)"() -> (w1870:bool)
            n668 = global read "Position_ESP300.vi" "Moving"() -> (w1868:bool)
            n669 = Or(x=w1870, y=w1868) -> (x .or. y?=w1869:bool)
            n670 = Build Array(w1870, w1870, w1869, w1868, w1868, w1870) -> (w1871:bool[])
            n671 = for {
              tunnel: w1881 -> [w1887]
              tunnel: w1880 -> [w1885] mode=indexing
              tunnel: w1877 -> [w1884] mode=indexing
              tunnel: w1871 -> [w1883] mode=indexing
              n672 = Compound Arithmetic op=AND(invert w1883, w1884) -> (w1886:bool)
              n673 = case shown="True" w1886 {
                tunnel: w1887 -> [_ w1889]
                tunnel: w1885 -> [_ w1888]
                frame False {
                }
                frame True {
                  n674 = Enqueue Element(queue=w1889, element=w1888) -> ()  [unwired: 2 in, 3 out]
                }
              }
            }
          }
          event "Pause": Value Change {
            n675 = event-data() -> ()  [unwired: 1 in, 1 out]
            n676 = global write "PauseMeander.vi" "Pause Meaner"("Pause") -> ()
            n677 = property on="Pause" class="Bool (strict)"("Blinking"="Pause") -> ()  [unwired: 2 in, 2 out]
          }
          event "BNC On/Off": Value Change {
            n678 = event-data() -> ()  [unwired: 1 in, 2 out]
            n679 = Unbundle By Name(w1899) -> ("BNC"=w1898:refnum<queue>)
            n680 = Select(t=T84 {"State"=enum."Run", "Para."=variant} ("element"), s="BNC On/Off", f=T84 {"State"=enum."Stop", "Para."=variant} ("element")) -> (s? t:f=w1895:T84)
            n681 = Enqueue Element(queue=w1898, element=w1895) -> ()  [unwired: 2 in, 3 out]
            n682 = Unbundle By Name(w1893) -> ("InstrumentMode.LaserCtrlMethod"=w1894:T17)
            n683 = case shown="\"BNC\"" w1894 {
              tunnel: "BNC On/Off" -> [_ w1900]
              frame Default {
              }
              frame "BNC" {
                n684 = property on="LaserON" class="Bool (strict)"("Value"=w1900) -> ()  [unwired: 2 in, 2 out]
              }
            }
          }
          event "Set Mode": Value Change {
            n685 = event-data() -> ()  [unwired: 1 in, 1 out]
            n686 = Unbundle By Name(w1922) -> ("BNC"=w1921:refnum<queue>)
            n687 = Unbundle By Name(w1918) -> ("InstrumentMode.LaserCtrlMethod"=w1920:T17)
            n688 = property on="BNC On/Off" class="Bool (strict)"("Value"=FALSE ("BNC Switch")) -> ()  [unwired: 2 in, 2 out]
            n689 = case shown="\"BNC\"" w1920 {
              tunnel: FALSE -> [_ w1938]
              frame Default {
              }
              frame "BNC" {
                n690 = property on="LaserON" class="Bool (strict)"("Value"=w1938) -> ()  [unwired: 2 in, 2 out]
              }
            }
            n691 = Bundle By Name(cluster=T87 {"Rep.Rate"=0.0, "Sys Ext Mode"=enum."Triggered", "Mode"=enum."Normal"}, "Mode"="Mode (BNC)", "Rep.Rate"="Rep.Rate (BNC)", "Sys Ext Mode"="Trigger Mode (BNC)") -> (w1914:T87)
            n692 = Bundle By Name(cluster=w1918, "BNC_Config.System.Mode"="Mode (BNC)", "BNC_Config.System.Rep.Rate"="Rep.Rate (BNC)", "BNC_Config.System.Sys Ext Mode"="Trigger Mode (BNC)") -> (w1905:T50)
            n693 = To Variant(anything=w1914) -> (Variant=w1915:variant)
            n694 = Bundle By Name(cluster=T84 {"State"=enum."Set System", "Para."=variant} ("element"), "Para."=w1915) -> (w1913:T84)
            n695 = Enqueue Element(queue=w1921, element=w1913) -> (error out=w1916:errorcluster)  [unwired: 2 in, 2 out]
            n696 = Unbundle By Name(w1905) -> ("BNC_Config.Channels"=w1904:T33[])
            n697 = for {
              N -> [w1925]
              tunnel: w1921 -> [w1937]
              tunnel: "Channels Enable Status" -> [w1927] mode=indexing
              shift-right: [w1930] -> _
              shift-left: w1916 -> [w1936]
              tunnel: w1904 -> [w1928] mode=indexing
              tunnel: [w1926] -> w1903 mode=indexing
              tunnel: [w1925] -> w1901
              i -> [w1931]
              n698 = Increment(x=w1931) -> (x+1=w1929:i32)
              n699 = Bundle By Name(cluster=T37 {"Channel"=0, "Enable"=FALSE}, "Channel"=w1929, "Enable"=w1927) -> (w1933:T37)
              n700 = Bundle By Name(cluster=w1928, "C-Enables.Enable"=w1927) -> (w1926:T33)
              n701 = Bundle By Name(cluster=T84 {"State"=enum."Set C-Enable", "Para."=variant} ("element"), "Para."=w1933) -> (w1934:T84)
              n702 = Enqueue Element(queue=w1937, element=w1934, error in (no error)=w1936) -> (error out=w1930:errorcluster)  [unwired: 1 in, 2 out]
            }
            n703 = in-place {
              in-place-border: w1903 -> [w1923]
              n704 = in-place-split #4(w1904, w1901) -> (w1924:T33[])  [unwired: 1 out]
              n705 = in-place-split #4(w1923, w1924) -> (w1902:T33[])  [unwired: 1 out]
            }
            n706 = Bundle By Name(cluster=w1905, "BNC_Config.Channels"=w1902) -> (w1917:T50)
          }
          event "Delay B", "Width A", "Width B", "Delay A": Value Change {
            # "legacy, need improvement"
            n707 = event-data() -> ()  [unwired: 1 in, 2 out]
            n708 = Unbundle By Name(w1948) -> ("BNC"=w1947:refnum<queue>)
            n709 = Unbundle By Name(w1943) -> ("BNC_Config.Channels"=w1942:T33[])
            n710 = Build Array("Delay A", "Delay B") -> (w1946:dbl[])
            n711 = Build Array("Width A", "Width B") -> (w1945:dbl[])
            n712 = for {
              N -> [w1955]
              tunnel: w1947 -> [w1966]
              tunnel: w1946 -> [w1961] mode=indexing
              tunnel: w1945 -> [w1960] mode=indexing
              tunnel: w1942 -> [w1958] mode=indexing
              tunnel: [w1956] -> w1939 mode=indexing
              tunnel: [w1955] -> w1940
              i -> [w1962]
              w1957 = T35 {"Channel"=0, "Delay"=0.0, "Width"=0.0}  # Set C-Mode
              n713 = Increment(x=w1962) -> (x+1=w1959:i32)
              n714 = Bundle By Name(cluster=w1957, "Channel"=w1959, "Delay"=w1961, "Width"=w1960) -> (w1963:T35)
              n715 = Bundle By Name(cluster=T84 {"State"=enum."Set C-Mode", "Para."=variant} ("element"), "Para."=w1963) -> (w1964:T84)
              n716 = Bundle By Name(cluster=w1958, "C-Mode"=w1957) -> (w1956:T33)
              n717 = Enqueue Element(queue=w1966, element=w1964) -> ()  [unwired: 2 in, 3 out]
            }
            n718 = in-place {
              in-place-border: w1939 -> [w1953]
              n719 = in-place-split #5(w1942, w1940) -> (w1954:T33[])  [unwired: 1 out]
              n720 = in-place-split #5(w1953, w1954) -> (w1941:T33[])  [unwired: 1 out]
            }
            n721 = Bundle By Name(cluster=w1943, "BNC_Config.Channels"=w1941) -> (w1944:T50)
          }
          event "Ch_A", "Ch_B", "Ch_C", "Ch_D": Value Change {
            n722 = event-data() -> ()  [unwired: 1 in, 2 out]
            n723 = Unbundle By Name(w1978) -> ("SRS DG535"=w1977:refnum<queue>)
            n724 = property on="DG535_Configs" class="Clust (strict)"() -> ("Value"=w1970:T48)  [unwired: 2 in, 2 out]
            n725 = Build Array("Ch_A", "Ch_B", "Ch_C", "Ch_D") -> (w1972:dbl[])
            n726 = Unbundle By Name(w1970) -> ("Delays"=w1971:T28[])
            n727 = for {
              tunnel: w1977 -> [w1985]
              tunnel: w1972 -> [w1981] mode=indexing
              shift-right: [w1983] -> _
              shift-left: _ -> [w1982]
              tunnel: w1971 -> [w1980] mode=indexing
              tunnel: [w1979] -> w1967 mode=indexing
              n728 = call-poly <userlib>:"Data Changed__ogtk.vi"("DBL"=w1981) -> ("Changed"=w1984:bool)
              n729 = case shown="True" w1984 {
                tunnel: w1985 -> [_ w1998]
                tunnel: [w1987 w1995] -> w1983
                tunnel: w1982 -> [w1987 w1994]
                tunnel: w1981 -> [_ w1993]
                tunnel: w1980 -> [w1986 w1991]
                tunnel: [w1986 w1988] -> w1979
                frame False {
                }
                frame True {
                  n730 = Unbundle By Name(w1991) -> ("Channel"=w1990:T29, "Sync To"=w1989:T29)
                  n731 = Bundle By Name(cluster=T28 {"Channel"=enum."A Output", "Sync To"=enum."T0 Output", "Delay"=0.0}, "Channel"=w1990, "Sync To"=w1989, "Delay"=w1993) -> (w1988:T28)
                  n732 = Bundle By Name(cluster=T82 {"State"=enum."Set Delay", "Para."=variant} ("element"), "Para."=w1988) -> (w1996:T82)
                  n733 = Enqueue Element(queue=w1998, element=w1996, error in (no error)=w1994) -> (error out=w1995:errorcluster)  [unwired: 1 in, 2 out]
                }
              }
            }
            n734 = Bundle By Name(cluster=w1969, "DG535.Delays"=w1967) -> (w1968:T50)
          }
          event "Delay(LDI-Rej.)", "Delay(PI)": Value Change {
            n735 = event-data() -> ()  [unwired: 1 in, 1 out]
            n736 = Unbundle By Name(w2004) -> ("Timing(LDPI).NoDelayOffset"=w2003:dbl, "InstrumentMode.InstruMode"=w2002:T18)
            n737 = Bundle By Name(cluster=w2004, "Timing(LDPI).Delay(PI)"="Delay(PI)", "Timing(LDPI).Delay(Rejection)"="Delay(LDI-Rej.)") -> (w2001:T50)
            n738 = case shown="\"fsLDPI\"" w2002 {
              tunnel: "Delay(PI)" -> [w2011 w2018 w2025 _ _ _]
              tunnel: "Delay(LDI-Rej.)" -> [w2010 w2017 w2024 _ _ _]
              tunnel: w2003 -> [w2005 w2016 w2023 _ _ _]
              frame "fsLDPI" {
                # "NoDelayOffset: 99.8095m"
                # "Ch_A=> 0 delay offset\nCh_B => ND:YAG flashlamp\n-CD HV pulser\n\nND:YAG Sync => Gage Trig in"
                n739 = First Call?() -> (First Call?: T/F=w2006:bool)
                n740 = Add(x=w2011, y=w2010) -> (x+y=w2008:dbl)
                n741 = case shown="True" w2006 {
                  tunnel: w2005 -> [_ w2012]
                  frame False {
                  }
                  frame True {
                    n742 = control-ref of="Ch_A"() -> (w2014:refnum<vi>)
                    n743 = control-ref of="Ch_C"() -> (w2013:refnum<vi>)
                    n744 = property class="DigNum (strict)"(reference=w2014, "Val(Sgnl)"=w2012) -> ()  [unwired: 1 in, 2 out]
                    n745 = property class="DigNum (strict)"(reference=w2013, "Val(Sgnl)"=0.0 ("Value (Signaling)")) -> ()  [unwired: 1 in, 2 out]
                  }
                }
                n746 = control-ref of="Ch_B"() -> (w2007:refnum<vi>)
                n747 = control-ref of="Ch_D"() -> (w2009:refnum<vi>)
                n748 = property class="DigNum (strict)"(reference=w2009, "Val(Sgnl)"=w2008) -> ()  [unwired: 1 in, 2 out]
                n749 = property class="DigNum (strict)"(reference=w2007, "Val(Sgnl)"=w2011) -> ()  [unwired: 1 in, 2 out]
              }
              frame "nsLDPI" {
                # "NoDelayOffset: 0.0001766"
                # "T0 => ND:YAG flashlap, inverted, High-Z\nCh_A => Explorer trig in, inverted\nCh_B => \nCh_D => HV pulser rise\n-CD => HV pulse"
                n750 = Add(x=w2018, y=w2017) -> (x+y=w2021:dbl)
                n751 = Subtract(x=w2016, y=w2018) -> (x-y=w2020:dbl)
                n752 = control-ref of="Ch_A"() -> (w2019:refnum<vi>)
                n753 = control-ref of="Ch_D"() -> (w2022:refnum<vi>)
                n754 = property class="DigNum (strict)"(reference=w2022, "Val(Sgnl)"=w2021) -> ()  [unwired: 1 in, 2 out]
                n755 = property class="DigNum (strict)"(reference=w2019, "Val(Sgnl)"=w2020) -> ()  [unwired: 1 in, 2 out]
              }
              frame "nsLD-fsPI" {
                (unwired) 0.0009859
                n756 = Negate(x=w2025) -> (-x=w2026:dbl)
                n757 = Add(x=0.001, y=w2024) -> (x+y=w2032:dbl)
                n758 = control-ref of="Ch_A"() -> (w2029:refnum<vi>)
                n759 = control-ref of="Ch_B"() -> (w2031:refnum<vi>)
                n760 = control-ref of="Ch_D"() -> (w2033:refnum<vi>)
                n761 = control-ref of="Ch_C"() -> (w2030:refnum<vi>)
                n762 = property class="DigNum (strict)"(reference=w2033, "Val(Sgnl)"=w2032) -> ()  [unwired: 1 in, 2 out]
                n763 = property class="DigNum (strict)"(reference=w2030, "Val(Sgnl)"=5e-05 ("Value (Signaling)")) -> ()  [unwired: 1 in, 2 out]
                n764 = property class="DigNum (strict)"(reference=w2029, "Val(Sgnl)"=w2023) -> ()  [unwired: 1 in, 2 out]
                n765 = property class="DigNum (strict)"(reference=w2031, "Val(Sgnl)"=w2026) -> ()  [unwired: 1 in, 2 out]
              }
              frame "GenericTOF" {
                n766 = First Call?() -> (First Call?: T/F=w2034:bool)
                n767 = case shown="True" w2034 {
                  frame False {
                  }
                  frame True {
                    w2035 = 0.0 ("Value (Signaling)")
                    n768 = control-ref of="Ch_B"() -> (w2036:refnum<vi>)
                    n769 = control-ref of="Ch_D"() -> (w2037:refnum<vi>)
                    n770 = control-ref of="Ch_A"() -> (w2039:refnum<vi>)
                    n771 = control-ref of="Ch_C"() -> (w2038:refnum<vi>)
                    n772 = property class="DigNum (strict)"(reference=w2036, "Val(Sgnl)"=w2035) -> ()  [unwired: 1 in, 2 out]
                    n773 = property class="DigNum (strict)"(reference=w2037, "Val(Sgnl)"=w2035) -> ()  [unwired: 1 in, 2 out]
                    n774 = property class="DigNum (strict)"(reference=w2039, "Val(Sgnl)"=w2035) -> ()  [unwired: 1 in, 2 out]
                    n775 = property class="DigNum (strict)"(reference=w2038, "Val(Sgnl)"=w2035) -> ()  [unwired: 1 in, 2 out]
                  }
                }
              }
              frame "BeamProfiling" {
                n776 = First Call?() -> (First Call?: T/F=w2040:bool)
                n777 = case shown="True" w2040 {
                  frame False {
                  }
                  frame True {
                    w2041 = 0.0 ("Value (Signaling)")
                    n778 = control-ref of="Ch_B"() -> (w2042:refnum<vi>)
                    n779 = control-ref of="Ch_D"() -> (w2043:refnum<vi>)
                    n780 = control-ref of="Ch_A"() -> (w2045:refnum<vi>)
                    n781 = control-ref of="Ch_C"() -> (w2044:refnum<vi>)
                    n782 = property class="DigNum (strict)"(reference=w2042, "Val(Sgnl)"=w2041) -> ()  [unwired: 1 in, 2 out]
                    n783 = property class="DigNum (strict)"(reference=w2043, "Val(Sgnl)"=w2041) -> ()  [unwired: 1 in, 2 out]
                    n784 = property class="DigNum (strict)"(reference=w2045, "Val(Sgnl)"=w2041) -> ()  [unwired: 1 in, 2 out]
                    n785 = property class="DigNum (strict)"(reference=w2044, "Val(Sgnl)"=w2041) -> ()  [unwired: 1 in, 2 out]
                  }
                }
              }
              frame Default {
                n786 = First Call?() -> (First Call?: T/F=w2046:bool)
                n787 = case shown="True" w2046 {
                  frame False {
                  }
                  frame True {
                    w2047 = 0.0 ("Value (Signaling)")
                    n788 = control-ref of="Ch_B"() -> (w2048:refnum<vi>)
                    n789 = control-ref of="Ch_D"() -> (w2049:refnum<vi>)
                    n790 = control-ref of="Ch_A"() -> (w2051:refnum<vi>)
                    n791 = control-ref of="Ch_C"() -> (w2050:refnum<vi>)
                    n792 = property class="DigNum (strict)"(reference=w2048, "Val(Sgnl)"=w2047) -> ()  [unwired: 1 in, 2 out]
                    n793 = property class="DigNum (strict)"(reference=w2049, "Val(Sgnl)"=w2047) -> ()  [unwired: 1 in, 2 out]
                    n794 = property class="DigNum (strict)"(reference=w2051, "Val(Sgnl)"=w2047) -> ()  [unwired: 1 in, 2 out]
                    n795 = property class="DigNum (strict)"(reference=w2050, "Val(Sgnl)"=w2047) -> ()  [unwired: 1 in, 2 out]
                  }
                }
              }
            }
          }
          event "Internal/Burst Rate": Value Change {
            n796 = event-data() -> ()  [unwired: 1 in, 2 out]
            n797 = Unbundle By Name(w2062) -> ("SRS DG535"=w2061:refnum<queue>)
            n798 = property on="DG535_Configs" class="Clust (strict)"() -> ("Value"=w2057:T48)  [unwired: 2 in, 2 out]
            n799 = Unbundle By Name(w2057) -> ("Trigger"=w2056:T27)
            n800 = Bundle By Name(cluster=w2056, "Internal/Burst Rate"="Internal/Burst Rate", "Trigger Mode"="Trigger Mode (SRS)") -> (w2053:T27)
            n801 = Bundle By Name(cluster=T82 {"State"=enum."Set Trigger", "Para."=variant} ("element"), "Para."=w2053) -> (w2059:T82)
            n802 = Bundle By Name(cluster=w2055, "Timing(LDPI).RepRate(Hz)"="Internal/Burst Rate", "DG535.Trigger"=w2053) -> (w2054:T50)
            n803 = Enqueue Element(queue=w2061, element=w2059) -> ()  [unwired: 2 in, 3 out]
          }
          event "SRS On/Off": Value Change {
            n804 = event-data() -> ()  [unwired: 1 in, 2 out]
            n805 = Unbundle By Name(w2073) -> ("SRS DG535"=w2072:refnum<queue>)
            n806 = Select(t=T82 {"State"=enum."Run", "Para."=variant} ("element"), s="SRS On/Off", f=T82 {"State"=enum."Stop", "Para."=variant}) -> (s? t:f=w2071:T82)
            n807 = Enqueue Element(queue=w2072, element=w2071) -> ()  [unwired: 2 in, 3 out]
            n808 = Unbundle By Name(w2066) -> ("DG535.Trigger.Trigger Mode"=w2064:T7, "InstrumentMode.LaserCtrlMethod"=w2068:T17)
            n809 = Equal?(x=DG535_TriggerMode."Internal" ("DG535.Trigger.Trigger Mode"), y=w2064) -> (x = y?=w2063:bool)
            n810 = case shown="True" w2063 {
              tunnel: w2068 -> [_ w2075]
              tunnel: "SRS On/Off" -> [_ w2074]
              frame False {
              }
              frame True {
                n811 = case shown="\"BNC\"" w2075 {
                  tunnel: w2074 -> [_ w2076]
                  frame Default {
                  }
                  frame "BNC" {
                    n812 = property on="LaserON" class="Bool (strict)"("Value"=w2076) -> ()  [unwired: 2 in, 2 out]
                  }
                }
              }
            }
          }
          event "Record": Value Change {
            n813 = event-data() -> ("NewVal"=w2081:bool)  [unwired: 1 in]
            n814 = Unbundle By Name(w2080) -> ("ProcCore_CtrlQueue"=w2079:refnum<queue>, "WriterCtrl"=w2078:refnum<queue>)
            n815 = case shown="True" w2081 {
              tunnel: w2078 -> [w2089 w2102]
              tunnel: w2079 -> [w2083 w2094]
              frame False {
                n816 = Bundle By Name(cluster=T75 {"Command"=enum."Initialize", "Params"=variant} ("element"), "Command"=ProcessStates."StopSave") -> (w2085:T75)
                n817 = Enqueue Element(queue=w2083, element=w2085) -> (error out=w2082:errorcluster)  [unwired: 2 in, 2 out]
                n818 = Enqueue Element(queue=w2089, element=T68 {"State"=enum."Close", "Params"=variant}, error in (no error)=w2082) -> ()  [unwired: 1 in, 3 out]
                n819 = property on="Snap" class="Bool (strict)"("DisabledEnum"=T49."Enabled" ("Disabled")) -> ()  [unwired: 2 in, 2 out]
              }
              frame True {
                n820 = local read "Files Format"() -> (w2092:T2)
                n821 = call <vilib>:"Dflt Data Dir.vi"() -> ("App:Default Data Directory"=w2090:path)
                n822 = Index Array(array=string[] ["*.txt", "*.mzml", "*.bin", "*.img", "*.imzML"], index=w2092) -> (element=w2091:string)
                n823 = feedback #6(w2090) -> (w2095:path)
                n824 = Strip Path(path=w2095) -> (stripped path=w2098:path, name=w2097:string)
                n825 = call "File Dialog2"("start path"=w2098, "default name"=w2097, "pattern (all files)"=w2091) -> ("selected path"=w2099:path, "cancelled"=w2101:bool, "error out"=w2100:errorcluster)  [unwired: 9 in, 1 out]
                n826 = case shown="False" w2101 {
                  tunnel: w2102 -> [w2111 _]
                  tunnel: w2099 -> [w2107 _]
                  tunnel: w2100 -> [_ _]
                  tunnel: [w2107 w2113] -> w2096
                  tunnel: w2095 -> [_ w2113]
                  tunnel: w2094 -> [w2106 _]
                  frame False {
                    n827 = local write "Filename Indicator"(w2107) -> ()
                    n828 = Bundle By Name(cluster=T75 {"Command"=enum."Initialize", "Params"=variant} ("element"), "Command"=ProcessStates."StartSave") -> (w2104:T75)
                    n829 = Bundle By Name(cluster=T68 {"State"=enum."Open", "Params"=variant} ("element"), "Params"=w2107) -> (w2109:T68)
                    n830 = property on="Snap" class="Bool (strict)"("DisabledEnum"=T49."Disabled and Grayed Out" ("Disabled")) -> ()  [unwired: 2 in, 2 out]
                    n831 = Enqueue Element(queue=w2106, element=w2104) -> ()  [unwired: 2 in, 3 out]
                    n832 = Enqueue Element(queue=w2111, element=w2109) -> ()  [unwired: 2 in, 3 out]
                  }
                  frame True {
                    n833 = property on="Record" class="Bool (strict)"("Value"=FALSE ("Save Multiple")) -> ()  [unwired: 2 in, 2 out]
                  }
                }
                n834 = feedback-in #6(w2096) -> ()
              }
            }
          }
          event "Snap": Value Change {
            n835 = event-data() -> ()  [unwired: 1 in, 1 out]
            n836 = local read "IncrementUpdate(A)"() -> (w2121:bool)
            n837 = local read "IncrementUpdate(B)"() -> (w2125:bool)
            n838 = local read "GraphEnable (A)"() -> (w2123:bool)
            n839 = local read "GraphEnable (B)"() -> (w2126:bool)
            n840 = Unbundle By Name(w2117) -> ("WriterCtrl"=w2116:refnum<queue>, "WriterSIG"=w2115:refnum<queue>)
            n841 = local read "Binning(A)"() -> (w2122:bool)
            n842 = local read "Binning(B)"() -> (w2124:bool)
            n843 = Compound Arithmetic op=AND(w2126, invert w2124, invert w2125) -> (w2118:bool)
            n844 = Compound Arithmetic op=AND(w2123, invert w2122, invert w2121) -> (w2119:bool)
            n845 = Or(x=w2118, y=w2119) -> (x .or. y?=w2120:bool)
            n846 = case shown="True" w2120 {
              tunnel: w2118 -> [_ w2146]
              tunnel: w2116 -> [_ w2144]
              tunnel: w2115 -> [_ w2143]
              tunnel: [_ w2139] -> w2127
              frame False {
                n847 = One Button Dialog(message="No active graph windows, no file is saved.\nPlease active one graph before press \"Save Once\"") -> ()  [unwired: 1 in, 1 out]
              }
              frame True {
                n848 = call <vilib>:"Dflt Data Dir.vi"() -> ("App:Default Data Directory"=w2130:path)
                n849 = local read "Graph (B)"() -> (w2140:cluster{dbl[], dbl[]})
                n850 = local read "Graph (A)"() -> (w2141:cluster{dbl[], dbl[]})
                n851 = Select(t=w2140, s=w2146, f=w2141) -> (s? t:f=w2142:cluster{dbl[], dbl[]})
                n852 = feedback #7(w2130) -> (w2132:path)
                n853 = Strip Path(path=w2132) -> (stripped path=w2136:path, name=w2135:string)
                n854 = call "File Dialog"("start path"=w2136, "default name"=w2135, "pattern (all files)"="*.txt", "pattern label"="Text MS File") -> ("selected path"=w2134:path, "cancelled"=w2145:bool, "error out"=w2131:errorcluster)  [unwired: 8 in, 1 out]
                n855 = case shown="False" w2145 {
                  tunnel: w2144 -> [_ _]
                  tunnel: w2134 -> [w2150 _]
                  tunnel: w2143 -> [_ _]
                  tunnel: w2142 -> [w2155 _]
                  tunnel: [w2151 _] -> w2139
                  tunnel: [w2150 w2156] -> w2133
                  tunnel: w2132 -> [_ w2156]
                  tunnel: w2131 -> [_ _]
                  frame False {
                    n856 = global read "Position_Micos.vi" "Position(Micos)"() -> (w2147:dbl[])
                    n857 = global read "Position_ESP300.vi" "Position_ESP"() -> (w2148:dbl[])
                    n858 = Unbundle(w2155) -> (w2154:dbl[])  [unwired: 1 out]
                    n859 = local read "Signal Segment"() -> (w2153:T3)
                    n860 = Insert Into Array(array=w2147, new element=w2148) -> (w2149:dbl[])  [unwired: 1 in]
                    n861 = Bundle By Name(cluster=w2153, "Spectrum"=w2154, "Position"=w2149) -> (w2152:T3)
                    n862 = call "WriteTextFile.vi"("Signal Segment"=w2152, "Filename"=w2150) -> ("error out"=w2151:errorcluster)  [unwired: 9 in]
                  }
                  frame True {
                  }
                }
                n863 = feedback-in #7(w2133) -> ()
              }
            }
            n864 = property on="Snap" class="Bool (strict)"(error in=w2127, "Value"=FALSE ("Save Once")) -> ()  [unwired: 1 in, 2 out]
          }
          event Value Change {
            n865 = event-data() -> ("NewVal"=w2161:T2)  [unwired: 1 in]
            n866 = Unbundle By Name(w2160) -> ("WriterCtrl"=w2159:refnum<queue>)
            n867 = Bundle By Name(cluster=T68 {"State"=enum."ChangeFormat", "Params"=variant} ("element"), "Params"=w2161) -> (w2163:T68)
            n868 = property on="Record" class="Bool (strict)"("Value"=FALSE ("Save Multiple")) -> (error out=w2158:errorcluster)  [unwired: 2 in, 1 out]
            n869 = Enqueue Element(queue=w2159, element=w2163, error in (no error)=w2158) -> ()  [unwired: 1 in, 3 out]
          }
          event Value Change {
            n870 = event-data() -> ()  [unwired: 1 in, 1 out]
            n871 = case shown="4294966296" "Gain (Voltage Range)" {
              selector: "Gain (Voltage Range)" -> [w2171 _ _ _]
              tunnel: [w2171 w2174 w2177 w2180] -> w2167
              tunnel: [0 ("Value (Signaling)") -180 ("Value (Signaling)") 180 ("Value (Signaling)") -400 ("Value (Signaling)")] -> w2168
              tunnel: [0.0 ("Value (Signaling)") 0.0175 ("Value (Signaling)") 0.0175 ("Value (Signaling)") 0.0055 ("Value (Signaling)")] -> w2169
              frame 100, 200, 400, 1000, 2000, 5000, 10000, Default {
              }
              frame -400 {
                w2174 = T10 400 items=["-100~900 mV"=4294966296, "-20~380 mV"=4294966896, "+/-5 V"=10000, "+/-2 V"=4000, "+/-1 V"=2000, "+/-500 mV"=1000, "+/-200 mV"=400, "+/-100 mV"=200, "+/-50 mV"=100] ("Gain (Voltage Range)")
                # "400mV range, 180 mV offset"
              }
              frame -401 {
                w2177 = T10 400 items=["-100~900 mV"=4294966296, "-20~380 mV"=4294966896, "+/-5 V"=10000, "+/-2 V"=4000, "+/-1 V"=2000, "+/-500 mV"=1000, "+/-200 mV"=400, "+/-100 mV"=200, "+/-50 mV"=100] ("Gain (Voltage Range)")
                # "400mV range, -180 mV offset"
              }
              frame -1000 {
                w2180 = T10 1000 items=["-100~900 mV"=4294966296, "-20~380 mV"=4294966896, "+/-5 V"=10000, "+/-2 V"=4000, "+/-1 V"=2000, "+/-500 mV"=1000, "+/-200 mV"=400, "+/-100 mV"=200, "+/-50 mV"=100] ("Gain (Voltage Range)")
                # "1000mV range, 400 mV offset"
              }
            }
            n872 = property on="Range" class="DigNum (strict)"("Value"=w2167) -> (error out=w2166:errorcluster)  [unwired: 2 in, 1 out]
            n873 = property on="ZeroOffsetCorrection" class="DigNum (strict)"("Val(Sgnl)"=w2169) -> ()  [unwired: 2 in, 2 out]
            n874 = property on="DC Offset" class="DigNum (strict)"(error in=w2166, "Val(Sgnl)"=w2168) -> ()  [unwired: 1 in, 2 out]
          }
          event Value Change {
            n875 = event-data() -> ()  [unwired: 1 in, 1 out]
            n876 = property on="Sample Rate" class="DigNum (strict)"("Val(Sgnl)"="SampleRate") -> ()  [unwired: 2 in, 2 out]
          }
          event Value Change {
            w2190 = T11 65280.0 items=["256K"=262144.0, "128K"=131072.0, "64K"=65280.0, "32K"=32768.0, "16K"=16384.0, "8K"=8192.0, "1K"=1024.0, "512"=512.0] ("y")
            n877 = event-data() -> ()  [unwired: 1 in, 1 out]
            n878 = control-ref of="Gage_Config"() -> (w2189:refnum<vi>)
            n879 = property class="Clust (strict)"(reference=w2189) -> (reference out=w2187:refnum<vi>, "Value"=w2188:T19)  [unwired: 1 in, 1 out]
            n880 = Greater? "For HwAverage"(x="Spectrum Length", y=w2190) -> ()  [unwired: 1 out]
            n881 = Bundle By Name(cluster=w2188, "Acquisition.Depth"="Spectrum Length", "Acquisition.Segment Size"="Spectrum Length") -> (w2186:T19)
            n882 = property class="Clust (strict)"(reference=w2187, "Val(Sgnl)"=w2186) -> ()  [unwired: 1 in, 2 out]
          }
          event "Scale(A)_X", "Scale(B)_X": Value Change {
            n883 = event-data() -> ()  [unwired: 1 in, 1 out]
            n884 = control-ref of="Graph (A)"() -> (w2195:refnum<vi>)
            n885 = control-ref of="Graph (B)"() -> (w2194:refnum<vi>)
            n886 = Build Array("Scale(A)_X", "Scale(B)_X") -> (w2196:bool[])
            n887 = Build Array(w2195, w2194) -> (w2193:refnum<vi>[])
            n888 = for {
              tunnel: w2196 -> [w2200] mode=indexing
              tunnel: w2193 -> [w2199] mode=indexing
              n889 = case shown="True" w2200 {
                tunnel: w2199 -> [_ w2203]
                frame False {
                }
                frame True {
                  n890 = property class="XYGraph (strict)"(reference=w2203) -> (reference out=w2201:refnum<vi>, "Value"=w2202:cluster{dbl[], dbl[]})  [unwired: 1 in, 1 out]
                  n891 = Unbundle(w2202) -> (w2211:dbl[])  [unwired: 1 out]
                  n892 = Array Size(array=w2211) -> (size(s)=w2209:i32)
                  n893 = Decrement(x=w2209) -> (x-1=w2210:i32)
                  n894 = Array Max & Min(array=w2211) -> (max value=w2206:dbl, min value=w2213:dbl)  [unwired: 2 out]
                  n895 = Index Array(array=w2211, index #1=0 ("index"), index #2=w2210) -> (element #2=w2207:dbl)  [unwired: 1 out]
                  n896 = In Range and Coerce(upper limit=w2206, x=0.0, lower limit=w2213) -> (coerced(x)=w2214:dbl)  [unwired: 1 out]
                  n897 = Round To Nearest(number=w2207) -> (nearest integer value=w2205:dbl)
                  n898 = Round Toward -Infinity(1:w2214) -> (0:w2204:dbl)
                  n899 = property on="Property Node" class="XYGraph (strict)"(reference=w2201, "XScale.Maximum"=w2205, "XScale.Minimum"=w2204) -> ()  [unwired: 1 in, 2 out]
                }
              }
            }
          }
          event "Scale(B)_Y", "Scale(A)_Y": Value Change {
            n900 = event-data() -> ()  [unwired: 1 in, 1 out]
            n901 = control-ref of="Graph (A)"() -> (w2221:refnum<vi>)
            n902 = control-ref of="Graph (B)"() -> (w2220:refnum<vi>)
            n903 = Build Array("Scale(A)_Y", "Scale(B)_Y") -> (w2217:bool[])
            n904 = Build Array(w2221, w2220) -> (w2216:refnum<vi>[])
            n905 = for {
              tunnel: w2217 -> [w2223] mode=indexing
              tunnel: w2216 -> [w2222] mode=indexing
              n906 = case shown="True" w2223 {
                tunnel: w2222 -> [_ w2224]
                frame False {
                }
                frame True {
                  n907 = call-poly "Autoscale_Y.vi"("GraphRef"=w2224) -> ()  [unwired: 11 in]
                }
              }
            }
          }
          event "Scale(A)X--", "Scale(A)X++", "Scale(B)X--", "Scale(B)X++": Value Change {
            w2226 = dbl[] [0.25, 1.0, 0.25, 1.0]  # ZoomIn/OutSetting
            n908 = event-data() -> ()  [unwired: 1 in, 1 out]
            n909 = control-ref of="Graph (A)"() -> (w2234:refnum<vi>)
            n910 = control-ref of="Graph (B)"() -> (w2233:refnum<vi>)
            n911 = Build Array("Scale(A)X++", "Scale(A)X--", "Scale(B)X++", "Scale(B)X--") -> (w2227:bool[])
            n912 = Build Array(w2234, w2234, w2233, w2233) -> (w2232:refnum<vi>[])
            n913 = for {
              tunnel: w2232 -> [w2237] mode=indexing
              tunnel: w2227 -> [w2236] mode=indexing
              tunnel: w2226 -> [w2235] mode=indexing
              n914 = case shown="True" w2236 {
                tunnel: w2237 -> [_ w2239]
                tunnel: w2235 -> [_ w2238]
                frame False {
                }
                frame True {
                  # "Zoom In"
                  n915 = property on="Property Node" class="XYGraph (strict)"(reference=w2239) -> (reference out=w2240:refnum<vi>, "XScale.Maximum"=w2249:dbl, "XScale.Minimum"=w2248:dbl)  [unwired: 1 in, 1 out]
                  n916 = Add(x=w2249, y=w2248) -> (x+y=w2247:dbl)
                  n917 = Subtract(x=w2249, y=w2248) -> (x-y=w2245:dbl)
                  n918 = Multiply(x=0.5, y=w2247) -> (x*y=w2244:dbl)
                  n919 = Multiply(x=w2245, y=w2238) -> (x*y=w2243:dbl)
                  n920 = Add(x=w2244, y=w2243) -> (x+y=w2242:dbl)
                  n921 = Subtract(x=w2244, y=w2243) -> (x-y=w2241:dbl)
                  n922 = property on="Property Node" class="XYGraph (strict)"(reference=w2240, "XScale.Maximum"=w2242, "XScale.Minimum"=w2241) -> ()  [unwired: 1 in, 2 out]
                }
              }
            }
          }
          event "Scale(A)Y++", "Scale(A)Y--", "Scale(B)Y++", "Scale(B)Y--": Value Change {
            n923 = event-data() -> ()  [unwired: 1 in, 1 out]
            n924 = control-ref of="Graph (A)"() -> (w2259:refnum<vi>)
            n925 = control-ref of="Graph (B)"() -> (w2258:refnum<vi>)
            n926 = Build Array(w2259, w2259, w2258, w2258) -> (w2251:refnum<vi>[])
            n927 = Build Array("Scale(A)Y++", "Scale(A)Y--", "Scale(B)Y++", "Scale(B)Y--") -> (w2253:bool[])
            n928 = for {
              tunnel: w2253 -> [w2262] mode=indexing
              tunnel: dbl[] [0.5, 2.0, 0.5, 2.0] -> [w2261] mode=indexing
              tunnel: w2251 -> [w2260] mode=indexing
              n929 = case shown="True" w2262 {
                tunnel: w2261 -> [_ w2264]
                tunnel: w2260 -> [_ w2263]
                frame False {
                }
                frame True {
                  n930 = call "Y_Scale_Change.vi"("Ratio"=w2264, "GraphRef"=w2263) -> ()  [unwired: 10 in]
                }
              }
            }
          }
          event User Event {
            n931 = event-data() -> ("Command"=w2266:T92, "Params."=w2286:variant)  [unwired: 1 in]
            n932 = Variant To Data(type=cluster{"Horizontal(%)":dbl, "Vertical(%)":dbl} {"Horizontal(%)"=0.0, "Vertical(%)"=0.0}, Variant=w2286) -> (data=w2284:cluster{"Horizontal(%)":dbl, "Vertical(%)":dbl})  [unwired: 1 in, 1 out]
            n933 = Unbundle By Name(w2284) -> ("Horizontal(%)"=w2275:dbl, "Vertical(%)"=w2274:dbl)
            n934 = control-ref of="Destination"() -> (w2281:refnum<vi>)
            n935 = call-poly <vilib>:"Array To Matrix.vi"("Real 2D Array"=dbl[][] [[5.0, 0.0, 1.0], [0.0, 5.0, 1.0], [0.0, 0.0, 1.0]]) -> ("Real Matrix"=w2271:T93)
            n936 = Build Array(w2275, w2274, 1.0 ("element")) -> (w2270:dbl[])
            n937 = property on="Property Node" class="Arr (strict)"(reference=w2281) -> (reference out=w2283:refnum<vi>, error out=w2282:errorcluster, "Value"=w2280:dbl[])  [unwired: 1 in]
            n938 = call-poly <vilib>:"A x B.vi"("Vector"=w2270, "A"=w2271) -> ("A x Vector"=w2269:dbl[])  [unwired: 1 out]
            n939 = Index Array(array=w2269) -> (element #1=w2268:dbl, element #2=w2267:dbl)  [unwired: 2 in]
            n940 = control-ref of="MoveAbs(Micos)"() -> (w2265:refnum<vi>)
            n941 = in-place {
              in-place-border: w2268 -> [w2297]
              in-place-border: w2267 -> [w2296]
              n942 = in-place-array #8(w2280, 0, 1) -> ()  [unwired: 2 out]
              n943 = in-place-array #8(w2297, w2296) -> (w2279:dbl[])  [unwired: 2 out]
            }
            n944 = case shown="\"MouseDoubleClick\"" w2266 {
              tunnel: w2283 -> [_ w2292 w2295]
              tunnel: w2282 -> [_ w2291 w2294]
              tunnel: w2279 -> [_ w2290 w2293]
              tunnel: w2265 -> [_ w2289 _]
              frame Default {
              }
              frame "MouseDoubleClick" {
                n945 = property on="Property Node" class="Arr (strict)"(reference=w2292, error in=w2291, "Value"=w2290) -> (error out=w2288:errorcluster)  [unwired: 1 out]
                n946 = property on="Property Node" class="Bool (strict)"(reference=w2289, error in=w2288, "Val(Sgnl)"=TRUE ("Value")) -> ()  [unwired: 2 out]
              }
              frame "MouseClick" {
                n947 = property on="Property Node" class="Arr (strict)"(reference=w2295, error in=w2294, "Value"=w2293) -> ()  [unwired: 2 out]
              }
            }
          }
          event "CameraOn": Value Change {
            n948 = event-data() -> ()  [unwired: 1 in, 1 out]
            n949 = disable-structure shown="IMAQdx_EXIST==TRUE" {
              disable-tunnel: w2299 -> [w2301 _]
              frame condition #0 {
                n950 = vi-ref "GenericCameraCore.vi"() -> (w2306:refnum<vi>)
                n951 = property class="VI Interface Type 1"(reference=w2306) -> (reference out=w2305:refnum<vi>, "Path"=w2304:path)  [unwired: 1 in, 1 out]
                n952 = Open VI Reference(type specifier VI Refnum (for type only)=w2305, vi path=w2304, options=128) -> (vi reference=w2303:refnum<vi>)  [unwired: 3 in, 1 out]
                n953 = call-by-ref "Start Asynchronous Call"(reference=w2303, "CameraEvent"=w2301, "Camera Selector"=T88 "cam0") -> ()  [unwired: 11 in, 2 out]
              }
              frame condition #1 (active) {
              }
            }
          }
        }
      }
      n954 = case "Main Data Acquisition Device Selector" shown="\"Gage_AdvMultiRec_8bit1Ch\"" w176 {
        tunnel: w270 -> [w411 w460 w474 _ w513 _ _]
        tunnel: w162 -> [w412 w461 w475 _ w512 _ _]
        tunnel: w262 -> [w413 w462 w476 w507 w514 _ _]
        tunnel: [w410 w459 w473 _ w511 _ _] -> w165
        frame "Gage" {
          # "Gage"
          n955 = disable-structure shown="GAGE_EXIST==TRUE" {
            disable-tunnel: w412 -> [w434 _]
            disable-tunnel: w411 -> [w433 _]
            disable-tunnel: [w426 _] -> w410
            frame condition #0 {
              n956 = property on="Gage_Config" class="Clust (strict)"() -> ("Value"=w418:T19)  [unwired: 2 in, 2 out]
              n957 = vi-ref "SecondaryData_Position.vi"() -> (w423:refnum<vi>)
              n958 = Bundle By Name(cluster=T72 {"SecondaryDataVIRef."=refnum, "Option"=0} ("SecondaryDataParams."), "SecondaryDataVIRef."=w423, "Option"=0) -> (w425:T72)
              n959 = Bundle By Name(cluster=T60 {"DWF States"=enum."SetAll_AcquChTrig_", "Variant"=variant} ("element"), "Variant"=w418) -> (w419:T60)
              n960 = Bundle By Name(cluster=T60 {"DWF States"=enum."SetSecondaryDataRef._", "Variant"=variant} ("element"), "Variant"=w425) -> (w420:T60)
              n961 = Build Array(T60 {"DWF States"=enum."Enumerate", "Variant"=variant} ("element"), T60 {"DWF States"=enum."Open", "Variant"=variant} ("element"), w420, w419) -> (w429:T60[])
              n962 = for {
                shift-right: [w438] -> w430
                shift-left: w433 -> [w439]
                tunnel: w429 -> [w437] mode=indexing
                shift-right: [w436] -> w416
                shift-left: _ -> [w435]
                n963 = Enqueue Element(queue=w439, element=w437, error in (no error)=w435) -> (queue out=w438:refnum<queue>, error out=w436:errorcluster)  [unwired: 1 in, 1 out]
              }
              n964 = control-ref of="Gage_Config"() -> (w428:refnum<vi>)
              n965 = property on="Get Some Values update" class="Clust (strict)"(reference=w428, error in=w416, "Val(Sgnl)"=w418) -> (error out=w427:errorcluster)  [unwired: 1 out]
              n966 = call <instrlib>:"Gage_Core.vi"("error in"=w427, "SignalBufferQueue"=w434, "DWFCtrlQueue in"=w430) -> ("error out"=w415:errorcluster)  [unwired: 8 in]
              n967 = Release Queue(queue=w430, error in (no error)=w415) -> (error out=w426:errorcluster)  [unwired: 1 in, 2 out]
            }
            frame condition #1 (active) {
            }
          }
          n968 = Unbundle By Name(w413) -> ("Graph"=w414:T67[])
          n969 = for {
            tunnel: w414 -> [w441] mode=indexing
            n970 = Unbundle By Name(w441) -> ("XY_Graph"=w440:refnum<vi>)
            n971 = property class="XYGraph (strict)"(reference=w440, "YScale.FormatString"="%#_3pV" ("Y Scale.Format String")) -> ()  [unwired: 1 in, 2 out]
          }
        }
        frame "KnifeEdge_Emu", "FakeSignal(Emulator)" {
          # "Beam profile:\nfocus at [0.5,0.5,0.5]\n\n3D Image Center:\n[0.5, 0.5, 1.5]\nZ range: 1.01 -1.99"
          # "Emulate Signal for testing. (Beam Profile and Image)"
          n972 = Unbundle By Name(w462) -> ("Graph"=w463:T67[])
          n973 = vi-ref "SecondaryData_Position.vi"() -> (w452:refnum<vi>)
          n974 = for {
            tunnel: w463 -> [w470] mode=indexing
            n975 = Unbundle By Name(w470) -> ("XY_Graph"=w469:refnum<vi>)
            n976 = property class="XYGraph (strict)"(reference=w469, "YScale.FormatString"="%#_3pV" ("Y Scale.Format String")) -> ()  [unwired: 1 in, 2 out]
          }
          n977 = Bundle By Name(cluster=T72 {"SecondaryDataVIRef."=refnum, "Option"=0} ("SecondaryDataParams."), "SecondaryDataVIRef."=w452, "Option"=0) -> (w454:T72)
          n978 = Bundle By Name(cluster=T60 {"DWF States"=enum."SetAll_AcquChTrig_", "Variant"=variant} ("element"), "Variant"="GenericDAQ_Config") -> (w444:T60)
          n979 = Bundle By Name(cluster=T60 {"DWF States"=enum."SetSecondaryDataRef._", "Variant"=variant} ("element"), "Variant"=w454) -> (w449:T60)
          n980 = Build Array(T60 {"DWF States"=enum."Enumerate", "Variant"=variant} ("element"), T60 {"DWF States"=enum."Open", "Variant"=variant} ("element"), w449, w444) -> (w455:T60[])
          n981 = for {
            shift-right: [w467] -> w456
            shift-left: w460 -> [w468]
            tunnel: w455 -> [w466] mode=indexing
            shift-right: [w465] -> w445
            shift-left: _ -> [w464]
            n982 = Enqueue Element(queue=w468, element=w466, error in (no error)=w464) -> (queue out=w467:refnum<queue>, error out=w465:errorcluster)  [unwired: 1 in, 1 out]
          }
          n983 = property on="GenericDAQ_Config" class="Clust (strict)"(error in=w445, "Val(Sgnl)"="GenericDAQ_Config") -> (error out=w446:errorcluster)  [unwired: 1 in, 1 out]
          n984 = call "GenericDAQCore.vi"("error in"=w446, "SignalBufferQueue"=w461, "DWFCtrlQueue in"=w456) -> ("error out"=w447:errorcluster)  [unwired: 8 in]
          n985 = Release Queue(queue=w456, error in (no error)=w447) -> (error out=w459:errorcluster)  [unwired: 1 in, 2 out]
        }
        frame "Gage_AdvMultiRec_8bit1Ch" {
          # "Gage"
          n986 = property on="Gage_Config" class="Clust (strict)"() -> ("Value"=w472:T19)  [unwired: 2 in, 2 out]
          n987 = Unbundle By Name(w476) -> ("Graph"=w477:T67[])
          n988 = disable-structure shown="GAGE_EXIST==TRUE" {
            disable-tunnel: w475 -> [w497 _]
            disable-tunnel: w474 -> [w496 _]
            disable-tunnel: [w489 _] -> w473
            disable-tunnel: w472 -> [w481 _]
            frame condition #0 {
              n989 = vi-ref "SecondaryData_Position.vi"() -> (w486:refnum<vi>)
              n990 = Bundle By Name(cluster=T72 {"SecondaryDataVIRef."=refnum, "Option"=0} ("SecondaryDataParams."), "SecondaryDataVIRef."=w486, "Option"=0) -> (w488:T72)
              n991 = Bundle By Name(cluster=T60 {"DWF States"=enum."SetAll_AcquChTrig_", "Variant"=variant} ("element"), "Variant"=w481) -> (w482:T60)
              n992 = Bundle By Name(cluster=T60 {"DWF States"=enum."SetSecondaryDataRef._", "Variant"=variant} ("element"), "Variant"=w488) -> (w483:T60)
              n993 = Build Array(T60 {"DWF States"=enum."Enumerate", "Variant"=variant} ("element"), T60 {"DWF States"=enum."Open", "Variant"=variant} ("element"), w483, w482) -> (w492:T60[])
              n994 = for {
                shift-right: [w501] -> w493
                shift-left: w496 -> [w502]
                tunnel: w492 -> [w500] mode=indexing
                shift-right: [w499] -> w479
                shift-left: _ -> [w498]
                n995 = Enqueue Element(queue=w502, element=w500, error in (no error)=w498) -> (queue out=w501:refnum<queue>, error out=w499:errorcluster)  [unwired: 1 in, 1 out]
              }
              n996 = control-ref of="Gage_Config"() -> (w491:refnum<vi>)
              n997 = property on="Get Some Values update" class="Clust (strict)"(reference=w491, error in=w479, "Val(Sgnl)"=w481) -> (error out=w490:errorcluster)  [unwired: 1 out]
              n998 = call <instrlib>:"GageAdvMultiRec8bit_Core.vi"("error in"=w490, "SignalBufferQueue in"=w497, "DWFCtrlQueue in"=w493) -> ("error out"=w478:errorcluster)  [unwired: 8 in]
              n999 = Release Queue(queue=w493, error in (no error)=w478) -> (error out=w489:errorcluster)  [unwired: 1 in, 2 out]
            }
            frame condition #1 (active) {
            }
          }
          n1000 = for {
            tunnel: w477 -> [w504] mode=indexing
            n1001 = Unbundle By Name(w504) -> ("XY_Graph"=w503:refnum<vi>)
            n1002 = property class="XYGraph (strict)"(reference=w503, "YScale.FormatString"="%#_3pV" ("Y Scale.Format String")) -> ()  [unwired: 1 in, 2 out]
          }
        }
        frame "IonWerks_TDCx4" {
          # "Obseleted Product\nRemoved from support list."
          # "Ionwerks TDCx4"
          n1003 = Unbundle By Name(w507) -> ("Graph"=w506:T67[])
          n1004 = for {
            tunnel: w506 -> [w509] mode=indexing
            n1005 = Unbundle By Name(w509) -> ("XY_Graph"=w508:refnum<vi>)
            n1006 = property class="XYGraph (strict)"(reference=w508, "YScale.FormatString"="%#_3pcps" ("Y Scale.Format String")) -> ()  [unwired: 1 in, 2 out]
          }
        }
        frame "AnalogDisc" {
          # "Gage"
          n1007 = disable-structure shown="AD_EXIST==TRUE" {
            disable-tunnel: w513 -> [w539 _]
            disable-tunnel: w512 -> [w531 _]
            disable-tunnel: [w521 _] -> w511
            frame condition #0 {
              n1008 = property on="AnalogDisc_Configs" class="Clust (strict)"() -> ("Value"=w518:T20)  [unwired: 2 in, 2 out]
              n1009 = vi-ref "SecondaryData_Position.vi"() -> (w525:refnum<vi>)
              n1010 = Bundle By Name(cluster=T73 {"SecondaryDataVIRef."=refnum, "Option"=0} ("SecondaryDataParams."), "SecondaryDataVIRef."=w525, "Option"=0) -> (w523:T73)
              n1011 = Bundle By Name(cluster=T60 {"DWF States"=enum."SetMode_", "Variant"=variant} ("element"), "Variant"=enum16{"Normal", "Turbo"}."Turbo" ("Mode")) -> (w534:T60)
              n1012 = Bundle By Name(cluster=T60 {"DWF States"=enum."SetAll_AcquChTrig_", "Variant"=variant} ("element"), "Variant"=w518) -> (w536:T60)
              n1013 = Bundle By Name(cluster=T60 {"DWF States"=enum."SetSecondaryDataRef._", "Variant"=variant} ("element"), "Variant"=w523) -> (w519:T60)
              n1014 = Build Array(T60 {"DWF States"=enum."CloseAll", "Variant"=variant} ("element"), T60 {"DWF States"=enum."Open", "Variant"=variant} ("element"), w536, T60 {"DWF States"=enum."fConfigurate", "Variant"=variant} ("element"), w534, T60 {"DWF States"=enum."fStart", "Variant"=variant} ("element"), w519) -> (w532:T60[])
              n1015 = for {
                shift-right: [w545] -> w522
                shift-left: w539 -> [w546]
                tunnel: w532 -> [w544] mode=indexing
                shift-right: [w543] -> w520
                shift-left: errorcluster {"status"=FALSE, "code"=0, "source"=""} ("error out") -> [w542]
                n1016 = Enqueue Element(queue=w546, element=w544, error in (no error)=w542) -> (queue out=w545:refnum<queue>, error out=w543:errorcluster)  [unwired: 1 in, 1 out]
              }
              n1017 = control-ref of="AnalogDisc_Configs"() -> (w529:refnum<vi>)
              n1018 = property class="Clust (strict)"(reference=w529, error in=w520, "Val(Sgnl)"=w518) -> (error out=w530:errorcluster)  [unwired: 1 out]
              n1019 = call <instrlib>:"AnalogDisc_Core.vi"("error in"=w530, "SignalBufferQueue"=w531, "DWFCtrlQueue in"=w522) -> ("error out"=w516:errorcluster)  [unwired: 8 in]
              n1020 = Release Queue(queue=w522, error in (no error)=w516) -> (error out=w521:errorcluster)  [unwired: 1 in, 2 out]
            }
            frame condition #1 (active) {
            }
          }
          n1021 = Unbundle By Name(w514) -> ("Graph"=w515:T67[])
          n1022 = for {
            tunnel: w515 -> [w548] mode=indexing
            n1023 = Unbundle By Name(w548) -> ("XY_Graph"=w547:refnum<vi>)
            n1024 = property class="XYGraph (strict)"(reference=w547, "YScale.FormatString"="%#_3pV" ("Y Scale.Format String")) -> ()  [unwired: 1 in, 2 out]
          }
        }
        frame Default {
        }
        frame "None" {
        }
      }
      n1025 = while "subApps Loop" {
        shift-right: [w561] -> w230
        shift-left: w351 -> [w568]
        tunnel: w269 -> [w577]
        tunnel: w263 -> [w557]
        tunnel: w158 -> [w558]
        stop <- w576 stop-if-true
        n1026 = Unbundle By Name(w557) -> ("InfoRef"=w566:refnum<vi>, "AppsLock"=w564:T63)
        n1027 = Unbundle By Name(w557) -> ("LaserCtrlMethod"=w559:T17)
        n1028 = property class="Str"(reference=w566, error in=w568, "Value"="subProgram Ready...") -> (error out=w569:errorcluster)  [unwired: 1 out]
        n1029 = Dequeue Element(queue=w577, error in (no error)=w569) -> (queue out=w571:refnum<queue>, element=w573:T71, timed out?=w574:bool, error out=w556:errorcluster)  [unwired: 1 in]
        n1030 = case shown="\"SDG_II\"" w559 {
          tunnel: [w580 w583 w586] -> w560
          tunnel: w556 -> [w578 w581 w585]
          tunnel: [w579 w582 w584] -> w555
          frame "BNC" {
            n1031 = property on="Rep.Rate (BNC)" class="DigNum (strict)"(error in=w578) -> (error out=w579:errorcluster, "Value"=w580:dbl)  [unwired: 1 in, 1 out]
          }
          frame "SRS_DG535" {
            n1032 = property on="Internal/Burst Rate" class="DigNum (strict)"(error in=w581) -> (error out=w582:errorcluster, "Value"=w583:dbl)  [unwired: 1 in, 1 out]
          }
          frame "SDG_II" {
            n1033 = property on="Internal/Burst Rate" class="DigNum (strict)"(error in=w585) -> (error out=w584:errorcluster, "Value"=w586:dbl)  [unwired: 1 in, 1 out]
          }
        }
        n1034 = Select(t=States-AToF."Idle", s=w574, f=w573) -> (s? t:f=w575:T71)
        n1035 = call <vilib>:"Acquire Semaphore.vi"("error in (no error)"=w555, "semaphore"=w564) -> ("error out"=w565:errorcluster, "semaphore out"=w563:T63)  [unwired: 3 in, 1 out]
        n1036 = case shown="\"Set_2PulseDelay\"" w575 {
          selector: w575 -> [_ _ _ _ _ _ _ _ _ _ _ _ _ _ _ _ _ _ w1133]
          tunnel: [_ _ _ _ _ _ _ _ _ _ _ _ _ _ _ _ TRUE _ _] -> w576
          tunnel: w565 -> [_ _ w629 w665 w699 w743 w785 w822 w864 w898 w936 w984 w1023 w1038 _ _ w1123 _ _]
          tunnel: w571 -> [_ _ w625 w661 w694 w740 w782 w820 w860 w894 w933 w980 _ w1035 _ _ w1122 _ _]
          tunnel: [_ _ w628 w664 w698 w742 w784 w825 w863 w897 w935 w983 w1020 w1037 _ _ _ _ _] -> w570
          tunnel: w557 -> [w603 w620 w626 w662 w696 w731 w777 w818 w861 w895 w934 w981 w1028 w1033 _ w1078 w1112 _ _]
          tunnel: w566 -> [_ _ _ _ _ _ _ _ _ _ _ _ _ _ _ _ _ _ w1126]
          tunnel: w560 -> [_ _ w623 w659 w693 w730 w776 w810 w857 w891 w926 w977 _ w1029 _ _ _ _ _]
          tunnel: w558 -> [_ _ w622 w658 _ _ _ w809 _ _ _ _ _ _ w1067 _ _ _ _]
          frame "Initialize" {
            n1037 = Unbundle By Name(w603) -> ("Micos"=w593:refnum<queue>, "WriterCtrl"=w602:refnum<queue>)
            n1038 = disable-structure shown="Disabled" {
              frame Disabled {
                n1039 = control-ref of="Gain (Voltage Range)"() -> ()  [unwired: 1 out]
                n1040 = control-ref of="Spectrum Length"() -> ()  [unwired: 1 out]
                n1041 = control-ref of="SampleRate"() -> ()  [unwired: 1 out]
                n1042 = control-ref of="Processing Mode\nNot Needed"() -> ()  [unwired: 1 out]
              }
              frame Enabled {
              }
            }
            n1043 = local read "Files Format"() -> (w604:T2)
            n1044 = Bundle By Name(cluster=T68 {"State"=enum."ChangeFormat", "Params"=variant} ("element"), "Params"=w604) -> (w605:T68)
            n1045 = Enqueue Element(queue=w602, element=w605) -> ()  [unwired: 2 in, 3 out]
            n1046 = Bundle By Name(cluster=T74 {"State"=enum."MotorEnable(1)", "Params."=variant} ("element"), "Params."=TRUE) -> (w595:T74)
            n1047 = Enqueue Element(queue=w593, element=w595) -> ()  [unwired: 2 in, 3 out]
            n1048 = control-ref of="Set Mode"() -> ()  [unwired: 1 out]
            n1049 = control-ref of="Velocity(Micos)"() -> (w601:refnum<vi>)
            n1050 = control-ref of="Accele.(Micos)"() -> (w599:refnum<vi>)
            n1051 = control-ref of="Velocity (ESP)"() -> (w598:refnum<vi>)
            n1052 = control-ref of="Accele. (ESP)"() -> (w592:refnum<vi>)
            n1053 = control-ref of="ZeroOffsetCorrection"() -> (w597:refnum<vi>)
            n1054 = control-ref of="Delay(LDI-Rej.)"() -> (w591:refnum<vi>)
            n1055 = control-ref of="Delay(PI)"() -> (w589:refnum<vi>)
            n1056 = control-ref of="Internal/Burst Rate"() -> (w590:refnum<vi>)
            n1057 = control-ref of="Trigger Mode (SRS)"() -> (w587:refnum<vi>)
            n1058 = Build Array(w601, w599, w598, w592, w597, w590, w591, w589) -> (w600:refnum<vi>[])
            n1059 = disable-structure "Diagram Disable Structure" shown="Enabled" {
              frame Enabled {
                # "Initial Values for SaveOnce function"
                n1060 = control-ref of="Cali."() -> (w612:refnum<vi>)
                n1061 = property on="This has to be enabled. No idea why." class="Arr (strict)"(reference=w612) -> (reference out=w611:refnum<vi>, error out=w613:errorcluster, "Value"=w614:dbl[])  [unwired: 1 in]
                n1062 = property on="Property Node" class="Arr (strict)"(reference=w611, error in=w613, "Val(Sgnl)"=w614) -> ()  [unwired: 2 out]
              }
              frame Disabled {
              }
            }
            n1063 = Build Array(w587) -> (w588:refnum<vi>[])
            n1064 = for {
              tunnel: w600 -> [w616] mode=indexing
              n1065 = property on="Property Node" class="DigNum (strict)"(reference=w616) -> (reference out=w615:refnum<vi>, error out=w618:errorcluster, "Value"=w617:dbl)  [unwired: 1 in]
              n1066 = property on="Property Node" class="DigNum (strict)"(reference=w615, error in=w618, "Val(Sgnl)"=w617) -> ()  [unwired: 2 out]
            }
            n1067 = for {
              tunnel: w588 -> [w608] mode=indexing
              n1068 = property on="Property Node" class="Enum (strict)"(reference=w608) -> (reference out=w607:refnum<vi>, error out=w610:errorcluster, "Value"=w609:T7)  [unwired: 1 in]
              n1069 = property on="Property Node" class="Enum (strict)"(reference=w607, error in=w610, "Val(Sgnl)"=w609) -> ()  [unwired: 2 out]
            }
          }
          frame "CalcMzArray" {
            # "data processing need separate contrl + data queue"
            n1070 = Unbundle By Name(w620) -> ("ProcCore_CtrlQueue"=w619:refnum<queue>)
            n1071 = Enqueue Element(queue=w619, element=T75 {"Command"=enum."CalcMzArray", "Params"=variant}) -> ()  [unwired: 2 in, 3 out]
          }
          frame "Meander_MCS" {
            n1072 = global read "Position_Micos.vi" "Position(Micos)"() -> (w624:dbl[])
            n1073 = call "CreateMeanderMask_3d.vi"("Rep. Rate (Hz)"=w623, "Start Position"=w624) -> ("Laser_Ctrl"=w630:bool, "start/end points"=w631:cluster{dbl, dbl, dbl}[][], "Canceled"=w632:bool, "ImageParameter"=w627:T94)  [unwired: 6 in]
            n1074 = case shown="False" w632 {
              tunnel: w631 -> [w656 _]
              tunnel: w629 -> [w643 w657]
              tunnel: w630 -> [w655 _]
              tunnel: [w646 w657] -> w628
              tunnel: w627 -> [w639 _]
              tunnel: w626 -> [w641 _]
              tunnel: w625 -> [w640 _]
              tunnel: w622 -> [w635 _]
              frame False {
                n1075 = Unbundle By Name(w635) -> ()  [unwired: 1 out]
                n1076 = Unbundle By Name(w639) -> ("Start Position"=w649:dbl[], "StepWidth"=w648:dbl[], "Dimension"=w647:i32[], "ScanSpeed"=w637:dbl)
                n1077 = property on="Depth" class="DigNum (strict)"() -> ("Value"=w638:dbl)  [unwired: 2 in, 2 out]
                n1078 = control-ref of="Velocity(Micos)"() -> (w634:refnum<vi>)
                n1079 = Bundle By Name(cluster=T77 {"Start Position"=[], "StepWidth"=[], "Dimension"=[], "SpecLength"=0} ("File Header"), "SpecLength"=w638, "Start Position"=w649, "StepWidth"=w648, "Dimension"=w647) -> (w650:T77)
                n1080 = Unbundle By Name(w641) -> ("Micos"=w636:refnum<queue>, "WriterCtrl"=w642:refnum<queue>)
                n1081 = Bundle By Name(cluster=T68 {"State"=enum."SetHeader", "Params"=variant} ("element"), "Params"=w650) -> (w652:T68)
                n1082 = property class="DigNum (strict)"(reference=w634) -> ("Value"=w633:dbl)  [unwired: 1 in, 2 out]
                n1083 = Enqueue Element(queue=w642, element=w652, error in (no error)=w643) -> (error out=w644:errorcluster)  [unwired: 1 in, 2 out]
                n1084 = call "MeanderCtrl_3d_StageRefs.vi"("QueuesRef"=w641, "MotionStageRefs"=w636, "AppsRef"=w640, "start/end points"=w656, "Laser_Ctrl"=w655, "error in"=w644, "HighSpeed"=w633, "ScanSpeed"=w637) -> ("error out"=w645:errorcluster)  [unwired: 5 in, 2 out]
                n1085 = property on="Record" class="Bool (strict)"(error in=w645, "Val(Sgnl)"=FALSE) -> (error out=w646:errorcluster)  [unwired: 1 in, 1 out]
              }
              frame True {
              }
            }
          }
          frame "CleanSurface" {
            n1086 = global read "Position_Micos.vi" "Position(Micos)"() -> (w660:dbl[])
            n1087 = call "CleanSurface_3d.vi"("Rep. Rate (Hz)"=w659, "Start Position"=w660) -> ("BNC_Ctrl"=w666:bool, "start/end points"=w667:cluster{dbl, dbl, dbl}[][], "Canceled"=w668:bool, "ImageParameter"=w663:T95)  [unwired: 6 in]
            n1088 = case shown="False" w668 {
              tunnel: w667 -> [w691 _]
              tunnel: w665 -> [w678 w692]
              tunnel: w666 -> [w690 _]
              tunnel: [w681 w692] -> w664
              tunnel: w663 -> [w671 _]
              tunnel: w662 -> [w675 _]
              tunnel: w661 -> [w674 _]
              tunnel: w658 -> [_ _]
              frame False {
                n1089 = Unbundle By Name(w675) -> ("WriterCtrl"=w676:refnum<queue>)
                n1090 = Unbundle By Name(w671) -> ("MeanderSpeed"=w669:dbl, "Start Position"=w684:dbl[], "StepWidth"=w683:dbl[], "Dimension"=w682:i32[])
                n1091 = property on="Depth" class="DigNum (strict)"() -> ("Value"=w670:dbl)  [unwired: 2 in, 2 out]
                n1092 = Bundle By Name(cluster=T77 {"Start Position"=[], "StepWidth"=[], "Dimension"=[], "SpecLength"=0} ("File Header"), "Start Position"=w684, "StepWidth"=w683, "Dimension"=w682, "SpecLength"=w670) -> (w685:T77)
                n1093 = control-ref of="Velocity(Micos)"() -> (w673:refnum<vi>)
                n1094 = Bundle By Name(cluster=T68 {"State"=enum."SetHeader", "Params"=variant} ("element"), "Params"=w685) -> (w687:T68)
                n1095 = property class="DigNum (strict)"(reference=w673) -> ("Value"=w672:dbl)  [unwired: 1 in, 2 out]
                n1096 = Enqueue Element(queue=w676, element=w687, error in (no error)=w678) -> (error out=w679:errorcluster)  [unwired: 1 in, 2 out]
                n1097 = Unbundle By Name(w675) -> ("Micos"=w677:refnum<queue>)
                n1098 = call "MeanderCtrl_3d_StageRefs.vi"("QueuesRef"=w675, "MotionStageRefs"=w677, "AppsRef"=w674, "start/end points"=w691, "Laser_Ctrl"=w690, "error in"=w679, "HighSpeed"=w672, "ScanSpeed"=w669) -> ("error out"=w680:errorcluster)  [unwired: 5 in, 2 out]
                n1099 = property on="Record" class="Bool (strict)"(error in=w680, "Val(Sgnl)"=FALSE) -> (error out=w681:errorcluster)  [unwired: 1 in, 1 out]
              }
              frame True {
              }
            }
          }
          frame "Meander_Npt" {
            n1100 = global read "Position_ESP300.vi" "Position_ESP"() -> (w695:dbl[])
            n1101 = call "CreateMeanderMask_3d.vi"("Rep. Rate (Hz)"=w693, "Start Position"=w695) -> ("Laser_Ctrl"=w700:bool, "start/end points"=w702:cluster{dbl, dbl, dbl}[][], "Canceled"=w703:bool, "ImageParameter"=w697:T94)  [unwired: 6 in]
            n1102 = Unbundle By Name(w697) -> ("ScanSpeed"=w701:dbl)
            n1103 = case shown="False" w703 {
              tunnel: w702 -> [w726 _]
              tunnel: w699 -> [w711 w727]
              tunnel: w701 -> [w725 _]
              tunnel: w700 -> [w724 _]
              tunnel: [w714 w727] -> w698
              tunnel: w697 -> [w718 _]
              tunnel: w696 -> [w706 _]
              tunnel: w694 -> [w705 _]
              frame False {
                n1104 = Unbundle By Name(w718) -> ("Start Position"=w717:dbl[], "StepWidth"=w716:dbl[], "Dimension"=w715:i32[])
                n1105 = Unbundle By Name(w706) -> ("WriterCtrl"=w707:refnum<queue>)
                n1106 = property on="Depth" class="DigNum (strict)"() -> ("Value"=w704:dbl)  [unwired: 2 in, 2 out]
                n1107 = Bundle By Name(cluster=T77 {"Start Position"=[], "StepWidth"=[], "Dimension"=[], "SpecLength"=0} ("File Header"), "Start Position"=w717, "StepWidth"=w716, "Dimension"=w715, "SpecLength"=w704) -> (w719:T77)
                n1108 = control-ref of="Velocity (ESP)"() -> (w710:refnum<vi>)
                n1109 = Bundle By Name(cluster=T68 {"State"=enum."SetHeader", "Params"=variant} ("element"), "Params"=w719) -> (w721:T68)
                n1110 = property class="DigNum (strict)"(reference=w710) -> ("Value"=w709:dbl)  [unwired: 1 in, 2 out]
                n1111 = Enqueue Element(queue=w707, element=w721, error in (no error)=w711) -> (error out=w712:errorcluster)  [unwired: 1 in, 2 out]
                n1112 = Unbundle By Name(w706) -> ("ESP300"=w708:refnum<queue>)
                n1113 = call "MeanderCtrl_3d_StageRefs.vi"("QueuesRef"=w706, "MotionStageRefs"=w708, "AppsRef"=w705, "start/end points"=w726, "Laser_Ctrl"=w724, "error in"=w712, "HighSpeed"=w709, "ScanSpeed"=w725) -> ("error out"=w713:errorcluster)  [unwired: 5 in, 2 out]
                n1114 = property on="Record" class="Bool (strict)"(error in=w713, "Val(Sgnl)"=FALSE) -> (error out=w714:errorcluster)  [unwired: 1 in, 1 out]
              }
              frame True {
              }
            }
          }
          frame "KnifeEdgeExpt" {
            n1115 = global read "Position_Micos.vi" "Position(Micos)"() -> (w739:dbl[])
            n1116 = vi-ref "SecondaryData_Position.vi"() -> (w733:refnum<vi>)
            n1117 = Bundle By Name(cluster=T72 {"SecondaryDataVIRef."=refnum, "Option"=0} ("SecondaryDataParams."), "SecondaryDataVIRef."=w733, "Option"=0) -> (w732:T72)
            n1118 = call "KnifeEdgeExpt.vi"("Rep. Rate (Hz)"=w730, "Start Position"=w739) -> ("SDG_Ctrl"=w744:bool, "Canceled"=w746:bool, "Angle_Incident"=w738:dbl, "X/Y (T:Y)"=w737:bool, "ImageParameter"=w741:T95, "w_fit_init."=w729:dbl[], "z0_fit_init."=w728:dbl[])  [unwired: 2 in, 1 out]
            n1119 = Unbundle By Name(w741) -> ("MeanderSpeed"=w745:dbl)
            n1120 = vi-ref "BeamProfile_Proc.vi"() -> (w736:refnum<vi>)
            n1121 = case shown="False" w746 {
              tunnel: w743 -> [w750 w775]
              tunnel: w745 -> [w761 _]
              tunnel: w744 -> [w774 _]
              tunnel: [w771 w775] -> w742
              tunnel: w741 -> [w772 _]
              tunnel: w731 -> [w752 _]
              tunnel: w740 -> [w768 _]
              tunnel: w738 -> [w759 _]
              tunnel: w737 -> [w758 _]
              tunnel: w736 -> [w757 _]
              tunnel: w732 -> [w753 _]
              tunnel: w729 -> [w748 _]
              tunnel: w728 -> [w747 _]
              frame False {
                n1122 = control-ref of="Velocity(Micos)"() -> (w767:refnum<vi>)
                n1123 = Unbundle By Name(w752) -> ("MainDAQCoreQueue"=w756:refnum<queue>)
                n1124 = property class="DigNum (strict)"(reference=w767) -> ("Value"=w760:dbl)  [unwired: 1 in, 2 out]
                n1125 = Bundle By Name(cluster=T60 {"DWF States"=enum."SetSecondaryDataRef._", "Variant"=variant} ("element"), "Variant"=w753) -> (w755:T60)
                n1126 = Enqueue Element(queue=w756, element=w755, error in (no error)=w750) -> (error out=w751:errorcluster)  [unwired: 1 in, 2 out]
                n1127 = Unbundle By Name(w772) -> ("Start Position"=w765:dbl[], "StepWidth"=w764:dbl[], "Dimension"=w763:i32[])
                n1128 = property on="Depth" class="DigNum (strict)"() -> ("Value"=w749:dbl)  [unwired: 2 in, 2 out]
                n1129 = Bundle By Name(cluster=T78 {"File Header"={"Start Position"=[], "StepWidth"=[], "Dimension"=[], "SpecLength"=0}, "w_fit_init."=[], "z0_fit_init."=[], "LowSpeed"=0.0, "HighSpeed"=0.0, "x/y?"=FALSE, "IncidentAngle"=0.0} ("BeamProfiling_Params"), "File Header.SpecLength"=w749, "w_fit_init."=w748, "z0_fit_init."=w747, "File Header.Start Position"=w765, "File Header.StepWidth"=w764, "File Header.Dimension"=w763, "LowSpeed"=w761, "HighSpeed"=w760, "IncidentAngle"=w759, "x/y?"=w758) -> (w762:T78)
                n1130 = Unbundle By Name(w752) -> ("Micos"=w769:refnum<queue>)
                n1131 = call "MeanderCtrl_Dynamic,StageRefs.vi"("QueuesRef"=w752, "MotionStageRefs"=w769, "AppsRef"=w768, "subprog_Ref"=w757, "Params."=w762, "Laser_Ctrl"=w774, "error in"=w751, "HighSpeed"=w760, "LowSpeed"=w761) -> ("error out"=w770:errorcluster)  [unwired: 5 in, 1 out]
                n1132 = property on="Record" class="Bool (strict)"(error in=w770, "Val(Sgnl)"=FALSE) -> (error out=w771:errorcluster)  [unwired: 1 in, 1 out]
              }
              frame True {
              }
            }
          }
          frame "InstruOptimizer_static" {
            n1133 = global read "Position_Micos.vi" "Position(Micos)"() -> (w781:dbl[])
            n1134 = call "KnifeEdgeExpt.vi"("Rep. Rate (Hz)"=w776, "Start Position"=w781) -> ("SDG_Ctrl"=w786:bool, "Canceled"=w788:bool, "Angle_Incident"=w780:dbl, "X/Y (T:Y)"=w779:bool, "ImageParameter"=w783:T95)  [unwired: 2 in, 3 out]
            n1135 = Unbundle By Name(w783) -> ("MeanderSpeed"=w787:dbl)
            n1136 = disable-structure shown="Disabled" {
              disable-tunnel: [w789 _] -> w778
              frame Disabled {
                n1137 = vi-ref "APSO_static.vi"() -> (w789:refnum<vi>)
              }
              frame Enabled {
              }
            }
            n1138 = case shown="False" w788 {
              tunnel: w785 -> [w794 w806]
              tunnel: w787 -> [w790 _]
              tunnel: w786 -> [w805 _]
              tunnel: [w802 w806] -> w784
              tunnel: w783 -> [w803 _]
              tunnel: w777 -> [w795 _]
              tunnel: w782 -> [w799 _]
              tunnel: w780 -> [_ _]
              tunnel: w779 -> [_ _]
              tunnel: w778 -> [w796 _]
              frame False {
                n1139 = Unbundle By Name(w803) -> ("Start Position"=w798:dbl[])  [unwired: 2 out]
                n1140 = Bundle By Name(cluster=T79 {"File Header"={"Start Position"=[], "StepWidth"=[], "Dimension"=[], "SpecLength"=0}, "Instru.Params."=[], "APSO_Params."=[], "LowSpeed"=0.0, "HighSpeed"=0.0} ("BeamProfiling_Params"), "Instru.Params."=dbl[] [], "APSO_Params."=dbl[] [], "File Header.Start Position"=w798, "LowSpeed"=w790, "HighSpeed"=w790) -> (w797:T79)
                n1141 = Unbundle By Name(w795) -> ("Micos"=w800:refnum<queue>)
                n1142 = call "MeanderCtrl_Dynamic,StageRefs.vi"("QueuesRef"=w795, "MotionStageRefs"=w800, "AppsRef"=w799, "subprog_Ref"=w796, "Params."=w797, "Laser_Ctrl"=w805, "error in"=w794, "LowSpeed"=w790) -> ("error out"=w801:errorcluster)  [unwired: 6 in, 1 out]
                n1143 = property on="Record" class="Bool (strict)"(error in=w801, "Val(Sgnl)"=FALSE) -> (error out=w802:errorcluster)  [unwired: 1 in, 1 out]
              }
              frame True {
              }
            }
          }
          frame "KnifeEdgeExpt_Npt" {
            w813 = 1  # Swap ESP/Micos
            n1144 = global read "Position_ESP300.vi" "Position_ESP"() -> (w826:dbl[])
            n1145 = vi-ref "SecondaryData_Position.vi"() -> (w812:refnum<vi>)
            n1146 = call "KnifeEdgeExpt.vi"("Rep. Rate (Hz)"=w810, "Start Position"=w826) -> ("SDG_Ctrl"=w823:bool, "Canceled"=w821:bool, "Angle_Incident"=w817:dbl, "X/Y (T:Y)"=w816:bool, "ImageParameter"=w819:T95, "w_fit_init."=w808:dbl[], "z0_fit_init."=w807:dbl[])  [unwired: 2 in, 1 out]
            n1147 = Bundle By Name(cluster=T73 {"SecondaryDataVIRef."=refnum, "Option"=0} ("SecondaryDataParams."), "SecondaryDataVIRef."=w812, "Option"=w813) -> (w811:T73)
            n1148 = Unbundle By Name(w819) -> ("MeanderSpeed"=w824:dbl)
            n1149 = vi-ref "BeamProfile_Proc.vi"() -> (w815:refnum<vi>)
            n1150 = case shown="False" w821 {
              tunnel: w822 -> [w834 w856]
              tunnel: w824 -> [w843 _]
              tunnel: w823 -> [w855 _]
              tunnel: [w852 w856] -> w825
              tunnel: w819 -> [w853 _]
              tunnel: w818 -> [w831 _]
              tunnel: w820 -> [w849 _]
              tunnel: w817 -> [w842 _]
              tunnel: w816 -> [w841 _]
              tunnel: w815 -> [w840 _]
              tunnel: w811 -> [w836 _]
              tunnel: w809 -> [w832 _]
              tunnel: w808 -> [w828 _]
              tunnel: w807 -> [w827 _]
              frame False {
                n1151 = Unbundle By Name(w832) -> ()  [unwired: 1 out]
                n1152 = Unbundle By Name(w831) -> ("MainDAQCoreQueue"=w839:refnum<queue>)
                n1153 = Bundle By Name(cluster=T60 {"DWF States"=enum."SetSecondaryDataRef._", "Variant"=variant} ("element"), "Variant"=w836) -> (w837:T60)
                n1154 = control-ref of="Velocity (ESP)"() -> (w830:refnum<vi>)
                n1155 = Enqueue Element(queue=w839, element=w837, error in (no error)=w834) -> (error out=w835:errorcluster)  [unwired: 1 in, 2 out]
                n1156 = property class="DigNum (strict)"(reference=w830) -> ("Value"=w829:dbl)  [unwired: 1 in, 2 out]
                n1157 = Unbundle By Name(w853) -> ("Start Position"=w847:dbl[], "StepWidth"=w846:dbl[], "Dimension"=w845:i32[])
                n1158 = property on="Depth" class="DigNum (strict)"() -> ("Value"=w833:dbl)  [unwired: 2 in, 2 out]
                n1159 = Bundle By Name(cluster=T78 {"File Header"={"Start Position"=[], "StepWidth"=[], "Dimension"=[], "SpecLength"=0}, "w_fit_init."=[], "z0_fit_init."=[], "LowSpeed"=0.0, "HighSpeed"=0.0, "x/y?"=FALSE, "IncidentAngle"=0.0} ("BeamProfiling_Params"), "File Header.Start Position"=w847, "File Header.StepWidth"=w846, "File Header.Dimension"=w845, "File Header.SpecLength"=w833, "LowSpeed"=w843, "HighSpeed"=w829, "x/y?"=w841, "IncidentAngle"=w842, "w_fit_init."=w828, "z0_fit_init."=w827) -> (w844:T78)
                n1160 = Unbundle By Name(w831) -> ("ESP300"=w850:refnum<queue>)
                n1161 = call "MeanderCtrl_Dynamic,StageRefs.vi"("QueuesRef"=w831, "MotionStageRefs"=w850, "AppsRef"=w849, "subprog_Ref"=w840, "Params."=w844, "Laser_Ctrl"=w855, "error in"=w835, "HighSpeed"=w829, "LowSpeed"=w843) -> ("error out"=w851:errorcluster)  [unwired: 5 in, 1 out]
                n1162 = property on="Record" class="Bool (strict)"(error in=w851, "Val(Sgnl)"=FALSE) -> (error out=w852:errorcluster)  [unwired: 1 in, 1 out]
              }
              frame True {
              }
            }
          }
          frame "Imaging_Micos" {
            n1163 = global read "Position_Micos.vi" "Position(Micos)"() -> (w859:dbl[])
            n1164 = vi-ref "Imaging_Proc.vi"() -> (w858:refnum<vi>)
            n1165 = call "CreateMeanderMask_3d.vi"("Rep. Rate (Hz)"=w857, "Start Position"=w859) -> ("Laser_Ctrl"=w865:bool, "Canceled"=w866:bool, "ImageParameter"=w862:T94)  [unwired: 6 in, 1 out]
            n1166 = case shown="True" w866 {
              tunnel: w864 -> [w874 w890]
              tunnel: w865 -> [w889 _]
              tunnel: [w887 w890] -> w863
              tunnel: w862 -> [w881 _]
              tunnel: w861 -> [w884 _]
              tunnel: w860 -> [w883 _]
              tunnel: w858 -> [w872 _]
              frame False {
                n1167 = Unbundle By Name(w881) -> ("Start Position"=w879:dbl[], "StepWidth"=w878:dbl[], "Dimension"=w877:i32[], "ScanSpeed"=w880:dbl)
                n1168 = property on="Sample Rate" class="DigNum (strict)"() -> ("Value"=w870:dbl)  [unwired: 2 in, 2 out]
                n1169 = property on="Trigger Delay" class="DigNum (strict)"() -> ("Value"=w869:dbl)  [unwired: 2 in, 2 out]
                n1170 = property on="Depth" class="DigNum (strict)"() -> ("Value"=w871:dbl)  [unwired: 2 in, 2 out]
                n1171 = local read "Velocity(Micos)"() -> (w873:dbl)
                n1172 = Subtract(x=w871, y=64.0) -> (x-y=w868:dbl)
                n1173 = property on="Cali." class="Arr (strict)"() -> ("Value"=w876:dbl[])  [unwired: 2 in, 2 out]
                n1174 = Bundle By Name(cluster=T80 {"File Header"={"Start Position"=[], "StepWidth"=[], "Dimension"=[], "SpecLength"=0}, "ScanSpeed"=0.0, "HighSpeed"=0.0, "SampleRate"=0.0, "Rep.Rate (Hz)"=0.0, "TrigDelay"=0.0, "mzCali"=[], "KeepStill(ms)"=0, "SaveRaw"=FALSE} ("BeamProfiling_Params"), "File Header.SpecLength"=w868, "SampleRate"=w870, "TrigDelay"=w869, "mzCali"=w876, "File Header.Start Position"=w879, "File Header.StepWidth"=w878, "File Header.Dimension"=w877, "ScanSpeed"=w880, "HighSpeed"=w873) -> (w875:T80)
                n1175 = Unbundle By Name(w884) -> ("Micos"=w885:refnum<queue>)
                n1176 = call "MeanderCtrl_Dynamic,StageRefs.vi"("QueuesRef"=w884, "MotionStageRefs"=w885, "AppsRef"=w883, "subprog_Ref"=w872, "Params."=w875, "Laser_Ctrl"=w889, "error in"=w874, "HighSpeed"=w873, "LowSpeed"=w880) -> ("error out"=w886:errorcluster)  [unwired: 5 in, 1 out]
                n1177 = property on="Record" class="Bool (strict)"(error in=w886, "Val(Sgnl)"=FALSE) -> (error out=w887:errorcluster)  [unwired: 1 in, 1 out]
              }
              frame True {
              }
            }
          }
          frame "DepthProfiling(3D)" {
            n1178 = global read "Position_Micos.vi" "Position(Micos)"() -> (w893:dbl[])
            n1179 = vi-ref "DepthProfiling_3D_Core.vi"() -> (w892:refnum<vi>)
            n1180 = call "CreateMeanderMask_3d.vi"("Rep. Rate (Hz)"=w891, "Start Position"=w893) -> ("Laser_Ctrl"=w899:bool, "start/end points"=w900:cluster{dbl, dbl, dbl}[][], "Canceled"=w901:bool, "ImageParameter"=w896:T94)  [unwired: 6 in]
            n1181 = case shown="False" w901 {
              tunnel: w900 -> [_ _]
              tunnel: w898 -> [w909 w925]
              tunnel: w899 -> [w924 _]
              tunnel: [w922 w925] -> w897
              tunnel: w896 -> [w916 _]
              tunnel: w895 -> [w919 _]
              tunnel: w894 -> [w918 _]
              tunnel: w892 -> [w907 _]
              frame False {
                n1182 = Unbundle By Name(w916) -> ("Start Position"=w914:dbl[], "StepWidth"=w913:dbl[], "Dimension"=w912:i32[], "ScanSpeed"=w915:dbl)
                n1183 = property on="Sample Rate" class="DigNum (strict)"() -> ("Value"=w905:dbl)  [unwired: 2 in, 2 out]
                n1184 = property on="Trigger Delay" class="DigNum (strict)"() -> ("Value"=w904:dbl)  [unwired: 2 in, 2 out]
                n1185 = property on="Depth" class="DigNum (strict)"() -> ("Value"=w906:dbl)  [unwired: 2 in, 2 out]
                n1186 = local read "Velocity(Micos)"() -> (w908:dbl)
                n1187 = Subtract(x=w906, y=64.0) -> (x-y=w903:dbl)
                n1188 = property on="Cali." class="Arr (strict)"() -> ("Value"=w911:dbl[])  [unwired: 2 in, 2 out]
                n1189 = Bundle By Name(cluster=T80 {"File Header"={"Start Position"=[], "StepWidth"=[], "Dimension"=[], "SpecLength"=0}, "ScanSpeed"=0.0, "HighSpeed"=0.0, "SampleRate"=0.0, "Rep.Rate (Hz)"=0.0, "TrigDelay"=0.0, "mzCali"=[], "KeepStill(ms)"=0, "SaveRaw"=FALSE} ("BeamProfiling_Params"), "File Header.SpecLength"=w903, "SampleRate"=w905, "TrigDelay"=w904, "mzCali"=w911, "File Header.Start Position"=w914, "File Header.StepWidth"=w913, "File Header.Dimension"=w912, "ScanSpeed"=w915, "HighSpeed"=w908) -> (w910:T80)
                n1190 = Unbundle By Name(w919) -> ("Micos"=w920:refnum<queue>)
                n1191 = call "MeanderCtrl_Dynamic,StageRefs.vi"("QueuesRef"=w919, "MotionStageRefs"=w920, "AppsRef"=w918, "subprog_Ref"=w907, "Params."=w910, "Laser_Ctrl"=w924, "error in"=w909, "HighSpeed"=w908, "LowSpeed"=w915) -> ("error out"=w921:errorcluster)  [unwired: 5 in, 1 out]
                n1192 = property on="Record" class="Bool (strict)"(error in=w921, "Val(Sgnl)"=FALSE) -> (error out=w922:errorcluster)  [unwired: 1 in, 1 out]
              }
              frame True {
              }
            }
          }
          frame "DepthProfile_RT" {
            n1193 = global read "Position_Micos.vi" "Position(Micos)"() -> (w929:dbl[])
            n1194 = vi-ref "DepthProfiling_Proc.vi"() -> (w932:refnum<vi>)
            n1195 = call "DepthProfile_Setup.vi"("RepRate (Hz)"=w926, "Start Position"=w929) -> ("Depth Profile Params."=w928:T96, "Canceled"=w930:bool, "Meander_Params."=w931:T77, "SaveRaw"=w927:bool)  [unwired: 6 in]
            n1196 = case shown="False" w930 {
              tunnel: w936 -> [w942 w976]
              tunnel: [w960 w976] -> w935
              tunnel: w931 -> [w943 _]
              tunnel: w934 -> [w944 _]
              tunnel: w933 -> [w957 _]
              tunnel: w932 -> [w950 _]
              tunnel: w928 -> [w949 _]
              tunnel: w927 -> [w940 _]
              frame False {
                n1197 = case "Save Raw File for offline processing" shown="True" w940 {
                  tunnel: w944 -> [_ w967]
                  tunnel: w943 -> [_ w966]
                  tunnel: w942 -> [w962 w965]
                  tunnel: [w962 w964] -> w941
                  frame False {
                  }
                  frame True {
                    n1198 = Unbundle By Name(w966) -> ("Start Position"=w971:dbl[], "StepWidth"=w970:dbl[], "Dimension"=w969:i32[])
                    n1199 = Unbundle By Name(w967) -> ("WriterCtrl"=w968:refnum<queue>)
                    n1200 = property on="Depth" class="DigNum (strict)"() -> ("Value"=w963:dbl)  [unwired: 2 in, 2 out]
                    n1201 = Bundle By Name(cluster=T77 {"Start Position"=[], "StepWidth"=[], "Dimension"=[], "SpecLength"=0} ("File Header"), "Start Position"=w971, "StepWidth"=w970, "Dimension"=w969, "SpecLength"=w963) -> (w972:T77)
                    n1202 = Bundle By Name(cluster=T68 {"State"=enum."SetHeader", "Params"=variant} ("element"), "Params"=w972) -> (w974:T68)
                    n1203 = Enqueue Element(queue=w968, element=w974, error in (no error)=w965) -> (error out=w964:errorcluster)  [unwired: 1 in, 2 out]
                  }
                }
                n1204 = property on="Depth" class="DigNum (strict)"() -> ("Value"=w938:dbl)  [unwired: 2 in, 2 out]
                n1205 = property on="Sample Rate" class="DigNum (strict)"() -> ("Value"=w939:dbl)  [unwired: 2 in, 2 out]
                n1206 = property on="Trigger Delay" class="DigNum (strict)"() -> ("Value"=w937:dbl)  [unwired: 2 in, 2 out]
                n1207 = Unbundle By Name(w949) -> ("HighSpeed"=w945:dbl, "RepRate (Hz)"=w946:dbl, "KeepStill(ms)"=w947:u32)  [unwired: 1 out]
                n1208 = Unbundle By Name(w943) -> ("Start Position"=w955:dbl[], "StepWidth"=w954:dbl[], "Dimension"=w953:i32[])
                n1209 = property on="Cali." class="Arr (strict)"() -> ("Value"=w952:dbl[])  [unwired: 2 in, 2 out]
                n1210 = Bundle By Name(cluster=T80 {"File Header"={"Start Position"=[], "StepWidth"=[], "Dimension"=[], "SpecLength"=0}, "ScanSpeed"=0.0, "HighSpeed"=0.0, "SampleRate"=0.0, "Rep.Rate (Hz)"=0.0, "TrigDelay"=0.0, "mzCali"=[], "KeepStill(ms)"=0, "SaveRaw"=FALSE} ("BeamProfiling_Params"), "File Header.SpecLength"=w938, "SampleRate"=w939, "TrigDelay"=w937, "mzCali"=w952, "SaveRaw"=w940, "File Header.Start Position"=w955, "File Header.StepWidth"=w954, "File Header.Dimension"=w953, "ScanSpeed"=w945, "HighSpeed"=w945, "Rep.Rate (Hz)"=w946, "KeepStill(ms)"=w947) -> (w951:T80)
                n1211 = Unbundle By Name(w944) -> ("Micos"=w958:refnum<queue>)
                n1212 = call "MeanderCtrl_Dynamic,StageRefs.vi"("QueuesRef"=w944, "MotionStageRefs"=w958, "AppsRef"=w957, "subprog_Ref"=w950, "Params."=w951, "Laser_Ctrl"=TRUE, "error in"=w941, "HighSpeed"=w945, "LowSpeed"=w945) -> ("error out"=w959:errorcluster)  [unwired: 5 in, 1 out]
                n1213 = property on="Record" class="Bool (strict)"(error in=w959, "Val(Sgnl)"=FALSE) -> (error out=w960:errorcluster)  [unwired: 1 in, 1 out]
              }
              frame True {
              }
            }
          }
          frame "DepthProfiling" {
            n1214 = global read "Position_Micos.vi" "Position(Micos)"() -> (w979:dbl[])
            n1215 = call "DepthProfile_Setup.vi"("RepRate (Hz)"=w977, "Start Position"=w979) -> ("Depth Profile Params."=w978:T96, "Canceled"=w985:bool, "Meander_Params."=w982:T77)  [unwired: 6 in, 1 out]
            n1216 = case shown="False" w985 {
              tunnel: w984 -> [w996 w1009]
              tunnel: [w999 w1009] -> w983
              tunnel: w982 -> [w1003 _]
              tunnel: w981 -> [w993 _]
              tunnel: w980 -> [w992 _]
              tunnel: w978 -> [w990 _]
              frame False {
                n1217 = Unbundle By Name(w1003) -> ("Start Position"=w1002:dbl[], "StepWidth"=w1001:dbl[], "Dimension"=w1000:i32[])
                n1218 = property on="Depth" class="DigNum (strict)"() -> ("Value"=w986:dbl)  [unwired: 2 in, 2 out]
                n1219 = Unbundle By Name(w993) -> ("WriterCtrl"=w994:refnum<queue>)
                n1220 = Bundle By Name(cluster=T77 {"Start Position"=[], "StepWidth"=[], "Dimension"=[], "SpecLength"=0} ("File Header"), "Start Position"=w1002, "StepWidth"=w1001, "Dimension"=w1000, "SpecLength"=w986) -> (w1004:T77)
                n1221 = Unbundle By Name(w990) -> ("SamplingPos."=w988:cluster{"x":dbl, "y":dbl, "z":dbl}[][], "HighSpeed"=w989:dbl, "KeepStill(ms)"=w987:u32)  [unwired: 1 out]
                n1222 = Bundle By Name(cluster=T68 {"State"=enum."SetHeader", "Params"=variant} ("element"), "Params"=w1004) -> (w1006:T68)
                n1223 = Enqueue Element(queue=w994, element=w1006, error in (no error)=w996) -> (error out=w997:errorcluster)  [unwired: 1 in, 2 out]
                n1224 = Unbundle By Name(w993) -> ("Micos"=w995:refnum<queue>)
                n1225 = call "MeanderCtrl_3d_StageRefs.vi"("QueuesRef"=w993, "MotionStageRefs"=w995, "AppsRef"=w992, "start/end points"=w988, "Laser_Ctrl"=TRUE, "error in"=w997, "HighSpeed"=w989, "ScanSpeed"=w989, "KeepStill"=w987) -> ("error out"=w998:errorcluster)  [unwired: 4 in, 2 out]
                n1226 = property on="Record" class="Bool (strict)"(error in=w998, "Val(Sgnl)"=FALSE) -> (error out=w999:errorcluster)  [unwired: 1 in, 1 out]
              }
              frame True {
              }
            }
          }
          frame "Set_2PulseDelay" {
            n1227 = Unbundle By Name(w1028) -> ("ESP300"=w1026:refnum<queue>)
            n1228 = Bundle By Name(cluster=T81 {"MotionStageRefs"=refnum, "Axis#"=0, "Delay(ps)"=0.0, "ZeroDelay_Offset"=0.0} ("Params."), "MotionStageRefs"=w1026, "Delay(ps)"="DP_Delay (ps)", "ZeroDelay_Offset"="ZeroDelayPos") -> (w1025:T81)
            n1229 = control-ref of="Destination(ESP)"() -> (w1019:refnum<vi>)
            n1230 = property class="Arr (strict)"(reference=w1019) -> (reference out=w1018:refnum<vi>, error out=w1011:errorcluster, "Value"=w1014:dbl[])  [unwired: 1 in]
            n1231 = call "Set_DoublePulse_Delay.vi"("error in"=w1023, "WaitForReady"=TRUE, "InputParams."=w1025) -> ("error out"=w1020:errorcluster, "DP_StagePos."=w1015:variant)  [unwired: 7 in]
            n1232 = Variant To Data(error in=w1011, type=w1014, Variant=w1015) -> (data=w1013:dbl[], error out=w1012:errorcluster)
            n1233 = Replace Array Subset(array=w1014, new element=w1013, index=0) -> (w1017:dbl[])
            n1234 = property class="Arr (strict)"(reference=w1018, error in=w1012, "Value"=w1017) -> (error out=w1010:errorcluster)  [unwired: 1 out]
            n1235 = call <vilib>:"Clear Errors.vi"("error in (no error)"=w1010) -> ()  [unwired: 6 in, 1 out]
          }
          frame "DelayScan" {
            n1236 = local read "ZeroDelayPos"() -> (w1030:dbl)
            n1237 = global read "Position_Micos.vi" "Position(Micos)"() -> (w1034:dbl[])
            n1238 = Unbundle By Name(w1033) -> ("ESP300"=w1032:refnum<queue>)
            n1239 = call "DoublePulse_Delay_Scan_Setup.vi"("Rep. Rate (Hz)"=w1029, "ZeroDelayPos"=w1030, "Start Position"=w1034, "ESP300"=w1032) -> ("Laser_Ctrl"=w1039:bool, "start/end points"=w1040:cluster{dbl, dbl, dbl}[][], "Canceled"=w1041:bool, "SecondaryParams"=w1031:variant[], "ImageParameter"=w1036:T94)  [unwired: 3 in]
            n1240 = case shown="False" w1041 {
              tunnel: w1040 -> [w1065 _]
              tunnel: w1038 -> [w1052 w1066]
              tunnel: w1039 -> [w1064 _]
              tunnel: [w1055 w1066] -> w1037
              tunnel: w1036 -> [w1048 _]
              tunnel: w1033 -> [w1046 _]
              tunnel: w1035 -> [w1050 _]
              tunnel: w1031 -> [w1043 _]
              frame False {
                n1241 = Unbundle By Name(w1048) -> ("ScanSpeed"=w1047:dbl)
                n1242 = local read "Velocity(Micos)"() -> (w1049:dbl)
                n1243 = Unbundle By Name(w1048) -> ("Start Position"=w1058:dbl[], "StepWidth"=w1057:dbl[], "Dimension"=w1056:i32[])
                n1244 = property on="Depth" class="DigNum (strict)"() -> ("Value"=w1042:dbl)  [unwired: 2 in, 2 out]
                n1245 = Unbundle By Name(w1046) -> ("WriterCtrl"=w1051:refnum<queue>)
                n1246 = Bundle By Name(cluster=T77 {"Start Position"=[], "StepWidth"=[], "Dimension"=[], "SpecLength"=0} ("File Header"), "Start Position"=w1058, "StepWidth"=w1057, "Dimension"=w1056, "SpecLength"=w1042) -> (w1059:T77)
                n1247 = Bundle By Name(cluster=T68 {"State"=enum."SetHeader", "Params"=variant} ("element"), "Params"=w1059) -> (w1061:T68)
                n1248 = Enqueue Element(queue=w1051, element=w1061, error in (no error)=w1052) -> (error out=w1053:errorcluster)  [unwired: 1 in, 2 out]
                n1249 = Unbundle By Name(w1046) -> ("Micos"=w1045:refnum<queue>)
                n1250 = vi-ref "Set_DoublePulse_Delay.vi"() -> (w1044:refnum<vi>)
                n1251 = call "MeanderCtrl_3d_StageRefs.vi"("QueuesRef"=w1046, "MotionStageRefs"=w1045, "AppsRef"=w1050, "SecondaryVI_Ref"=w1044, "SecondaryParams"=w1043, "start/end points"=w1065, "Laser_Ctrl"=w1064, "error in"=w1053, "HighSpeed"=w1049, "ScanSpeed"=w1047) -> ("error out"=w1054:errorcluster)  [unwired: 3 in, 2 out]
                n1252 = property on="Record" class="Bool (strict)"(error in=w1054, "Val(Sgnl)"=FALSE) -> (error out=w1055:errorcluster)  [unwired: 1 in, 1 out]
              }
              frame True {
              }
            }
          }
          frame "Save Settings" {
            n1253 = feedback #9(path "" ("selected path")) -> (w1070:path)
            n1254 = Strip Path(path=w1070) -> (stripped path=w1072:path, name=w1071:string)
            n1255 = call "File Dialog4"("start path"=w1072, "default name"=w1071, "pattern (all files)"="*.conf.json", "pattern label"="Json Configuration Files") -> ("selected path"=w1074:path, "cancelled"=w1075:bool)  [unwired: 8 in, 2 out]
            n1256 = feedback-in #9(w1074) -> ()
            n1257 = case shown="False" w1075 {
              tunnel: w1067 -> [w1076 _]
              frame False {
                n1258 = call "SaveConfigs_toFile.vi"("Configuration"=w1076) -> ()  [unwired: 11 in]
              }
              frame True {
              }
            }
          }
          frame "EnergyCalibration" {
            n1259 = Unbundle By Name(w1078) -> ("ESP300"=w1077:refnum<queue>)
            n1260 = call "Acquire_EnergyCalibrationCurve.vi"("Queue in"=w1077) -> ()  [unwired: 10 in, 1 out]
          }
          frame "Quit" {
            n1261 = Unbundle By Name(w1112) -> ("SRS DG535"=w1099:refnum<queue>, "BNC"=w1111:refnum<queue>, "Feedback"=w1110:refnum<queue>, "ESP300"=w1109:refnum<queue>, "Micos"=w1108:refnum<queue>, "SDG_ii"=w1107:refnum<queue>, "EPM2000"=w1089:refnum<queue>, "NI-USB_DAQmx"=w1106:refnum<queue>, "MainDAQCoreQueue"=w1105:refnum<queue>, "WriterCtrl"=w1104:refnum<queue>)  [unwired: 1 out]
            n1262 = Release Queue(queue=w1122, error in (no error)=w1123) -> ()  [unwired: 1 in, 3 out]
            n1263 = Enqueue Element(queue=w1104, element=T68 {"State"=enum."QuitProg.", "Params"=variant}) -> ()  [unwired: 2 in, 3 out]
            n1264 = Enqueue Element(queue=w1105, element=T60 {"DWF States"=enum."Quit", "Variant"=variant}) -> ()  [unwired: 2 in, 3 out]
            n1265 = global write "QuitProg.vi" "QuitProg."(TRUE ("QuitProg.")) -> ()
            n1266 = Enqueue Element(queue=w1106, element=T85 {"State"=enum."Quit", "Para."=variant}) -> ()  [unwired: 2 in, 3 out]
            n1267 = Enqueue Element(queue=w1089, element=T83 {"State"=enum."Close", "Parameter"=0.0}) -> (queue out=w1100:refnum<queue>)  [unwired: 2 in, 2 out]
            n1268 = Enqueue Element(queue=w1100, element=T83 {"State"=enum."Quit", "Parameter"=0.0}) -> ()  [unwired: 2 in, 3 out]
            n1269 = Enqueue Element(queue=w1107, element=T70 {"State"=enum."Tun OFF", "Parameter"=0.0}) -> (queue out=w1114:refnum<queue>)  [unwired: 2 in, 2 out]
            n1270 = Enqueue Element(queue=w1114, element=T70 {"State"=enum."Close", "Parameter"=0.0}) -> (queue out=w1102:refnum<queue>)  [unwired: 2 in, 2 out]
            n1271 = Enqueue Element(queue=w1108, element=T74 {"State"=enum."STOP", "Params."=variant}) -> (queue out=w1083:refnum<queue>)  [unwired: 2 in, 2 out]
            n1272 = Enqueue Element(queue=w1099, element=T82 {"State"=enum."Stop", "Para."=variant}) -> (queue out=w1095:refnum<queue>, error out=w1088:errorcluster)  [unwired: 2 in, 1 out]
            n1273 = Enqueue Element(queue=w1102, element=T70 {"State"=enum."Quit", "Parameter"=0.0}) -> ()  [unwired: 2 in, 3 out]
            n1274 = Enqueue Element(queue=w1111, element=T84 {"State"=enum."Close", "Para."=variant}) -> (queue out=w1117:refnum<queue>)  [unwired: 2 in, 2 out]
            n1275 = Enqueue Element(queue=w1117, element=T84 {"State"=enum."Quit", "Para."=variant}) -> ()  [unwired: 2 in, 3 out]
            n1276 = Bundle By Name(cluster=T74 {"State"=enum."MotorEnable(1)", "Params."=variant} ("element"), "Params."=FALSE) -> (w1081:T74)
            n1277 = Enqueue Element(queue=w1095, element=T82 {"State"=enum."Close", "Para."=variant}, error in (no error)=w1088) -> (queue out=w1094:refnum<queue>, error out=w1087:errorcluster)  [unwired: 1 in, 1 out]
            n1278 = Enqueue Element(queue=w1083, element=w1081) -> (queue out=w1082:refnum<queue>)  [unwired: 2 in, 2 out]
            n1279 = Enqueue Element(queue=w1082, element=T74 {"State"=enum."Close", "Params."=variant}) -> (queue out=w1090:refnum<queue>)  [unwired: 2 in, 2 out]
            n1280 = Enqueue Element(queue=w1094, element=T82 {"State"=enum."Quit", "Para."=variant}, error in (no error)=w1087) -> (error out=w1086:errorcluster)  [unwired: 1 in, 2 out]
            n1281 = Enqueue Element(queue=w1090, element=T74 {"State"=enum."Quit", "Params."=variant}) -> ()  [unwired: 2 in, 3 out]
            n1282 = call <vilib>:"Clear Errors.vi"("error in (no error)"=w1086) -> ()  [unwired: 6 in, 1 out]
            n1283 = Enqueue Element(queue=w1109, element=T74 {"State"=enum."Quit", "Params."=variant}) -> ()  [unwired: 2 in, 3 out]
            n1284 = Release Queue(queue=w1110) -> ()  [unwired: 2 in, 3 out]
          }
          frame "Check_AppsLock" {
            # "No need"
          }
          frame Default {
            n1285 = property on="Property Node" class="Str"(reference=w1126) -> (reference out=w1129:refnum<vi>, "Value"=w1130:string)  [unwired: 1 in, 1 out]
            n1286 = Format Into String(format string="%s", initial string="\nUnsupported function:", w1133) -> (resulting string=w1128:string)  [unwired: 1 in, 1 out]
            n1287 = Concatenate Strings(w1130, w1128) -> (w1127:string)
            n1288 = property on="Property Node" class="Str"(reference=w1129, "Value"=w1127) -> ()  [unwired: 1 in, 2 out]
          }
        }
        n1289 = call <userlib>:"ErrorLog.vi"("error in (no error)"=w570) -> ("error out"=w562:errorcluster)  [unwired: 10 in]
        n1290 = call <vilib>:"Release Semaphore.vi"("error in (no error)"=w562, "semaphore"=w563) -> ("error out"=w561:errorcluster)  [unwired: 4 in, 1 out]
      }
      n1291 = Merge Errors(w223, w224, w225, w226, w227, w228, w229) -> (w222:errorcluster)
      n1292 = Merge Errors(w165, w169, w168) -> (w164:errorcluster)
      n1293 = Release Queue(queue=w171, error in (no error)=w164) -> (error out=w172:errorcluster)  [unwired: 1 in, 2 out]
      n1294 = Release Queue(queue=w173, error in (no error)=w172) -> (error out=w166:errorcluster)  [unwired: 1 in, 2 out]
      n1295 = Release Queue(queue=w162, error in (no error)=w166) -> (error out=w167:errorcluster)  [unwired: 1 in, 2 out]
      n1296 = Release Queue(queue=w163, error in (no error)=w167) -> (error out=w170:errorcluster)  [unwired: 1 in, 2 out]
      n1297 = Merge Errors(w222, w230, w170) -> (w221:errorcluster)
    }
  }
  n1298 = Release Queue(queue=w71, error in (no error)=w70) -> (error out=w54:errorcluster)  [unwired: 1 in, 2 out]
  n1299 = Release Queue(queue=w68, error in (no error)=w54) -> (error out=w69:errorcluster)  [unwired: 1 in, 2 out]
  n1300 = Release Queue(queue=w67, error in (no error)=w69) -> (error out=w65:errorcluster)  [unwired: 1 in, 2 out]
  n1301 = Release Queue(queue=w66, error in (no error)=w65) -> (error out=w63:errorcluster)  [unwired: 1 in, 2 out]
  n1302 = Release Queue(queue=w64, error in (no error)=w63) -> (error out=w60:errorcluster)  [unwired: 1 in, 2 out]
  n1303 = Release Queue(queue=w61, error in (no error)=w60) -> (error out=w59:errorcluster)  [unwired: 1 in, 2 out]
  n1304 = Release Queue(queue=w62, error in (no error)=w59) -> (error out=w58:errorcluster)  [unwired: 1 in, 2 out]
  n1305 = call <vilib>:"General Error Handler.vi"("type of dialog (OK msg:1)"=w57, "error in (no error)"=w58, "[exception action] (none:0)"=w56, "[exception code]"=1) -> ()  [unwired: 7 in, 5 out]
